vi "16Channels_savedata.vi"() -> ()   [LabVIEW 2020]
uses:
  Energy Meter/Labview Driver for S-Link (VISA).llb/Factor.ctl
  <vilib>/Utility/file.llb/Write Delimited Spreadsheet (string).vi
  <vilib>/Utility/file.llb/Write To Spreadsheet File (string).vi
  <vilib>/Utility/file.llb/Read Delimited Spreadsheet (DBL).vi
panel:
  out "Second Window Output":T1={"Status"=TRUE, "Indicator Color"=[], "Time"="", "Energy Value"=0.0, "Spectrometer Output"={array[3648 elements], array[3648 elements]}, "Energy stat"=TRUE}
  out "Program Status:":string="Program Stopped!"
  in  "Send 8":bool
  in  "Send 7":bool
  in  "Send 6":bool
  in  "Com Port 8":refnum<visa-resource-name>="COM27"
  in  "Com Port 7":refnum<visa-resource-name>="COM25"
  in  "Com Port 6":refnum<visa-resource-name>="COM23"
  in  "Save Next shot to File?":bool=TRUE
  in  "Com Port 5":refnum<visa-resource-name>="COM24"
  in  "Send 5":bool
  in  "Tab Control":T2(tab)=enum."Plots"
  out "Scale 8":dbl format="%.0e"
  out "Ch 08 Status":bool
  in  "Scale UP 8":bool
  in  "Scale Down 8":bool
  out "Measure 8":dbl format="%.3e"
  out "Scale 1":dbl=0.00031622776601683794 format="%.0e"
  out "Scale 2":dbl=0.00031622776601683794 format="%.0e"
  out "Ch 02 Status":bool
  out "Ch 01 Status":bool
  out "Scale 3":dbl=0.03162277660168379 format="%.0e"
  out "Scale 4":dbl=0.03162277660168379 format="%.0e"
  out "Ch 04 Status":bool
  out "Ch 03 Status":bool
  in  "Scale Down":bool
  in  "Scale UP 2":bool
  in  "Scale Down 2":bool
  in  "Scale UP":bool
  out "Measure 2":dbl format="%.3e"
  out "Measure 3":dbl format="%.3e"
  out "Measure 4":dbl format="%.3e"
  in  "Scale UP 3":bool
  in  "Scale Down 3":bool
  in  "Scale UP 4":bool
  in  "Scale Down 4":bool
  out "Scale 5":dbl=0.03162277660168379 format="%.0e"
  out "Scale 6":dbl=0.03162277660168379 format="%.0e"
  out "Ch 06 Status":bool
  out "Ch 05 Status":bool
  out "Measure 5":dbl format="%.3e"
  out "Measure 6":dbl format="%.3e"
  in  "Scale UP 5":bool
  in  "Scale Down 5":bool
  in  "Scale UP 6":bool
  in  "Scale Down 6":bool
  out "Measure 1":dbl format="%.3e"
  out "Scale 7":dbl format="%.0e"
  out "Ch 07 Status":bool
  in  "Scale UP 7":bool
  in  "Scale Down 7":bool
  out "Measure 7":dbl format="%.3e"
  in  "Scale UP 9":bool
  in  "Scale Down 9":bool
  in  "Scale UP 10":bool
  in  "Scale Down 10":bool
  out "Scale 9":dbl=0.03162277660168379 format="%.0e"
  out "Scale 10":dbl=0.03162277660168379 format="%.0e"
  out "Ch 09 Status":bool
  out "Ch 10 Status":bool
  out "Measure 9":dbl format="%.3e"
  out "Measure 10":dbl format="%.3e"
  out "Measure 11":dbl=0.00198 format="%.3e"
  out "Measure 12":dbl=0.001829 format="%.3e"
  in  "Scale UP 11":bool
  in  "Scale Down 11":bool
  in  "Scale UP 12":bool
  in  "Scale Down 12":bool
  out "Scale 11":dbl=0.0031622776601683794 format="%.0e"
  out "Scale 12":dbl=0.03162277660168379 format="%.0e"
  out "Ch 11 Status":bool
  out "Ch 12 Status":bool
  out "Scale 13":dbl format="%.0e"
  out "Scale 14":dbl format="%.0e"
  out "Ch 13 Status":bool
  out "Ch 14 Status":bool
  out "Scale 15":dbl=0.03162277660168379 format="%.0e"
  out "Scale 16":dbl=0.03162277660168379 format="%.0e"
  out "Ch 15 Status":bool
  out "Ch 16 Status":bool
  in  "Scale UP 13":bool
  in  "Scale Down 13":bool
  in  "Scale UP 14":bool
  in  "Scale Down 14":bool
  out "Measure 13":dbl=0.0004823 format="%.3e"
  out "Measure 14":dbl=1.44e-05 format="%.3e"
  in  "Scale UP 15":bool
  in  "Scale Down 15":bool
  in  "Scale UP 16":bool
  in  "Scale Down 16":bool
  out "Measure 15":dbl format="%.3e"
  out "Measure 16":dbl format="%.3e"
  out "Ch 1":dbl(graph)
  out "Ch 2":dbl(graph)
  out "Ch 3":dbl(graph)
  out "Ch 4":dbl(graph)
  out "Ch 5":dbl(graph)
  out "Ch 6":dbl(graph)=0.01011366
  out "Ch 7":dbl(graph)=0.0052277218000000006
  out "Ch 8":dbl(graph)=0.007128125500000001
  out "Ch 9":dbl(graph)=1.049625
  out "Ch 10":dbl(graph)=11.3826
  out "Ch 11":dbl(graph)=178.2
  out "Ch 12":dbl(graph)=0.001829
  out "Ch 13":dbl(graph)=591.068296
  out "Ch 14":dbl(graph)=1.44
  out "Ch 15":dbl(graph)
  out "Ch 16":dbl(graph)
  out "Ch 01 Status 2":bool=TRUE
  out "Ch 03 Status 2":bool=TRUE
  out "Ch 06 Status 2":bool=TRUE
  out "Ch 07 Status 2":bool=TRUE
  out "Ch 10 Status 2":bool=TRUE
  out "Ch 02 Status 2":bool=TRUE
  out "Ch 04 Status 2":bool=TRUE
  out "Ch 05 Status 2":bool=TRUE
  out "Ch 08 Status 2":bool=TRUE
  out "Ch 09 Status 2":bool=TRUE
  out "Ch 11 Status 2":bool=TRUE
  out "Ch 13 Status 2":bool=TRUE
  out "Ch 15 Status 2":bool=TRUE
  out "Ch 12 Status 2":bool=TRUE
  out "Ch 14 Status 2":bool=TRUE
  out "Ch 16 Status 2":bool=TRUE
  in  "Ch9 ON/OFF":bool=TRUE
  in  "Ch10 ON/OFF":bool=TRUE
  in  "Ch11 ON/OFF":bool=TRUE
  in  "Ch12 ON/OFF":bool=TRUE
  in  "Ch13 ON/OFF":bool=TRUE
  in  "Ch14 ON/OFF":bool=TRUE
  in  "C15 ON/OFF":bool=TRUE
  in  "Ch16 ON/OFF":bool=TRUE
  in  "Ch1 ON/OFF":bool=TRUE
  in  "Ch2 ON/OFF":bool=TRUE
  in  "Ch4 ON/OFF":bool=TRUE
  in  "Ch3 ON/OFF":bool=TRUE
  in  "Ch6 ON/OFF":bool=TRUE
  in  "Ch5 ON/OFF":bool=TRUE
  in  "Ch8 ON/OFF":bool=TRUE
  in  "Ch7 ON/OFF":bool=TRUE
  out "Trigger ch 10":bool=TRUE
  out "Trigger ch 9":bool=TRUE
  out "Trigger ch 8":bool=TRUE
  out "Trigger ch 7":bool
  out "Trigger ch 6":bool=TRUE
  out "Trigger ch 5":bool=TRUE
  out "Trigger ch 4":bool=TRUE
  out "Trigger ch 3":bool=TRUE
  out "Trigger ch 2":bool=TRUE
  out "Trigger ch 1":bool=TRUE
  in  "Threshold Green 1":dbl=9.0
  in  "Threshold Green 2":dbl=6.0
  out "Wavelength 7":i16
  out "Wavelength 6":i16=532
  out "Wavelength 5":i16=532
  out "Wavelength 4":i16=532
  out "Wavelength 3":i16=532
  out "Wavelength 2":i16=1064
  out "Wavelength 1":i16=1064
  out "Wavelength 8":i16
  in  "Factor 7":T3=642.7 caption="Factor1" format="%#_13g"
  in  "Factor 6":T3=470.0 caption="Factor1" format="%#_13g"
  in  "Factor 5":T3=470.0 caption="Factor1" format="%#_13g"
  in  "Factor 4":T3=486.0 caption="Factor1" format="%#_13g"
  in  "Factor 3":T3=3108.0 caption="Factor1" format="%#_13g"
  in  "Factor 2":T3=12595.0 caption="Factor1" format="%#_13g"
  in  "Factor 1":T3=8156.0 caption="Factor1" format="%#_13g"
  in  "Factor 8":T3=789.82 caption="Factor1" format="%#_13g"
  in  "Threshold IR 1":dbl=2.3
  in  "Threshold IR 2":dbl=2.0
  in  "Factor 9":T3=622.2 caption="Factor1" format="%#_13g"
  in  "Factor 10":T3=777.5 caption="Factor1" format="%#_13g"
  out "Wavelength 9":i16=532
  out "Wavelength 10":i16=532
  in  "Factor 11":T3=90.0 caption="Factor1" format="%#_13g"
  in  "Factor 12":T3=1.0 caption="Factor1" format="%#_13g"
  in  "Threshold 2nd stage 1":dbl=0.16
  in  "Threshold 2nd stage 2":dbl=0.12
  in  "Threshold 3rd stage 1":dbl=2.5
  in  "Threshold 3rd stage 2":dbl=2.0
  out "Trigger ch 11":bool
  out "Trigger ch 12":bool=TRUE
  out "Wavelength 11":i16=800
  out "Wavelength 12":i16=800
  out "Wavelength 13":i16
  out "Wavelength 14":i16
  out "Trigger ch 13":bool
  out "Trigger ch 14":bool
  out "Wavelength 15":i16=800
  out "Wavelength 16":i16=800
  out "Trigger ch 15":bool=TRUE
  out "Trigger ch 16":bool=TRUE
  in  "Threshold 1st stage 1":dbl=0.0013 format="%#_2e"
  in  "Threshold 1st stage 2":dbl=0.001 format="%#_2e"
  in  "Threshold quantaray stage 1":dbl=0.62
  in  "Threshold quantaray stage 2":dbl=0.58
  in  "Factor 13":T3=1225.52 caption="Factor1" format="%#_13g"
  in  "Factor 14":T3=100.0 caption="Factor1" format="%#_13g"
  in  "Factor 15":T3=1.0 caption="Factor1" format="%#_13g"
  in  "Factor a":T3=43958.0 caption="Factor1" format="%#_13g"
  in  "Threshold 4th stage 2":dbl=7.0
  in  "Threshold 4th stage 1":dbl=9.0
  in  "Threshold 5th stage 2":dbl
  in  "Threshold 5th stage 1":dbl
  in  "Factor b":T3=10193.0 caption="Factor1" format="%#_13g"
  in  "Factor c":T3=-0.3437 caption="Factor1" format="%#_13g"
  out "Path Spectrometer Folder":path=path "D:/Spectrometer/20220114"
  out "Path Spectrometer Data Old":path
  in  "Path Spectrometer Base":path=path "D:/Spectrometer"
  in  "Base Path":path=path "D:/Energy Meter"
  out "Folder":path=path "D:/Energy Meter/20220114"
  in  "Path SLAB #10":path=path "D:/Energy Meter/20220114/SLAB10.csv"
  in  "Path SLAB #9":path=path "D:/Energy Meter/20220114/SLAB9.csv"
  in  "Path SLAB #8":path=path "D:/Energy Meter/20220114/SLAB8.csv"
  in  "Path SLAB #7":path=path "D:/Energy Meter/20220114/SLAB7.csv"
  in  "Path SLAB #5":path=path "D:/Energy Meter/20220114/SLAB5.csv"
  in  "Path SLAB #4":path=path "D:/Energy Meter/20220114/SLAB4.csv"
  in  "Path SLAB #3":path=path "D:/Energy Meter/20220114/SLAB3.csv"
  in  "Path SLAB #2":path=path "D:/Energy Meter/20220114/SLAB2.csv"
  in  "Path Frontend #2":path=path "D:/Energy Meter/20220114/FrontEnd2.csv"
  in  "Path Frontend #1":path=path "D:/Energy Meter/20220114/FrontEnd1.csv"
  out "Date":string="20220114"
  out "Time":string="11:33:50.900"
  in  "Path 1st stage":path=path "D:/Energy Meter/20220114/1st_stage.csv"
  in  "Path 2nd stage":path=path "D:/Energy Meter/20220114/2nd_stage.csv"
  in  "Path 3rd stage":path=path "D:/Energy Meter/20220114/3rd_stage.csv"
  in  "Path 4th stage":path=path "D:/Energy Meter/20220114/4th_stage.csv"
  in  "Path 5th stage":path=path "D:/Energy Meter/20220114/5th_stage.csv"
  in  "Path quanta ray":path=path "D:/Energy Meter/20220114/quanta-ray.csv"
  in  "Send 4":bool
  in  "Com Port 4":refnum<visa-resource-name>="COM26"
  in  "Command":i32(ring)=22 items=["*RST", "*VER", "*CA1", "*CA2", "*SS1", "*SS2", "*SU1", "*SU2", "*SD1", "*SD2", "*CS1", "*CS2", "*AT1", "*AT2", "*AN1", "*AN2", "*PW1", "*PW2", "*TL1", "*TL2", "*ST1", "*ST2", "*ET1", "*ET2", "*EM1", "*EM2", "*SC1", "*SC2"]
  in  "Option":string="0"
  in  "Send 3":bool
  in  "Com Port 3":refnum<visa-resource-name>="COM20"
  in  "Send 2":bool
  in  "Stop Application":bool
  in  "Send":bool
  in  "Com Port 2":refnum<visa-resource-name>="COM22"
  in  "Com Port 1":refnum<visa-resource-name>="COM21"
  # "FrontEnd 1"
  # "SLAB 7"
  # "Quanta-Ray"
  # "FrontEnd 2"
  # "SLAB 9"
  # "1st Stage"
  # "SLAB 2"
  # "SLAB 10"
  # "4th Stage"
  # "SLAB 4"
  # "SLAB 8"
  # "5th Stage"
  # "SLAB 5"
  # "2nd Stage"
  # "SLAB 3"
  # "3rd Stage"
  # "FrontEnd #1"
  # "J"
  # "FrontEnd #2"
  # "J"
  # "Quanta-Ray"
  # "mJ"
  # "1st Stage"
  # "mJ"
  # "SLAB #2"
  # "SLAB #4"
  # "2nd Stage"
  # "3rd Stage"
  # "J"
  # "J"
  # "mJ"
  # "J"
  # "SLAB #3"
  # "SLAB #5"
  # "4th Stage"
  # "5th Stage"
  # "J"
  # "J"
  # "J"
  # "J"
  # "SLAB #7"
  # "SLAB #9"
  # "J"
  # "J"
  # "SLAB #8"
  # "SLAB #10"
  # "J"
  # "J"
  # "External\nTrigger"
  # "Wavelength"
  # "Energy Factor"
  # "Threshold 1\n(Warning)"
  # "Threshold 2\n(Bad)"
  # "Channel 01"
  # "IR"
  # "J"
  # "Com Port 1"
  # "Channel 02"
  # "Green"
  # "J"
  # "Channel 03"
  # "1st Stage"
  # "J"
  # "Com Port 2"
  # "Channel 04"
  # "2nd Stage"
  # "J"
  # "Channel 05"
  # "3rd Stage"
  # "J"
  # "Com Port 3"
  # "4th Stage"
  # "J"
  # "Channel 06"
  # "5th Stage"
  # "J"
  # "Channel 07"
  # "Com Port 4"
  # "Quanta-Ray"
  # "J"
  # "MUST USE THE FOLLOWING COMPORT SETTING! Otherwise the app will not save to proper files\n\nCom Port 1: COM21\nCom Port 2: COM22\nCom Port 3: COM20\nCom Port 4: COM26\nCom Port 5: COM24\nCom Port 6: COM23\nCom Port 7: COM25\nCom Port 8: COM27\n\nCOM20: Ch1- SLAB 5  Ch2 - SLAB 3  \nCOM21: Ch1- FrontEnd 1  Ch2- FrontEnd 2\nCOM22: Ch1- SLAB 2  Ch2 - SLAB 4\nCOM24: Ch1 - SLAB 10   Ch2 - SLAB 8\nCOM26: Ch1 - SLAB 7   Ch2 -SLAB 9\nCOM23: Ch1 - 2nd Stage  Ch2 - 3rd Stage\nCOM25: Ch1 - Quantaray  Ch2 - 1st Stage\nCOM27: Ch1 - 4th Stage  Ch2 - 5th Stage"
  # "Channel 08"
  # "Channel 09"
  # "Activate Channels"
  # "Com Port 5"
  # "Channel 10"
  # "Need to restart to change the status!"
  # "Ch09"
  # "Ch01"
  # "Ch09: SLAB #10\n\nCh10: SLAB #8\n\nCh11: 2nd Stage\n\nCh12: 3rd Stage\n\nCh13: Quanta-Ray\n\nCh14: 1st Stage\n\nCh15: 4th Stage\n\nCh16: 5th Stage"
  # "Ch01: FrontEnd #1 \n\nCh02: FrontEnd #2\n\nCh03: SLAB #2\n\nCh04: SLAB #4\n\nCh05: SLAB #5\n\nCh06: SLAB #3\n\nCh07: SLAB #7\n\nCh08: SLAB #9"
  # "OFF"
  # "ON"
  # "OFF"
  # "ON"
  # "Channel 11"
  # "Com Port 6"
  # "Ch10"
  # "Ch02"
  # "OFF"
  # "ON"
  # "OFF"
  # "ON"
  # "Channel 12"
  # "Ch11"
  # "Ch03"
  # "OFF"
  # "ON"
  # "OFF"
  # "ON"
  # "Channel 13"
  # "Ch12"
  # "Ch04"
  # "OFF"
  # "ON"
  # "OFF"
  # "ON"
  # "Com Port 7"
  # "Channel 14"
  # "Ch13"
  # "Ch05"
  # "OFF"
  # "ON"
  # "OFF"
  # "ON"
  # "Ch14"
  # "Channel 15"
  # "Ch06"
  # "OFF"
  # "ON"
  # "OFF"
  # "ON"
  # "Com Port 8"
  # "Ch15"
  # "Ch07"
  # "Channel 16"
  # "a"
  # "OFF"
  # "ON"
  # "OFF"
  # "ON"
  # "b"
  # "Ch16"
  # "Ch08"
  # "OFF"
  # "ON"
  # "OFF"
  # "ON"
  # "Polynominal Factor: ax^2+bx+c"
  # "c"
  # "Change base path before running the program!"
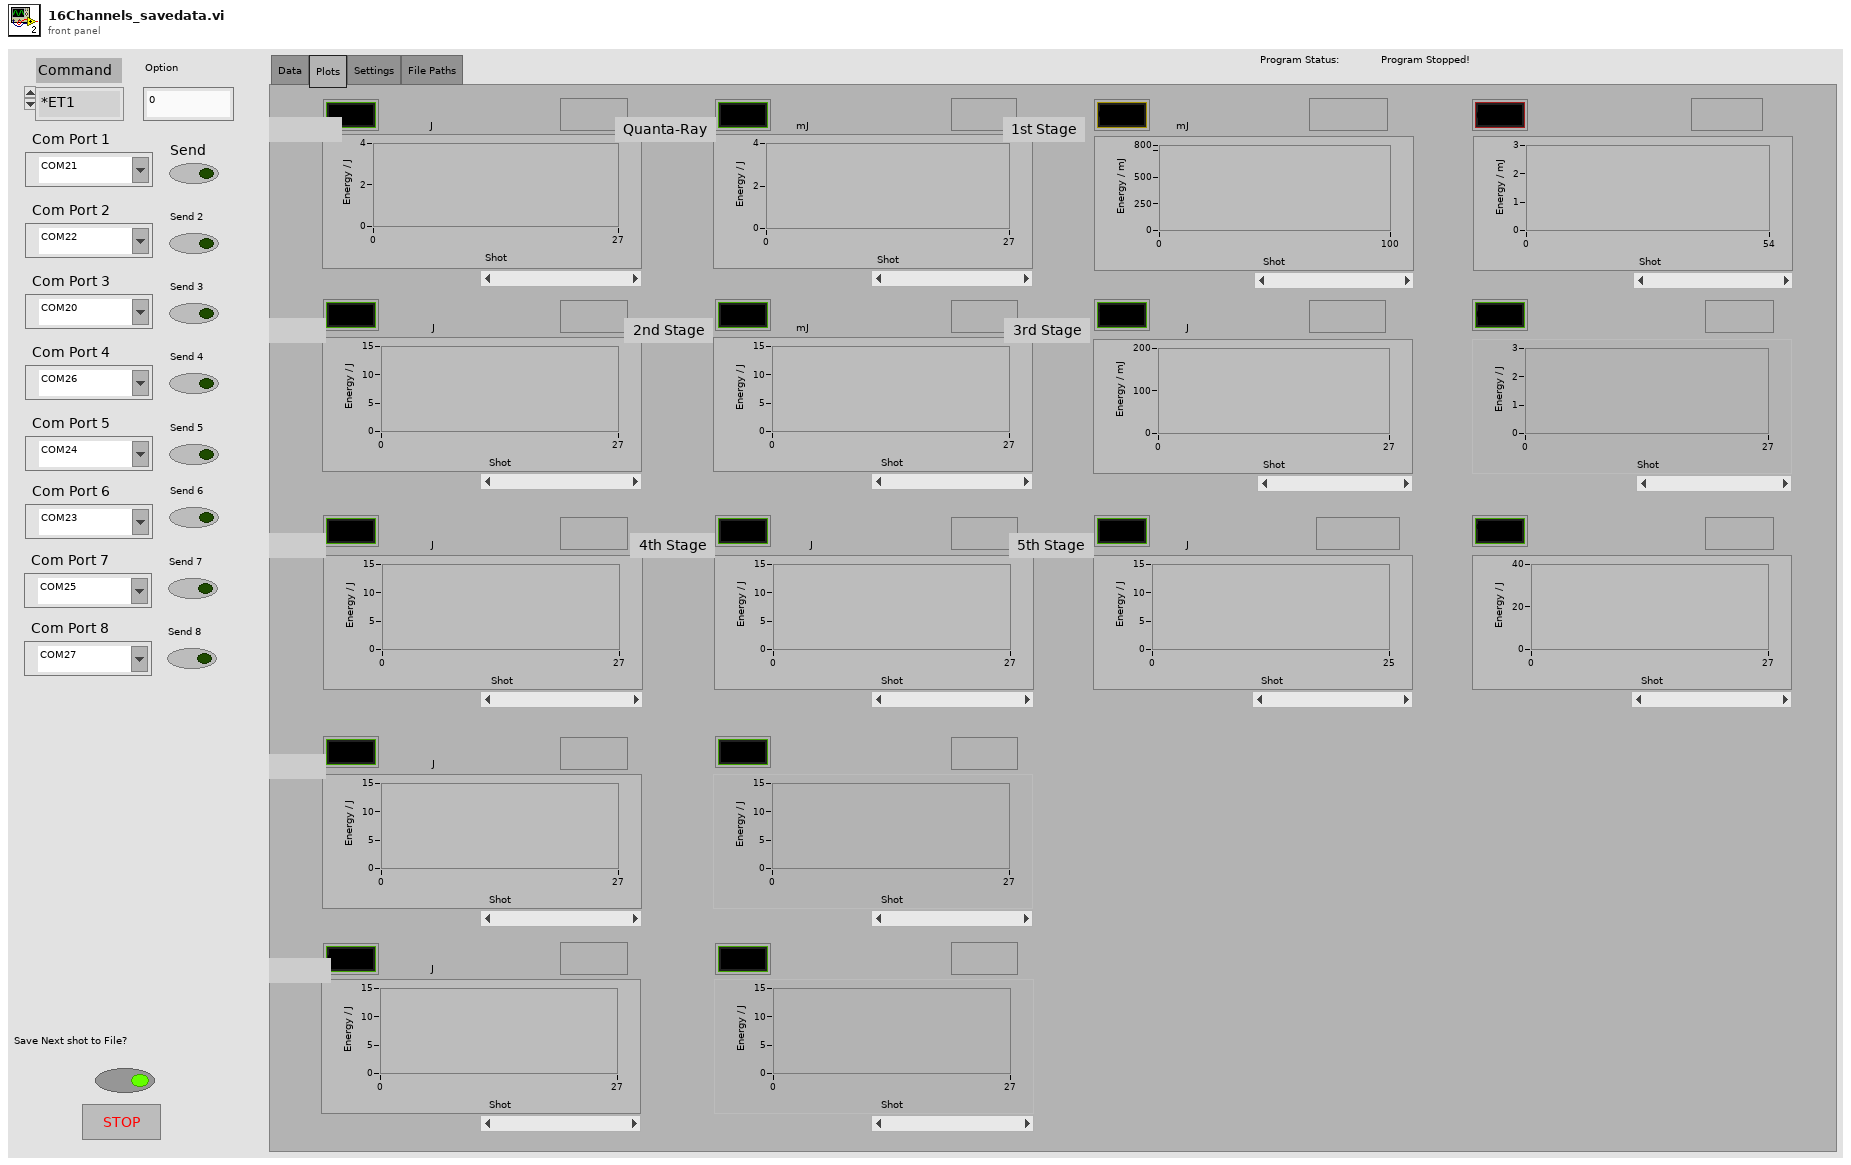
[diagram p1: front panel]
types:
  T1 = cluster{"Status":bool, "Indicator Color":cluster{u32, u32}[], "Time":string, "Energy Value":dbl, "Spectrometer Output":cluster{dbl[], dbl[]}, "Energy stat":bool}
  T2 = enum32{"Data", "Plots", "Settings", "File Paths"}
  T3 = typedef "Factor.ctl" = dbl
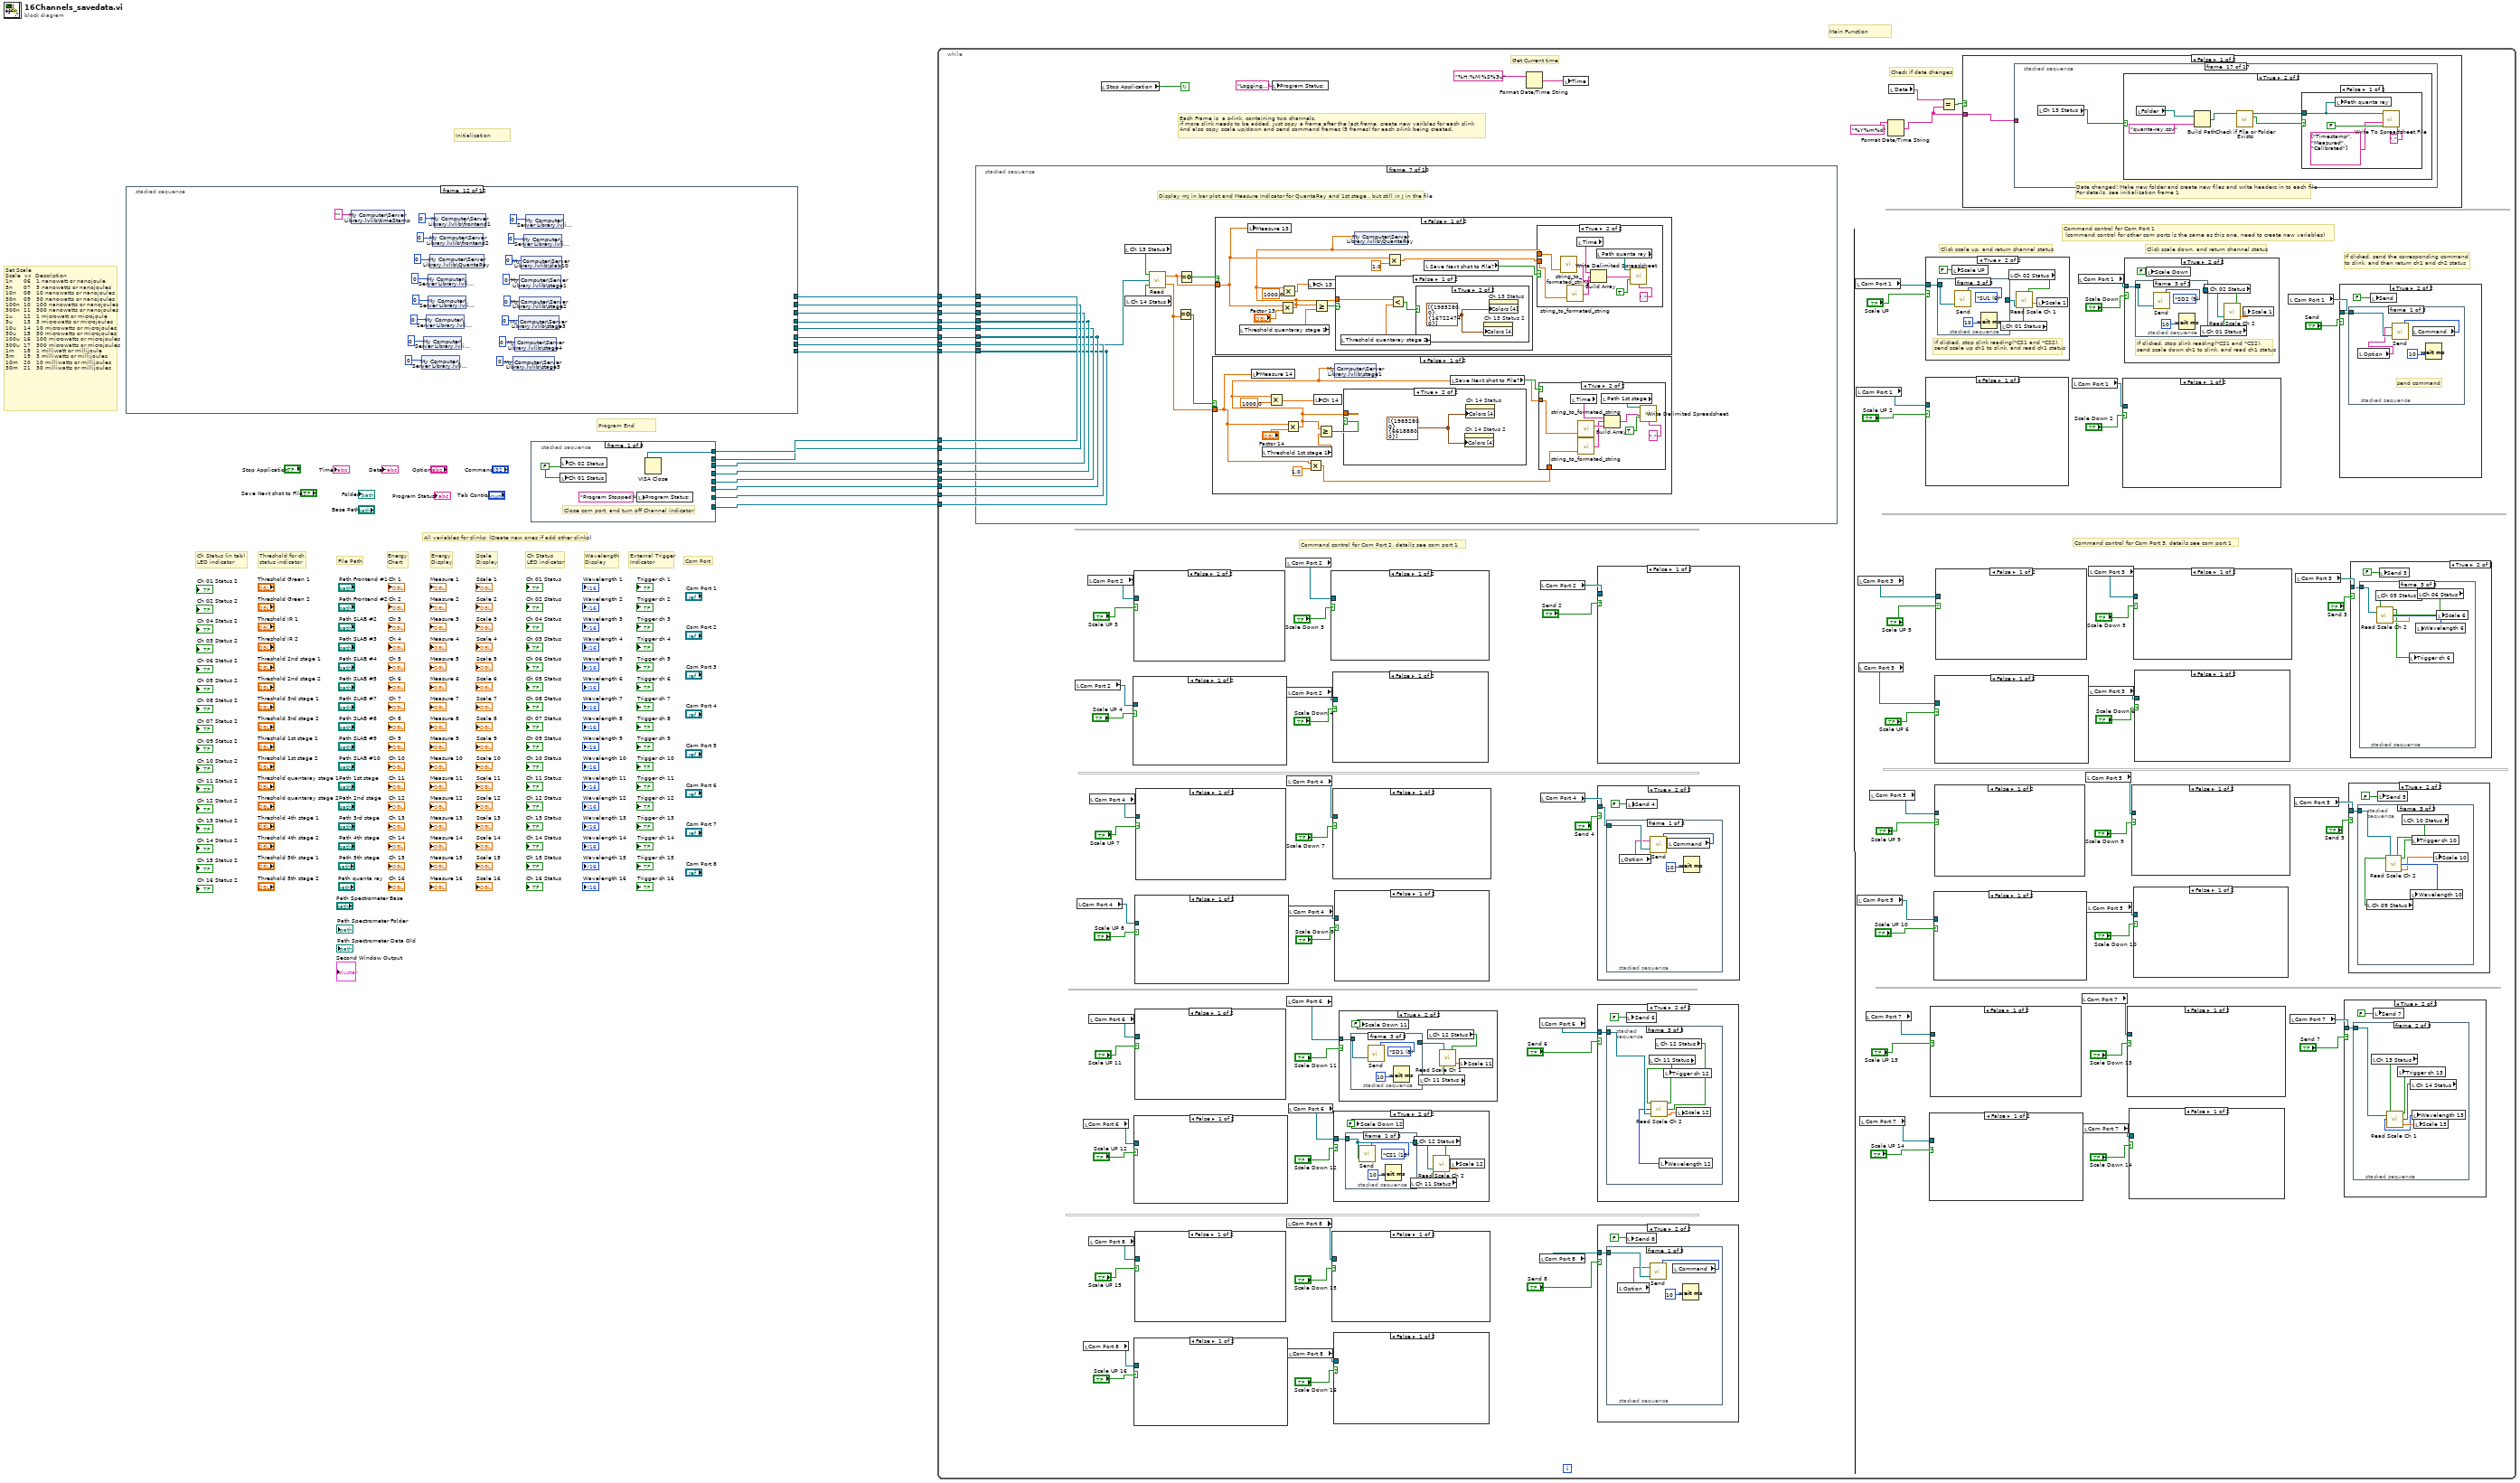
[diagram p0: block diagram]
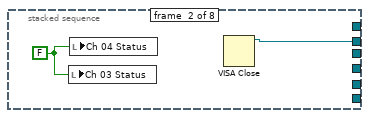
[diagram p2: hidden frame]
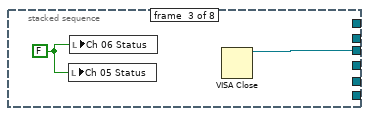
[diagram p3: hidden frame]
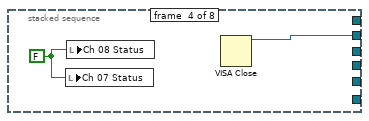
[diagram p4: hidden frame]
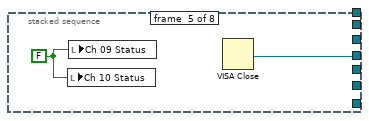
[diagram p5: hidden frame]
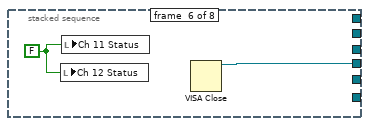
[diagram p6: hidden frame]
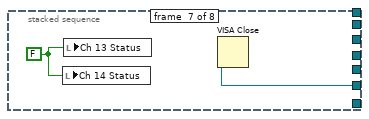
[diagram p7: hidden frame]
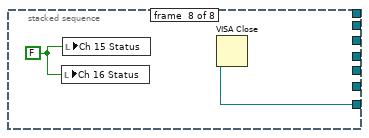
[diagram p8: hidden frame]
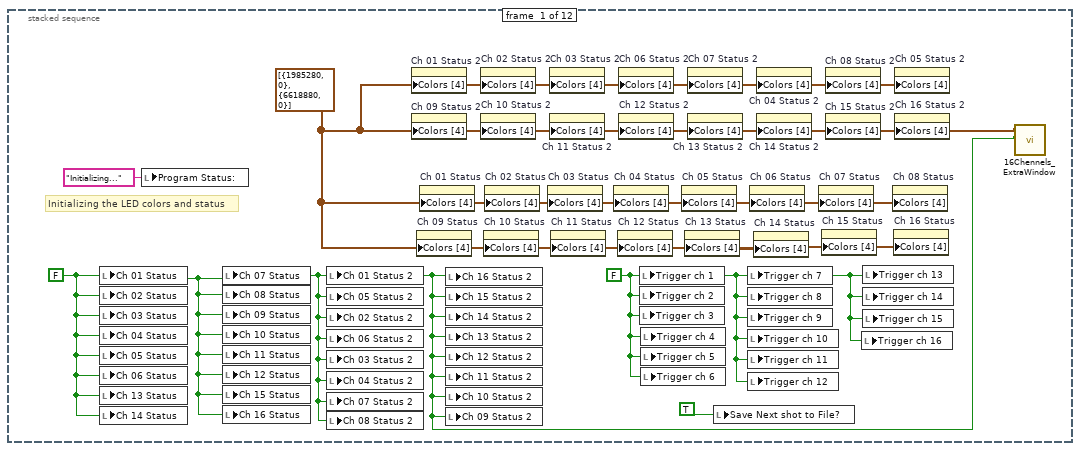
[diagram p9: hidden frame]
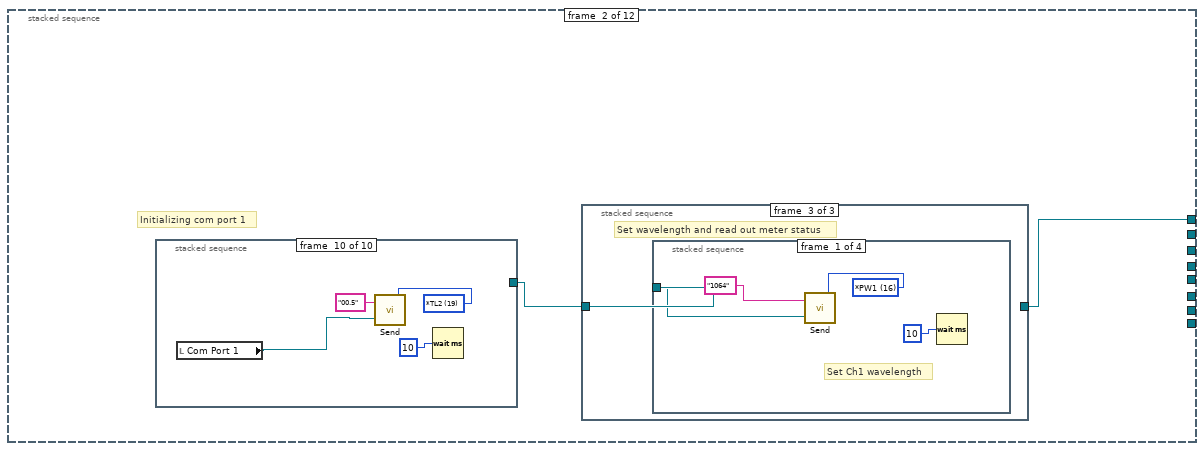
[diagram p10: hidden frame]
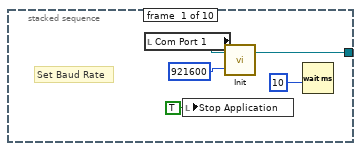
[diagram p11: hidden frame]
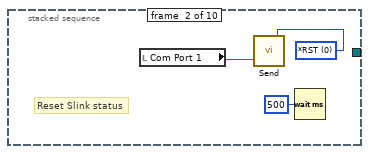
[diagram p12: hidden frame]
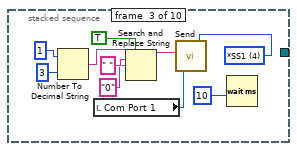
[diagram p13: hidden frame]
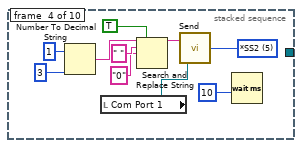
[diagram p14: hidden frame]
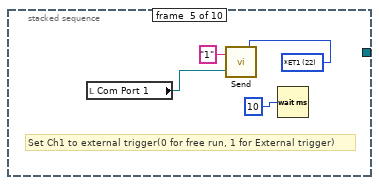
[diagram p15: hidden frame]
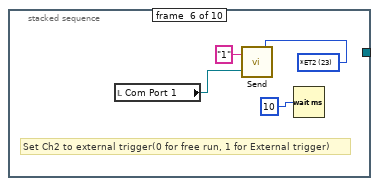
[diagram p16: hidden frame]
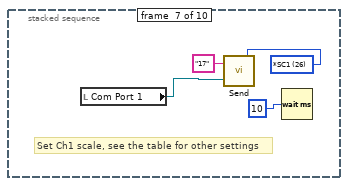
[diagram p17: hidden frame]
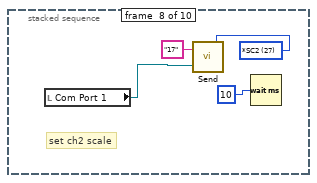
[diagram p18: hidden frame]
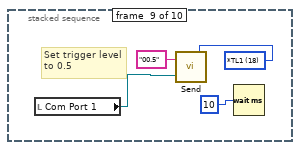
[diagram p19: hidden frame]
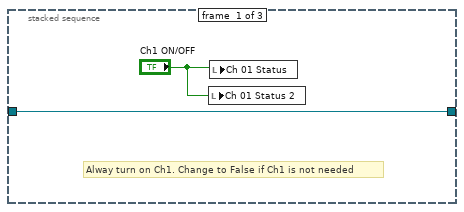
[diagram p20: hidden frame]
diagram:
  # "Ch Status (in tab) \nLED indicator"
  # "Com Port"
  # "Wavelength\nDisplay"
  # "Ch Status \nLED indicator"
  # "Scale \nDisplay"
  # "Energy\nDisplay"
  # "Energy\nChart"
  # "File Path"
  # "Threshold for ch\nstatus indicator"
  # "Main Function"
  # "All variables for slinks: (Create new ones if add other slinks)"
  # "Initialization"
  # "Program End"
  # "External Trigger\nIndicator"
  # "Set Scale\nScale  xx  Description\n1n      06   1 nanowatt or nanojoule\n3n      07   3 nanowatts or nanojoules\n10n    08   10 nanowatts or nanojoules\n30n    09   30 nanowatts or nanojoules\n100n  10   100 nanowatts or nanojoules\n300n  11   300 nanowatts or nanojoules\n1u      12   1 microwatt or microjoule\n3u      13   3 microwatts or microjoules\n10u    14   10 microwatts or microjoules\n30u    15   30 microwatts or microjoules\n100u  16   100 microwatts or microjoules\n300u  17   300 microwatts or microjoules\n1m     18   1 milliwatt or millijoule\n3m     19   3 milliwatts or millijoules\n10m   20   10 milliwatts or millijoules\n30m   21   30 milliwatts or millijoules"
  n1 = stacked-sequence {
    tunnel: [_ w23 _ _ _ _ _ _ _ _ _ _] -> w16
    tunnel: [_ _ w104 _ _ _ _ _ _ _ _ _] -> w14
    tunnel: [_ _ _ w185 _ _ _ _ _ _ _ _] -> w13
    tunnel: [_ _ _ _ w266 _ _ _ _ _ _ _] -> w12
    tunnel: [_ _ _ _ _ w338 _ _ _ _ _ _] -> w11
    tunnel: [_ _ _ _ _ _ w410 _ _ _ _ _] -> w10
    tunnel: [_ _ _ _ _ _ _ w483 _ _ _ _] -> w9
    tunnel: [_ _ _ _ _ _ _ _ w556 _ _ _] -> w8
    frame #0 {
      w19 = FALSE
      w18 = cluster{u32, u32}[] [{1985280, 0}, {6618880, 0}] ("Colors [4]")
      w17 = FALSE ("Ch 1 Status")
      # "Initializing the LED colors and status"
      n2 = local write "Ch 01 Status"(w17) -> ()
      n3 = local write "Ch 02 Status"(w17) -> ()
      n4 = local write "Ch 03 Status"(w17) -> ()
      n5 = local write "Ch 04 Status"(w17) -> ()
      n6 = local write "Ch 05 Status"(w17) -> ()
      n7 = local write "Ch 06 Status"(w17) -> ()
      n8 = local write "Ch 13 Status"(w17) -> ()
      n9 = local write "Ch 14 Status"(w17) -> ()
      n10 = local write "Program Status:"("Initializing..." ("Program Status")) -> ()
      n11 = local write "Ch 07 Status"(w17) -> ()
      n12 = local write "Ch 08 Status"(w17) -> ()
      n13 = local write "Ch 09 Status"(w17) -> ()
      n14 = local write "Ch 10 Status"(w17) -> ()
      n15 = local write "Ch 11 Status"(w17) -> ()
      n16 = local write "Ch 12 Status"(w17) -> ()
      n17 = local write "Ch 15 Status"(w17) -> ()
      n18 = local write "Ch 16 Status"(w17) -> ()
      n19 = local write "Ch 01 Status 2"(w17) -> ()
      n20 = local write "Ch 05 Status 2"(w17) -> ()
      n21 = local write "Ch 02 Status 2"(w17) -> ()
      n22 = local write "Ch 06 Status 2"(w17) -> ()
      n23 = local write "Ch 03 Status 2"(w17) -> ()
      n24 = local write "Ch 04 Status 2"(w17) -> ()
      n25 = local write "Ch 07 Status 2"(w17) -> ()
      n26 = local write "Ch 08 Status 2"(w17) -> ()
      n27 = property on="Ch 01 Status 2" class="Bool (strict)"("Colors [4]"=w18) -> ()  [unwired: 2 in, 2 out]
      n28 = property on="Ch 09 Status 2" class="Bool (strict)"("Colors [4]"=w18) -> ()  [unwired: 2 in, 2 out]
      n29 = property on="Ch 09 Status" class="Bool (strict)"("Colors [4]"=w18) -> ()  [unwired: 2 in, 2 out]
      n30 = property on="Ch 01 Status" class="Bool (strict)"("Colors [4]"=w18) -> ()  [unwired: 2 in, 2 out]
      n31 = local write "Ch 16 Status 2"(w17) -> ()
      n32 = local write "Ch 15 Status 2"(w17) -> ()
      n33 = local write "Ch 14 Status 2"(w17) -> ()
      n34 = local write "Ch 13 Status 2"(w17) -> ()
      n35 = local write "Ch 12 Status 2"(w17) -> ()
      n36 = local write "Ch 11 Status 2"(w17) -> ()
      n37 = local write "Ch 10 Status 2"(w17) -> ()
      n38 = local write "Ch 09 Status 2"(w17) -> ()
      n39 = property on="Ch 02 Status 2" class="Bool (strict)"("Colors [4]"=w18) -> ()  [unwired: 2 in, 2 out]
      n40 = property on="Ch 10 Status 2" class="Bool (strict)"("Colors [4]"=w18) -> ()  [unwired: 2 in, 2 out]
      n41 = property on="Ch 10 Status" class="Bool (strict)"("Colors [4]"=w18) -> ()  [unwired: 2 in, 2 out]
      n42 = property on="Ch 02 Status" class="Bool (strict)"("Colors [4]"=w18) -> ()  [unwired: 2 in, 2 out]
      n43 = property on="Ch 03 Status" class="Bool (strict)"("Colors [4]"=w18) -> ()  [unwired: 2 in, 2 out]
      n44 = property on="Ch 03 Status 2" class="Bool (strict)"("Colors [4]"=w18) -> ()  [unwired: 2 in, 2 out]
      n45 = property on="Ch 11 Status 2" class="Bool (strict)"("Colors [4]"=w18) -> ()  [unwired: 2 in, 2 out]
      n46 = property on="Ch 11 Status" class="Bool (strict)"("Colors [4]"=w18) -> ()  [unwired: 2 in, 2 out]
      n47 = property on="Ch 04 Status" class="Bool (strict)"("Colors [4]"=w18) -> ()  [unwired: 2 in, 2 out]
      n48 = property on="Ch 12 Status" class="Bool (strict)"("Colors [4]"=w18) -> ()  [unwired: 2 in, 2 out]
      n49 = property on="Ch 06 Status 2" class="Bool (strict)"("Colors [4]"=w18) -> ()  [unwired: 2 in, 2 out]
      n50 = property on="Ch 12 Status 2" class="Bool (strict)"("Colors [4]"=w18) -> ()  [unwired: 2 in, 2 out]
      n51 = local write "Trigger ch 1"(w19) -> ()
      n52 = local write "Trigger ch 2"(w19) -> ()
      n53 = local write "Trigger ch 3"(w19) -> ()
      n54 = local write "Trigger ch 4"(w19) -> ()
      n55 = local write "Trigger ch 5"(w19) -> ()
      n56 = local write "Trigger ch 6"(w19) -> ()
      n57 = property on="Ch 05 Status" class="Bool (strict)"("Colors [4]"=w18) -> ()  [unwired: 2 in, 2 out]
      n58 = property on="Ch 13 Status" class="Bool (strict)"("Colors [4]"=w18) -> ()  [unwired: 2 in, 2 out]
      n59 = property on="Ch 07 Status 2" class="Bool (strict)"("Colors [4]"=w18) -> ()  [unwired: 2 in, 2 out]
      n60 = property on="Ch 13 Status 2" class="Bool (strict)"("Colors [4]"=w18) -> ()  [unwired: 2 in, 2 out]
      n61 = local write "Save Next shot to File?"(TRUE) -> ()
      n62 = local write "Trigger ch 7"(w19) -> ()
      n63 = local write "Trigger ch 8"(w19) -> ()
      n64 = local write "Trigger ch 9"(w19) -> ()
      n65 = local write "Trigger ch 10"(w19) -> ()
      n66 = local write "Trigger ch 11"(w19) -> ()
      n67 = local write "Trigger ch 12"(w19) -> ()
      n68 = property on="Ch 06 Status" class="Bool (strict)"("Colors [4]"=w18) -> ()  [unwired: 2 in, 2 out]
      n69 = property on="Ch 14 Status" class="Bool (strict)"("Colors [4]"=w18) -> ()  [unwired: 2 in, 2 out]
      n70 = property on="Ch 04 Status 2" class="Bool (strict)"("Colors [4]"=w18) -> ()  [unwired: 2 in, 2 out]
      n71 = property on="Ch 14 Status 2" class="Bool (strict)"("Colors [4]"=w18) -> ()  [unwired: 2 in, 2 out]
      n72 = property on="Ch 07 Status" class="Bool (strict)"("Colors [4]"=w18) -> ()  [unwired: 2 in, 2 out]
      n73 = property on="Ch 15 Status" class="Bool (strict)"("Colors [4]"=w18) -> ()  [unwired: 2 in, 2 out]
      n74 = property on="Ch 08 Status 2" class="Bool (strict)"("Colors [4]"=w18) -> ()  [unwired: 2 in, 2 out]
      n75 = property on="Ch 15 Status 2" class="Bool (strict)"("Colors [4]"=w18) -> ()  [unwired: 2 in, 2 out]
      n76 = local write "Trigger ch 16"(w19) -> ()
      n77 = local write "Trigger ch 13"(w19) -> ()
      n78 = local write "Trigger ch 14"(w19) -> ()
      n79 = local write "Trigger ch 15"(w19) -> ()
      n80 = property on="Ch 08 Status" class="Bool (strict)"("Colors [4]"=w18) -> ()  [unwired: 2 in, 2 out]
      n81 = property on="Ch 16 Status" class="Bool (strict)"("Colors [4]"=w18) -> ()  [unwired: 2 in, 2 out]
      n82 = property on="Ch 05 Status 2" class="Bool (strict)"("Colors [4]"=w18) -> ()  [unwired: 2 in, 2 out]
      n83 = property on="Ch 16 Status 2" class="Bool (strict)"("Colors [4]"=w18) -> ()  [unwired: 2 in, 2 out]
      n84 = call "16Chennels_ExtraWindow.vi"("Ch 16 Status"=w17, "Colors [4]"=w18) -> ()  [unwired: 8 in]
    }
    frame #1 {
      # "Initializing com port 1"
      n85 = stacked-sequence {
        tunnel: [w24 _ _ _ _ _ _ _ _ _] -> w22
        frame #0 {
          # "Set Baud Rate"
          n86 = local read "Com Port 1"() -> (w24:refnum<visa-resource-name>)
          n87 = local write "Stop Application"(TRUE ("Stop programme")) -> ()
          n88 = call "Init.vi"("Baud Rate 2"=u32 921600 ("Baud Rate 3"), "# Port"=w24) -> ()  [unwired: 1 in]
          n89 = Wait (ms)(milliseconds to wait=10) -> ()  [unwired: 1 out]
        }
        frame #1 {
          w29 = 0 items=["*RST", "*VER", "*CA1", "*CA2", "*SS100", "*SS200", "*SU1", "*SU2", "*SD1", "*SD2", "*CS1", "*CS2", "*AT1", "*AT2", "*AN1", "*AN2", "*PW1", "*PW2", "*TL1", "*TL2", "*ST1", "*ST2", "*ET1", "*ET2", "*EM1", "*EM2", "*SC1", "*SC2"] ("string to write")
          # "Reset Slink status"
          n90 = local read "Com Port 1"() -> (w30:refnum<visa-resource-name>)
          n91 = call "Send.vi"("string to write"=w29, "port number"=w30) -> ()  [unwired: 1 in]
          n92 = Wait (ms)(milliseconds to wait=500) -> ()  [unwired: 1 out]
        }
        frame #2 {
          w37 = 4 items=["*RST", "*VER", "*CA1", "*CA2", "*SS1", "*SS2", "*SU1", "*SU2", "*SD1", "*SD2", "*CS1", "*CS2", "*AT1", "*AT2", "*AN1", "*AN2", "*PW1", "*PW2", "*TL1", "*TL2", "*ST1", "*ST2", "*ET1", "*ET2", "*EM1", "*EM2", "*SC1", "*SC2"] ("string to write")
          n93 = Number To Decimal String(number=1, width (-)=i16 3) -> (decimal integer string=w32:string)
          n94 = local read "Com Port 1"() -> (w39:refnum<visa-resource-name>)
          n95 = Search and Replace String(replace all?=TRUE ("replace all? (F)"), input string=w32, search string=" ", replace string="0" ("replace string (\"\")")) -> (result string=w33:string)  [unwired: 4 in, 3 out]
          n96 = call "Send.vi"("string to write"=w37, "port number"=w39, "Option"=w33) -> ()
          n97 = Wait (ms)(milliseconds to wait=10) -> ()  [unwired: 1 out]
        }
        frame #3 {
          w47 = 5 items=["*RST", "*VER", "*CA1", "*CA2", "*SS1", "*SS2", "*SU1", "*SU2", "*SD1", "*SD2", "*CS1", "*CS2", "*AT1", "*AT2", "*AN1", "*AN2", "*PW1", "*PW2", "*TL1", "*TL2", "*ST1", "*ST2", "*ET1", "*ET2", "*EM1", "*EM2", "*SC1", "*SC2"] ("string to write")
          n98 = Number To Decimal String(number=1, width (-)=i16 3) -> (decimal integer string=w46:string)
          n99 = local read "Com Port 1"() -> (w49:refnum<visa-resource-name>)
          n100 = Search and Replace String(replace all?=TRUE ("replace all? (F)"), input string=w46, search string=" ", replace string="0" ("replace string (\"\")")) -> (result string=w42:string)  [unwired: 4 in, 3 out]
          n101 = call "Send.vi"("string to write"=w47, "port number"=w49, "Option"=w42) -> ()
          n102 = Wait (ms)(milliseconds to wait=10) -> ()  [unwired: 1 out]
        }
        frame #4 {
          w53 = 22 items=["*RST", "*VER", "*CA1", "*CA2", "*SS1", "*SS2", "*SU1", "*SU2", "*SD1", "*SD2", "*CS1", "*CS2", "*AT1", "*AT2", "*AN1", "*AN2", "*PW1", "*PW2", "*TL1", "*TL2", "*ST1", "*ST2", "*ET1", "*ET2", "*EM1", "*EM2", "*SC1", "*SC2"] ("string to write")
          # "Set Ch1 to external trigger(0 for free run, 1 for External trigger)"
          n103 = local read "Com Port 1"() -> (w51:refnum<visa-resource-name>)
          n104 = call "Send.vi"("string to write"=w53, "port number"=w51, "Option"="1") -> ()
          n105 = Wait (ms)(milliseconds to wait=10) -> ()  [unwired: 1 out]
        }
        frame #5 {
          w57 = 23 items=["*RST", "*VER", "*CA1", "*CA2", "*SS1", "*SS2", "*SU1", "*SU2", "*SD1", "*SD2", "*CS1", "*CS2", "*AT1", "*AT2", "*AN1", "*AN2", "*PW1", "*PW2", "*TL1", "*TL2", "*ST1", "*ST2", "*ET1", "*ET2", "*EM1", "*EM2", "*SC1", "*SC2"] ("string to write")
          # "Set Ch2 to external trigger(0 for free run, 1 for External trigger)"
          n106 = local read "Com Port 1"() -> (w55:refnum<visa-resource-name>)
          n107 = call "Send.vi"("string to write"=w57, "port number"=w55, "Option"="1") -> ()
          n108 = Wait (ms)(milliseconds to wait=10) -> ()  [unwired: 1 out]
        }
        frame #6 {
          w61 = 26 items=["*RST", "*VER", "*CA1", "*CA2", "*SS1", "*SS2", "*SU1", "*SU2", "*SD1", "*SD2", "*CS1", "*CS2", "*AT1", "*AT2", "*AN1", "*AN2", "*PW1", "*PW2", "*TL1", "*TL2", "*ST1", "*ST2", "*ET1", "*ET2", "*EM1", "*EM2", "*SC1", "*SC2"] ("string to write")
          # "Set Ch1 scale, see the table for other settings"
          n109 = local read "Com Port 1"() -> (w59:refnum<visa-resource-name>)
          n110 = call "Send.vi"("string to write"=w61, "port number"=w59, "Option"="17") -> ()
          n111 = Wait (ms)(milliseconds to wait=10) -> ()  [unwired: 1 out]
        }
        frame #7 {
          w65 = 27 items=["*RST", "*VER", "*CA1", "*CA2", "*SS1", "*SS2", "*SU1", "*SU2", "*SD1", "*SD2", "*CS1", "*CS2", "*AT1", "*AT2", "*AN1", "*AN2", "*PW1", "*PW2", "*TL1", "*TL2", "*ST1", "*ST2", "*ET1", "*ET2", "*EM1", "*EM2", "*SC1", "*SC2"] ("string to write")
          # "set ch2 scale"
          n112 = local read "Com Port 1"() -> (w63:refnum<visa-resource-name>)
          n113 = call "Send.vi"("string to write"=w65, "port number"=w63, "Option"="17") -> ()
          n114 = Wait (ms)(milliseconds to wait=10) -> ()  [unwired: 1 out]
        }
        frame #8 {
          w69 = 18 items=["*RST", "*VER", "*CA1", "*CA2", "*SS1", "*SS2", "*SU1", "*SU2", "*SD1", "*SD2", "*CS1", "*CS2", "*AT1", "*AT2", "*AN1", "*AN2", "*PW1", "*PW2", "*TL1", "*TL2", "*ST1", "*ST2", "*ET1", "*ET2", "*EM1", "*EM2", "*SC1", "*SC2"] ("string to write")
          # "Set trigger level\nto 0.5"
          n115 = local read "Com Port 1"() -> (w68:refnum<visa-resource-name>)
          n116 = call "Send.vi"("string to write"=w69, "port number"=w68, "Option"="00.5") -> ()
          n117 = Wait (ms)(milliseconds to wait=10) -> ()  [unwired: 1 out]
        }
        frame #9 {
          w73 = 19 items=["*RST", "*VER", "*CA1", "*CA2", "*SS1", "*SS2", "*SU1", "*SU2", "*SD1", "*SD2", "*CS1", "*CS2", "*AT1", "*AT2", "*AN1", "*AN2", "*PW1", "*PW2", "*TL1", "*TL2", "*ST1", "*ST2", "*ET1", "*ET2", "*EM1", "*EM2", "*SC1", "*SC2"] ("string to write")
          n118 = local read "Com Port 1"() -> (w71:refnum<visa-resource-name>)
          n119 = call "Send.vi"("string to write"=w73, "port number"=w71, "Option"="00.5") -> ()
          n120 = Wait (ms)(milliseconds to wait=10) -> ()  [unwired: 1 out]
        }
      }
      n121 = stacked-sequence {
        tunnel: w22 -> [w76 _ w78]
        tunnel: [w76 _ _] -> w23
        frame #0 {
          # "Alway turn on Ch1. Change to False if Ch1 is not needed"
          n122 = local write "Ch 01 Status 2"("Ch1 ON/OFF") -> ()
          n123 = local write "Ch 01 Status"("Ch1 ON/OFF") -> ()
        }
        frame #1 {
          # "Alway turn on Ch2. Change to False if Ch1 is not needed"
          n124 = local write "Ch 02 Status 2"("Ch2 ON/OFF") -> ()
          n125 = local write "Ch 02 Status"("Ch2 ON/OFF") -> ()
        }
        frame #2 {
          # "Set wavelength and read out meter status"
          n126 = stacked-sequence {
            tunnel: w78 -> [w80 w84 w92 w96]
            frame #0 {
              w82 = 16 items=["*RST", "*VER", "*CA1", "*CA2", "*SS1", "*SS2", "*SU1", "*SU2", "*SD1", "*SD2", "*CS1", "*CS2", "*AT1", "*AT2", "*AN1", "*AN2", "*PW1", "*PW2", "*TL1", "*TL2", "*ST1", "*ST2", "*ET1", "*ET2", "*EM1", "*EM2", "*SC1", "*SC2"] ("string to write")
              # "Set Ch1 wavelength"
              n127 = call "Send.vi"("string to write"=w82, "port number"=w80, "Option"="1064") -> ()
              n128 = Wait (ms)(milliseconds to wait=10) -> ()  [unwired: 1 out]
            }
            frame #1 {
              # "read out ch1 status"
              n129 = local read "Ch 01 Status"() -> (w83:bool)
              n130 = case shown="True" w83 {
                tunnel: w84 -> [_ w90]
                frame False {
                }
                frame True {
                  n131 = local read "Ch 02 Status"() -> (w86:bool)
                  n132 = local read "Ch 01 Status"() -> (w89:bool)
                  n133 = call "Read Scale Ch 1.vi"("Ch2"=w86, "Com Port"=w90, "Ch 1"=w89) -> ("Scale 1Ch"=w87:dbl, "Trigger Status Ch1"=w85:bool, "Wavelength"=w88:u32)
                  n134 = local write "Trigger ch 1"(w85) -> ()
                  n135 = local write "Wavelength 1"(w88) -> ()
                  n136 = local write "Scale 1"(w87) -> ()
                }
              }
            }
            frame #2 {
              w94 = 17 items=["*RST", "*VER", "*CA1", "*CA2", "*SS1", "*SS2", "*SU1", "*SU2", "*SD1", "*SD2", "*CS1", "*CS2", "*AT1", "*AT2", "*AN1", "*AN2", "*PW1", "*PW2", "*TL1", "*TL2", "*ST1", "*ST2", "*ET1", "*ET2", "*EM1", "*EM2", "*SC1", "*SC2"] ("string to write")
              # "set ch2 wavelength"
              n137 = call "Send.vi"("string to write"=w94, "port number"=w92, "Option"="1064") -> ()
              n138 = Wait (ms)(milliseconds to wait=10) -> ()  [unwired: 1 out]
            }
            frame #3 {
              # "read out ch2 status"
              n139 = local read "Ch 02 Status"() -> (w95:bool)
              n140 = case shown="True" w95 {
                tunnel: w96 -> [_ w102]
                frame False {
                }
                frame True {
                  n141 = local read "Ch 01 Status"() -> (w100:bool)
                  n142 = local read "Ch 02 Status"() -> (w99:bool)
                  n143 = call "Read Scale Ch 2.vi"("Ch 2"=w99, "Com Port"=w102, "Ch1"=w100) -> ("Scale Ch2"=w101:dbl, "External Trigger Ch2"=w97:bool, "Wavelength"=w98:u32)
                  n144 = local write "Wavelength 2"(w98) -> ()
                  n145 = local write "Trigger ch 2"(w97) -> ()
                  n146 = local write "Scale 2"(w101) -> ()
                }
              }
            }
          }
        }
      }
    }
    frame #2 {
      # "See frame 2 for explanations"
      # "Initializing com port 2"
      n147 = stacked-sequence {
        tunnel: [w105 _ _ _ _ _ _ _ _ _] -> w103
        frame #0 {
          n148 = local read "Com Port 2"() -> (w105:refnum<visa-resource-name>)
          n149 = local write "Stop Application"(TRUE ("Stop programme")) -> ()
          n150 = call "Init.vi"("Baud Rate 2"=u32 921600 ("Baud Rate 3"), "# Port"=w105) -> ()  [unwired: 1 in]
          n151 = Wait (ms)(milliseconds to wait=10) -> ()  [unwired: 1 out]
        }
        frame #1 {
          w110 = 0 items=["*RST", "*VER", "*CA1", "*CA2", "*SS100", "*SS200", "*SU1", "*SU2", "*SD1", "*SD2", "*CS1", "*CS2", "*AT1", "*AT2", "*AN1", "*AN2", "*PW1", "*PW2", "*TL1", "*TL2", "*ST1", "*ST2", "*ET1", "*ET2", "*EM1", "*EM2", "*SC1", "*SC2"] ("string to write")
          n152 = local read "Com Port 2"() -> (w111:refnum<visa-resource-name>)
          n153 = call "Send.vi"("string to write"=w110, "port number"=w111) -> ()  [unwired: 1 in]
          n154 = Wait (ms)(milliseconds to wait=500) -> ()  [unwired: 1 out]
        }
        frame #2 {
          w118 = 4 items=["*RST", "*VER", "*CA1", "*CA2", "*SS1", "*SS2", "*SU1", "*SU2", "*SD1", "*SD2", "*CS1", "*CS2", "*AT1", "*AT2", "*AN1", "*AN2", "*PW1", "*PW2", "*TL1", "*TL2", "*ST1", "*ST2", "*ET1", "*ET2", "*EM1", "*EM2", "*SC1", "*SC2"] ("string to write")
          n155 = Number To Decimal String(number=1, width (-)=i16 3) -> (decimal integer string=w113:string)
          n156 = local read "Com Port 2"() -> (w120:refnum<visa-resource-name>)
          n157 = Search and Replace String(replace all?=TRUE ("replace all? (F)"), input string=w113, search string=" ", replace string="0" ("replace string (\"\")")) -> (result string=w114:string)  [unwired: 4 in, 3 out]
          n158 = call "Send.vi"("string to write"=w118, "port number"=w120, "Option"=w114) -> ()
          n159 = Wait (ms)(milliseconds to wait=10) -> ()  [unwired: 1 out]
        }
        frame #3 {
          w128 = 5 items=["*RST", "*VER", "*CA1", "*CA2", "*SS1", "*SS2", "*SU1", "*SU2", "*SD1", "*SD2", "*CS1", "*CS2", "*AT1", "*AT2", "*AN1", "*AN2", "*PW1", "*PW2", "*TL1", "*TL2", "*ST1", "*ST2", "*ET1", "*ET2", "*EM1", "*EM2", "*SC1", "*SC2"] ("string to write")
          n160 = Number To Decimal String(number=1, width (-)=i16 3) -> (decimal integer string=w127:string)
          n161 = local read "Com Port 2"() -> (w130:refnum<visa-resource-name>)
          n162 = Search and Replace String(replace all?=TRUE ("replace all? (F)"), input string=w127, search string=" ", replace string="0" ("replace string (\"\")")) -> (result string=w123:string)  [unwired: 4 in, 3 out]
          n163 = call "Send.vi"("string to write"=w128, "port number"=w130, "Option"=w123) -> ()
          n164 = Wait (ms)(milliseconds to wait=10) -> ()  [unwired: 1 out]
        }
        frame #4 {
          w134 = 22 items=["*RST", "*VER", "*CA1", "*CA2", "*SS1", "*SS2", "*SU1", "*SU2", "*SD1", "*SD2", "*CS1", "*CS2", "*AT1", "*AT2", "*AN1", "*AN2", "*PW1", "*PW2", "*TL1", "*TL2", "*ST1", "*ST2", "*ET1", "*ET2", "*EM1", "*EM2", "*SC1", "*SC2"] ("string to write")
          n165 = local read "Com Port 2"() -> (w132:refnum<visa-resource-name>)
          n166 = call "Send.vi"("string to write"=w134, "port number"=w132, "Option"="1") -> ()
          n167 = Wait (ms)(milliseconds to wait=10) -> ()  [unwired: 1 out]
        }
        frame #5 {
          w138 = 23 items=["*RST", "*VER", "*CA1", "*CA2", "*SS1", "*SS2", "*SU1", "*SU2", "*SD1", "*SD2", "*CS1", "*CS2", "*AT1", "*AT2", "*AN1", "*AN2", "*PW1", "*PW2", "*TL1", "*TL2", "*ST1", "*ST2", "*ET1", "*ET2", "*EM1", "*EM2", "*SC1", "*SC2"] ("string to write")
          n168 = local read "Com Port 2"() -> (w136:refnum<visa-resource-name>)
          n169 = call "Send.vi"("string to write"=w138, "port number"=w136, "Option"="1") -> ()
          n170 = Wait (ms)(milliseconds to wait=10) -> ()  [unwired: 1 out]
        }
        frame #6 {
          w142 = 26 items=["*RST", "*VER", "*CA1", "*CA2", "*SS1", "*SS2", "*SU1", "*SU2", "*SD1", "*SD2", "*CS1", "*CS2", "*AT1", "*AT2", "*AN1", "*AN2", "*PW1", "*PW2", "*TL1", "*TL2", "*ST1", "*ST2", "*ET1", "*ET2", "*EM1", "*EM2", "*SC1", "*SC2"] ("string to write")
          n171 = local read "Com Port 2"() -> (w141:refnum<visa-resource-name>)
          n172 = call "Send.vi"("string to write"=w142, "port number"=w141, "Option"="21") -> ()
          n173 = Wait (ms)(milliseconds to wait=10) -> ()  [unwired: 1 out]
        }
        frame #7 {
          w146 = 27 items=["*RST", "*VER", "*CA1", "*CA2", "*SS1", "*SS2", "*SU1", "*SU2", "*SD1", "*SD2", "*CS1", "*CS2", "*AT1", "*AT2", "*AN1", "*AN2", "*PW1", "*PW2", "*TL1", "*TL2", "*ST1", "*ST2", "*ET1", "*ET2", "*EM1", "*EM2", "*SC1", "*SC2"] ("string to write")
          n174 = local read "Com Port 2"() -> (w144:refnum<visa-resource-name>)
          n175 = call "Send.vi"("string to write"=w146, "port number"=w144, "Option"="21") -> ()
          n176 = Wait (ms)(milliseconds to wait=10) -> ()  [unwired: 1 out]
        }
        frame #8 {
          w150 = 18 items=["*RST", "*VER", "*CA1", "*CA2", "*SS1", "*SS2", "*SU1", "*SU2", "*SD1", "*SD2", "*CS1", "*CS2", "*AT1", "*AT2", "*AN1", "*AN2", "*PW1", "*PW2", "*TL1", "*TL2", "*ST1", "*ST2", "*ET1", "*ET2", "*EM1", "*EM2", "*SC1", "*SC2"] ("string to write")
          n177 = local read "Com Port 2"() -> (w148:refnum<visa-resource-name>)
          n178 = call "Send.vi"("string to write"=w150, "port number"=w148, "Option"="00.5") -> ()
          n179 = Wait (ms)(milliseconds to wait=10) -> ()  [unwired: 1 out]
        }
        frame #9 {
          w154 = 19 items=["*RST", "*VER", "*CA1", "*CA2", "*SS1", "*SS2", "*SU1", "*SU2", "*SD1", "*SD2", "*CS1", "*CS2", "*AT1", "*AT2", "*AN1", "*AN2", "*PW1", "*PW2", "*TL1", "*TL2", "*ST1", "*ST2", "*ET1", "*ET2", "*EM1", "*EM2", "*SC1", "*SC2"] ("string to write")
          n180 = local read "Com Port 2"() -> (w152:refnum<visa-resource-name>)
          n181 = call "Send.vi"("string to write"=w154, "port number"=w152, "Option"="00.5") -> ()
          n182 = Wait (ms)(milliseconds to wait=10) -> ()  [unwired: 1 out]
        }
      }
      n183 = stacked-sequence {
        tunnel: w103 -> [w157 _ w159]
        tunnel: [w157 _ _] -> w104
        frame #0 {
          n184 = local write "Ch 03 Status 2"("Ch3 ON/OFF") -> ()
          n185 = local write "Ch 03 Status"("Ch3 ON/OFF") -> ()
        }
        frame #1 {
          n186 = local write "Ch 04 Status"("Ch4 ON/OFF") -> ()
          n187 = local write "Ch 04 Status 2"("Ch4 ON/OFF") -> ()
        }
        frame #2 {
          n188 = stacked-sequence {
            tunnel: w159 -> [w160 w165 w172 w177]
            frame #0 {
              w163 = 16 items=["*RST", "*VER", "*CA1", "*CA2", "*SS1", "*SS2", "*SU1", "*SU2", "*SD1", "*SD2", "*CS1", "*CS2", "*AT1", "*AT2", "*AN1", "*AN2", "*PW1", "*PW2", "*TL1", "*TL2", "*ST1", "*ST2", "*ET1", "*ET2", "*EM1", "*EM2", "*SC1", "*SC2"] ("string to write")
              n189 = call "Send.vi"("string to write"=w163, "port number"=w160, "Option"="532") -> ()
              n190 = Wait (ms)(milliseconds to wait=10) -> ()  [unwired: 1 out]
            }
            frame #1 {
              n191 = local read "Ch 03 Status"() -> (w164:bool)
              n192 = case shown="True" w164 {
                tunnel: w165 -> [_ w171]
                frame False {
                }
                frame True {
                  n193 = local read "Ch 04 Status"() -> (w168:bool)
                  n194 = local read "Ch 03 Status"() -> (w170:bool)
                  n195 = call "Read Scale Ch 1.vi"("Ch2"=w168, "Com Port"=w171, "Ch 1"=w170) -> ("Scale 1Ch"=w167:dbl, "Trigger Status Ch1"=w166:bool, "Wavelength"=w169:u32)
                  n196 = local write "Wavelength 3"(w169) -> ()
                  n197 = local write "Scale 3"(w167) -> ()
                  n198 = local write "Trigger ch 3"(w166) -> ()
                }
              }
            }
            frame #2 {
              w175 = 17 items=["*RST", "*VER", "*CA1", "*CA2", "*SS1", "*SS2", "*SU1", "*SU2", "*SD1", "*SD2", "*CS1", "*CS2", "*AT1", "*AT2", "*AN1", "*AN2", "*PW1", "*PW2", "*TL1", "*TL2", "*ST1", "*ST2", "*ET1", "*ET2", "*EM1", "*EM2", "*SC1", "*SC2"] ("string to write")
              n199 = call "Send.vi"("string to write"=w175, "port number"=w172, "Option"="532") -> ()
              n200 = Wait (ms)(milliseconds to wait=10) -> ()  [unwired: 1 out]
            }
            frame #3 {
              n201 = local read "Ch 04 Status"() -> (w176:bool)
              n202 = case shown="True" w176 {
                tunnel: w177 -> [_ w183]
                frame False {
                }
                frame True {
                  n203 = local read "Ch 03 Status"() -> (w181:bool)
                  n204 = local read "Ch 04 Status"() -> (w180:bool)
                  n205 = call "Read Scale Ch 2.vi"("Ch 2"=w180, "Com Port"=w183, "Ch1"=w181) -> ("Scale Ch2"=w182:dbl, "External Trigger Ch2"=w178:bool, "Wavelength"=w179:u32)
                  n206 = local write "Trigger ch 4"(w178) -> ()
                  n207 = local write "Wavelength 4"(w179) -> ()
                  n208 = local write "Scale 4"(w182) -> ()
                }
              }
            }
          }
        }
      }
    }
    frame #3 {
      # "See frame 2 for explanations"
      # "Initializing com port 3"
      n209 = stacked-sequence {
        tunnel: [w186 _ _ _ _ _ _ _ _ _] -> w184
        frame #0 {
          n210 = local read "Com Port 3"() -> (w186:refnum<visa-resource-name>)
          n211 = local write "Stop Application"(TRUE ("Stop programme")) -> ()
          n212 = call "Init.vi"("Baud Rate 2"=u32 921600 ("Baud Rate 3"), "# Port"=w186) -> ()  [unwired: 1 in]
          n213 = Wait (ms)(milliseconds to wait=10) -> ()  [unwired: 1 out]
        }
        frame #1 {
          w190 = 0 items=["*RST", "*VER", "*CA1", "*CA2", "*SS100", "*SS200", "*SU1", "*SU2", "*SD1", "*SD2", "*CS1", "*CS2", "*AT1", "*AT2", "*AN1", "*AN2", "*PW1", "*PW2", "*TL1", "*TL2", "*ST1", "*ST2", "*ET1", "*ET2", "*EM1", "*EM2", "*SC1", "*SC2"] ("string to write")
          n214 = local read "Com Port 3"() -> (w192:refnum<visa-resource-name>)
          n215 = call "Send.vi"("string to write"=w190, "port number"=w192) -> ()  [unwired: 1 in]
          n216 = Wait (ms)(milliseconds to wait=500) -> ()  [unwired: 1 out]
        }
        frame #2 {
          w199 = 4 items=["*RST", "*VER", "*CA1", "*CA2", "*SS1", "*SS2", "*SU1", "*SU2", "*SD1", "*SD2", "*CS1", "*CS2", "*AT1", "*AT2", "*AN1", "*AN2", "*PW1", "*PW2", "*TL1", "*TL2", "*ST1", "*ST2", "*ET1", "*ET2", "*EM1", "*EM2", "*SC1", "*SC2"] ("string to write")
          n217 = Number To Decimal String(number=1, width (-)=i16 3) -> (decimal integer string=w194:string)
          n218 = local read "Com Port 3"() -> (w201:refnum<visa-resource-name>)
          n219 = Search and Replace String(replace all?=TRUE ("replace all? (F)"), input string=w194, search string=" ", replace string="0" ("replace string (\"\")")) -> (result string=w195:string)  [unwired: 4 in, 3 out]
          n220 = call "Send.vi"("string to write"=w199, "port number"=w201, "Option"=w195) -> ()
          n221 = Wait (ms)(milliseconds to wait=10) -> ()  [unwired: 1 out]
        }
        frame #3 {
          w209 = 5 items=["*RST", "*VER", "*CA1", "*CA2", "*SS1", "*SS2", "*SU1", "*SU2", "*SD1", "*SD2", "*CS1", "*CS2", "*AT1", "*AT2", "*AN1", "*AN2", "*PW1", "*PW2", "*TL1", "*TL2", "*ST1", "*ST2", "*ET1", "*ET2", "*EM1", "*EM2", "*SC1", "*SC2"] ("string to write")
          n222 = Number To Decimal String(number=1, width (-)=i16 3) -> (decimal integer string=w208:string)
          n223 = local read "Com Port 3"() -> (w211:refnum<visa-resource-name>)
          n224 = Search and Replace String(replace all?=TRUE ("replace all? (F)"), input string=w208, search string=" ", replace string="0" ("replace string (\"\")")) -> (result string=w204:string)  [unwired: 4 in, 3 out]
          n225 = call "Send.vi"("string to write"=w209, "port number"=w211, "Option"=w204) -> ()
          n226 = Wait (ms)(milliseconds to wait=10) -> ()  [unwired: 1 out]
        }
        frame #4 {
          w215 = 22 items=["*RST", "*VER", "*CA1", "*CA2", "*SS1", "*SS2", "*SU1", "*SU2", "*SD1", "*SD2", "*CS1", "*CS2", "*AT1", "*AT2", "*AN1", "*AN2", "*PW1", "*PW2", "*TL1", "*TL2", "*ST1", "*ST2", "*ET1", "*ET2", "*EM1", "*EM2", "*SC1", "*SC2"] ("string to write")
          n227 = local read "Com Port 3"() -> (w213:refnum<visa-resource-name>)
          n228 = call "Send.vi"("string to write"=w215, "port number"=w213, "Option"="1") -> ()
          n229 = Wait (ms)(milliseconds to wait=10) -> ()  [unwired: 1 out]
        }
        frame #5 {
          w219 = 23 items=["*RST", "*VER", "*CA1", "*CA2", "*SS1", "*SS2", "*SU1", "*SU2", "*SD1", "*SD2", "*CS1", "*CS2", "*AT1", "*AT2", "*AN1", "*AN2", "*PW1", "*PW2", "*TL1", "*TL2", "*ST1", "*ST2", "*ET1", "*ET2", "*EM1", "*EM2", "*SC1", "*SC2"] ("string to write")
          n230 = local read "Com Port 3"() -> (w217:refnum<visa-resource-name>)
          n231 = call "Send.vi"("string to write"=w219, "port number"=w217, "Option"="1") -> ()
          n232 = Wait (ms)(milliseconds to wait=10) -> ()  [unwired: 1 out]
        }
        frame #6 {
          w223 = 26 items=["*RST", "*VER", "*CA1", "*CA2", "*SS1", "*SS2", "*SU1", "*SU2", "*SD1", "*SD2", "*CS1", "*CS2", "*AT1", "*AT2", "*AN1", "*AN2", "*PW1", "*PW2", "*TL1", "*TL2", "*ST1", "*ST2", "*ET1", "*ET2", "*EM1", "*EM2", "*SC1", "*SC2"] ("string to write")
          n233 = local read "Com Port 3"() -> (w221:refnum<visa-resource-name>)
          n234 = call "Send.vi"("string to write"=w223, "port number"=w221, "Option"="21") -> ()
          n235 = Wait (ms)(milliseconds to wait=10) -> ()  [unwired: 1 out]
        }
        frame #7 {
          w227 = 27 items=["*RST", "*VER", "*CA1", "*CA2", "*SS1", "*SS2", "*SU1", "*SU2", "*SD1", "*SD2", "*CS1", "*CS2", "*AT1", "*AT2", "*AN1", "*AN2", "*PW1", "*PW2", "*TL1", "*TL2", "*ST1", "*ST2", "*ET1", "*ET2", "*EM1", "*EM2", "*SC1", "*SC2"] ("string to write")
          n236 = local read "Com Port 3"() -> (w225:refnum<visa-resource-name>)
          n237 = call "Send.vi"("string to write"=w227, "port number"=w225, "Option"="21") -> ()
          n238 = Wait (ms)(milliseconds to wait=10) -> ()  [unwired: 1 out]
        }
        frame #8 {
          w231 = 18 items=["*RST", "*VER", "*CA1", "*CA2", "*SS1", "*SS2", "*SU1", "*SU2", "*SD1", "*SD2", "*CS1", "*CS2", "*AT1", "*AT2", "*AN1", "*AN2", "*PW1", "*PW2", "*TL1", "*TL2", "*ST1", "*ST2", "*ET1", "*ET2", "*EM1", "*EM2", "*SC1", "*SC2"] ("string to write")
          n239 = local read "Com Port 3"() -> (w229:refnum<visa-resource-name>)
          n240 = call "Send.vi"("string to write"=w231, "port number"=w229, "Option"="00.5") -> ()
          n241 = Wait (ms)(milliseconds to wait=10) -> ()  [unwired: 1 out]
        }
        frame #9 {
          w235 = 19 items=["*RST", "*VER", "*CA1", "*CA2", "*SS1", "*SS2", "*SU1", "*SU2", "*SD1", "*SD2", "*CS1", "*CS2", "*AT1", "*AT2", "*AN1", "*AN2", "*PW1", "*PW2", "*TL1", "*TL2", "*ST1", "*ST2", "*ET1", "*ET2", "*EM1", "*EM2", "*SC1", "*SC2"] ("string to write")
          n242 = local read "Com Port 3"() -> (w233:refnum<visa-resource-name>)
          n243 = call "Send.vi"("string to write"=w235, "port number"=w233, "Option"="00.5") -> ()
          n244 = Wait (ms)(milliseconds to wait=10) -> ()  [unwired: 1 out]
        }
      }
      n245 = stacked-sequence {
        tunnel: w184 -> [w238 _ w240]
        tunnel: [w238 _ _] -> w185
        frame #0 {
          n246 = local write "Ch 05 Status"("Ch5 ON/OFF") -> ()
          n247 = local write "Ch 05 Status 2"("Ch5 ON/OFF") -> ()
        }
        frame #1 {
          n248 = local write "Ch 06 Status"("Ch6 ON/OFF") -> ()
          n249 = local write "Ch 06 Status 2"("Ch6 ON/OFF") -> ()
        }
        frame #2 {
          n250 = stacked-sequence {
            tunnel: w240 -> [w241 w246 w253 w258]
            frame #0 {
              w244 = 16 items=["*RST", "*VER", "*CA1", "*CA2", "*SS1", "*SS2", "*SU1", "*SU2", "*SD1", "*SD2", "*CS1", "*CS2", "*AT1", "*AT2", "*AN1", "*AN2", "*PW1", "*PW2", "*TL1", "*TL2", "*ST1", "*ST2", "*ET1", "*ET2", "*EM1", "*EM2", "*SC1", "*SC2"] ("string to write")
              n251 = call "Send.vi"("string to write"=w244, "port number"=w241, "Option"="532") -> ()
              n252 = Wait (ms)(milliseconds to wait=10) -> ()  [unwired: 1 out]
            }
            frame #1 {
              n253 = local read "Ch 05 Status"() -> (w245:bool)
              n254 = case shown="True" w245 {
                tunnel: w246 -> [_ w252]
                frame False {
                }
                frame True {
                  n255 = local read "Ch 05 Status"() -> (w251:bool)
                  n256 = local read "Ch 06 Status"() -> (w249:bool)
                  n257 = call "Read Scale Ch 1.vi"("Ch2"=w249, "Com Port"=w252, "Ch 1"=w251) -> ("Scale 1Ch"=w248:dbl, "Trigger Status Ch1"=w247:bool, "Wavelength"=w250:u32)
                  n258 = local write "Trigger ch 5"(w247) -> ()
                  n259 = local write "Wavelength 5"(w250) -> ()
                  n260 = local write "Scale 5"(w248) -> ()
                }
              }
            }
            frame #2 {
              w256 = 17 items=["*RST", "*VER", "*CA1", "*CA2", "*SS1", "*SS2", "*SU1", "*SU2", "*SD1", "*SD2", "*CS1", "*CS2", "*AT1", "*AT2", "*AN1", "*AN2", "*PW1", "*PW2", "*TL1", "*TL2", "*ST1", "*ST2", "*ET1", "*ET2", "*EM1", "*EM2", "*SC1", "*SC2"] ("string to write")
              n261 = call "Send.vi"("string to write"=w256, "port number"=w253, "Option"="532") -> ()
              n262 = Wait (ms)(milliseconds to wait=10) -> ()  [unwired: 1 out]
            }
            frame #3 {
              n263 = local read "Ch 06 Status"() -> (w257:bool)
              n264 = case shown="True" w257 {
                tunnel: w258 -> [_ w264]
                frame False {
                }
                frame True {
                  n265 = local read "Ch 05 Status"() -> (w262:bool)
                  n266 = local read "Ch 06 Status"() -> (w261:bool)
                  n267 = call "Read Scale Ch 2.vi"("Ch 2"=w261, "Com Port"=w264, "Ch1"=w262) -> ("Scale Ch2"=w263:dbl, "External Trigger Ch2"=w259:bool, "Wavelength"=w260:u32)
                  n268 = local write "Wavelength 6"(w260) -> ()
                  n269 = local write "Trigger ch 6"(w259) -> ()
                  n270 = local write "Scale 6"(w263) -> ()
                }
              }
            }
          }
        }
      }
    }
    frame #4 {
      # "See frame 2 for explanations"
      # "Initializing com port 4"
      n271 = stacked-sequence {
        tunnel: [w267 _ _ _ _ _ _ _] -> w265
        frame #0 {
          n272 = local read "Com Port 4"() -> (w267:refnum<visa-resource-name>)
          n273 = local write "Stop Application"(TRUE ("Stop programme")) -> ()
          n274 = call "Init.vi"("Baud Rate 2"=u32 921600 ("Baud Rate 3"), "# Port"=w267) -> ()  [unwired: 1 in]
          n275 = Wait (ms)(milliseconds to wait=10) -> ()  [unwired: 1 out]
        }
        frame #1 {
          w271 = 0 items=["*RST", "*VER", "*CA1", "*CA2", "*SS100", "*SS200", "*SU1", "*SU2", "*SD1", "*SD2", "*CS1", "*CS2", "*AT1", "*AT2", "*AN1", "*AN2", "*PW1", "*PW2", "*TL1", "*TL2", "*ST1", "*ST2", "*ET1", "*ET2", "*EM1", "*EM2", "*SC1", "*SC2"] ("string to write")
          n276 = local read "Com Port 4"() -> (w273:refnum<visa-resource-name>)
          n277 = call "Send.vi"("string to write"=w271, "port number"=w273) -> ()  [unwired: 1 in]
          n278 = Wait (ms)(milliseconds to wait=500) -> ()  [unwired: 1 out]
        }
        frame #2 {
          w280 = 4 items=["*RST", "*VER", "*CA1", "*CA2", "*SS1", "*SS2", "*SU1", "*SU2", "*SD1", "*SD2", "*CS1", "*CS2", "*AT1", "*AT2", "*AN1", "*AN2", "*PW1", "*PW2", "*TL1", "*TL2", "*ST1", "*ST2", "*ET1", "*ET2", "*EM1", "*EM2", "*SC1", "*SC2"] ("string to write")
          n279 = Number To Decimal String(number=1, width (-)=i16 3) -> (decimal integer string=w275:string)
          n280 = local read "Com Port 4"() -> (w282:refnum<visa-resource-name>)
          n281 = Search and Replace String(replace all?=TRUE ("replace all? (F)"), input string=w275, search string=" ", replace string="0" ("replace string (\"\")")) -> (result string=w276:string)  [unwired: 4 in, 3 out]
          n282 = call "Send.vi"("string to write"=w280, "port number"=w282, "Option"=w276) -> ()
          n283 = Wait (ms)(milliseconds to wait=10) -> ()  [unwired: 1 out]
        }
        frame #3 {
          w290 = 5 items=["*RST", "*VER", "*CA1", "*CA2", "*SS1", "*SS2", "*SU1", "*SU2", "*SD1", "*SD2", "*CS1", "*CS2", "*AT1", "*AT2", "*AN1", "*AN2", "*PW1", "*PW2", "*TL1", "*TL2", "*ST1", "*ST2", "*ET1", "*ET2", "*EM1", "*EM2", "*SC1", "*SC2"] ("string to write")
          n284 = Number To Decimal String(number=1, width (-)=i16 3) -> (decimal integer string=w289:string)
          n285 = local read "Com Port 4"() -> (w292:refnum<visa-resource-name>)
          n286 = Search and Replace String(replace all?=TRUE ("replace all? (F)"), input string=w289, search string=" ", replace string="0" ("replace string (\"\")")) -> (result string=w285:string)  [unwired: 4 in, 3 out]
          n287 = call "Send.vi"("string to write"=w290, "port number"=w292, "Option"=w285) -> ()
          n288 = Wait (ms)(milliseconds to wait=10) -> ()  [unwired: 1 out]
        }
        frame #4 {
          w296 = 22 items=["*RST", "*VER", "*CA1", "*CA2", "*SS1", "*SS2", "*SU1", "*SU2", "*SD1", "*SD2", "*CS1", "*CS2", "*AT1", "*AT2", "*AN1", "*AN2", "*PW1", "*PW2", "*TL1", "*TL2", "*ST1", "*ST2", "*ET1", "*ET2", "*EM1", "*EM2", "*SC1", "*SC2"] ("string to write")
          n289 = local read "Com Port 4"() -> (w294:refnum<visa-resource-name>)
          n290 = call "Send.vi"("string to write"=w296, "port number"=w294, "Option"="1") -> ()
          n291 = Wait (ms)(milliseconds to wait=10) -> ()  [unwired: 1 out]
        }
        frame #5 {
          w300 = 23 items=["*RST", "*VER", "*CA1", "*CA2", "*SS1", "*SS2", "*SU1", "*SU2", "*SD1", "*SD2", "*CS1", "*CS2", "*AT1", "*AT2", "*AN1", "*AN2", "*PW1", "*PW2", "*TL1", "*TL2", "*ST1", "*ST2", "*ET1", "*ET2", "*EM1", "*EM2", "*SC1", "*SC2"] ("string to write")
          n292 = local read "Com Port 4"() -> (w298:refnum<visa-resource-name>)
          n293 = call "Send.vi"("string to write"=w300, "port number"=w298, "Option"="1") -> ()
          n294 = Wait (ms)(milliseconds to wait=10) -> ()  [unwired: 1 out]
        }
        frame #6 {
          w304 = 26 items=["*RST", "*VER", "*CA1", "*CA2", "*SS1", "*SS2", "*SU1", "*SU2", "*SD1", "*SD2", "*CS1", "*CS2", "*AT1", "*AT2", "*AN1", "*AN2", "*PW1", "*PW2", "*TL1", "*TL2", "*ST1", "*ST2", "*ET1", "*ET2", "*EM1", "*EM2", "*SC1", "*SC2"] ("string to write")
          n295 = local read "Com Port 4"() -> (w302:refnum<visa-resource-name>)
          n296 = call "Send.vi"("string to write"=w304, "port number"=w302, "Option"="21") -> ()
          n297 = Wait (ms)(milliseconds to wait=10) -> ()  [unwired: 1 out]
        }
        frame #7 {
          w308 = 27 items=["*RST", "*VER", "*CA1", "*CA2", "*SS1", "*SS2", "*SU1", "*SU2", "*SD1", "*SD2", "*CS1", "*CS2", "*AT1", "*AT2", "*AN1", "*AN2", "*PW1", "*PW2", "*TL1", "*TL2", "*ST1", "*ST2", "*ET1", "*ET2", "*EM1", "*EM2", "*SC1", "*SC2"] ("string to write")
          n298 = local read "Com Port 4"() -> (w306:refnum<visa-resource-name>)
          n299 = call "Send.vi"("string to write"=w308, "port number"=w306, "Option"="21") -> ()
          n300 = Wait (ms)(milliseconds to wait=10) -> ()  [unwired: 1 out]
        }
      }
      n301 = stacked-sequence {
        tunnel: w265 -> [w311 _ w313]
        tunnel: [w311 _ _] -> w266
        frame #0 {
          n302 = local write "Ch 07 Status"("Ch7 ON/OFF") -> ()
          n303 = local write "Ch 07 Status 2"("Ch7 ON/OFF") -> ()
        }
        frame #1 {
          n304 = local write "Ch 08 Status 2"("Ch8 ON/OFF") -> ()
          n305 = local write "Ch 08 Status"("Ch8 ON/OFF") -> ()
        }
        frame #2 {
          n306 = stacked-sequence {
            tunnel: w313 -> [w314 w319 w326 w331]
            frame #0 {
              w317 = 16 items=["*RST", "*VER", "*CA1", "*CA2", "*SS1", "*SS2", "*SU1", "*SU2", "*SD1", "*SD2", "*CS1", "*CS2", "*AT1", "*AT2", "*AN1", "*AN2", "*PW1", "*PW2", "*TL1", "*TL2", "*ST1", "*ST2", "*ET1", "*ET2", "*EM1", "*EM2", "*SC1", "*SC2"] ("string to write")
              n307 = call "Send.vi"("string to write"=w317, "port number"=w314, "Option"="532") -> ()
              n308 = Wait (ms)(milliseconds to wait=10) -> ()  [unwired: 1 out]
            }
            frame #1 {
              n309 = local read "Ch 07 Status"() -> (w318:bool)
              n310 = case shown="True" w318 {
                tunnel: w319 -> [_ w325]
                frame False {
                }
                frame True {
                  n311 = local read "Ch 08 Status"() -> (w322:bool)
                  n312 = local read "Ch 07 Status"() -> (w324:bool)
                  n313 = call "Read Scale Ch 1.vi"("Ch2"=w322, "Com Port"=w325, "Ch 1"=w324) -> ("Scale 1Ch"=w321:dbl, "Trigger Status Ch1"=w320:bool, "Wavelength"=w323:u32)
                  n314 = local write "Wavelength 7"(w323) -> ()
                  n315 = local write "Scale 7"(w321) -> ()
                  n316 = local write "Trigger ch 7"(w320) -> ()
                }
              }
            }
            frame #2 {
              w329 = 17 items=["*RST", "*VER", "*CA1", "*CA2", "*SS1", "*SS2", "*SU1", "*SU2", "*SD1", "*SD2", "*CS1", "*CS2", "*AT1", "*AT2", "*AN1", "*AN2", "*PW1", "*PW2", "*TL1", "*TL2", "*ST1", "*ST2", "*ET1", "*ET2", "*EM1", "*EM2", "*SC1", "*SC2"] ("string to write")
              n317 = call "Send.vi"("string to write"=w329, "port number"=w326, "Option"="532") -> ()
              n318 = Wait (ms)(milliseconds to wait=10) -> ()  [unwired: 1 out]
            }
            frame #3 {
              n319 = local read "Ch 08 Status"() -> (w330:bool)
              n320 = case shown="True" w330 {
                tunnel: w331 -> [_ w336]
                frame False {
                }
                frame True {
                  n321 = local read "Ch 07 Status"() -> (w334:bool)
                  n322 = local read "Ch 08 Status"() -> (w332:bool)
                  n323 = call "Read Scale Ch 2.vi"("Ch 2"=w332, "Com Port"=w336, "Ch1"=w334) -> ("Scale Ch2"=w335:dbl, "Wavelength"=w333:u32)  [unwired: 1 out]
                  n324 = local write "Wavelength 8"(w333) -> ()
                  n325 = local write "Trigger ch 8"(w332) -> ()
                  n326 = local write "Scale 8"(w335) -> ()
                }
              }
            }
          }
        }
      }
    }
    frame #5 {
      # "See frame 2 for explanations"
      # "Initializing com port 5"
      n327 = stacked-sequence {
        tunnel: [w339 _ _ _ _ _ _ _] -> w337
        frame #0 {
          n328 = local read "Com Port 5"() -> (w339:refnum<visa-resource-name>)
          n329 = local write "Stop Application"(TRUE ("Stop programme")) -> ()
          n330 = call "Init.vi"("Baud Rate 2"=u32 921600 ("Baud Rate 3"), "# Port"=w339) -> ()  [unwired: 1 in]
          n331 = Wait (ms)(milliseconds to wait=10) -> ()  [unwired: 1 out]
        }
        frame #1 {
          w343 = 0 items=["*RST", "*VER", "*CA1", "*CA2", "*SS100", "*SS200", "*SU1", "*SU2", "*SD1", "*SD2", "*CS1", "*CS2", "*AT1", "*AT2", "*AN1", "*AN2", "*PW1", "*PW2", "*TL1", "*TL2", "*ST1", "*ST2", "*ET1", "*ET2", "*EM1", "*EM2", "*SC1", "*SC2"] ("string to write")
          n332 = local read "Com Port 5"() -> (w345:refnum<visa-resource-name>)
          n333 = call "Send.vi"("string to write"=w343, "port number"=w345) -> ()  [unwired: 1 in]
          n334 = Wait (ms)(milliseconds to wait=500) -> ()  [unwired: 1 out]
        }
        frame #2 {
          w352 = 4 items=["*RST", "*VER", "*CA1", "*CA2", "*SS1", "*SS2", "*SU1", "*SU2", "*SD1", "*SD2", "*CS1", "*CS2", "*AT1", "*AT2", "*AN1", "*AN2", "*PW1", "*PW2", "*TL1", "*TL2", "*ST1", "*ST2", "*ET1", "*ET2", "*EM1", "*EM2", "*SC1", "*SC2"] ("string to write")
          n335 = Number To Decimal String(number=1, width (-)=i16 3) -> (decimal integer string=w347:string)
          n336 = local read "Com Port 5"() -> (w354:refnum<visa-resource-name>)
          n337 = Search and Replace String(replace all?=TRUE ("replace all? (F)"), input string=w347, search string=" ", replace string="0" ("replace string (\"\")")) -> (result string=w348:string)  [unwired: 4 in, 3 out]
          n338 = call "Send.vi"("string to write"=w352, "port number"=w354, "Option"=w348) -> ()
          n339 = Wait (ms)(milliseconds to wait=10) -> ()  [unwired: 1 out]
        }
        frame #3 {
          w362 = 5 items=["*RST", "*VER", "*CA1", "*CA2", "*SS1", "*SS2", "*SU1", "*SU2", "*SD1", "*SD2", "*CS1", "*CS2", "*AT1", "*AT2", "*AN1", "*AN2", "*PW1", "*PW2", "*TL1", "*TL2", "*ST1", "*ST2", "*ET1", "*ET2", "*EM1", "*EM2", "*SC1", "*SC2"] ("string to write")
          n340 = Number To Decimal String(number=1, width (-)=i16 3) -> (decimal integer string=w361:string)
          n341 = local read "Com Port 5"() -> (w364:refnum<visa-resource-name>)
          n342 = Search and Replace String(replace all?=TRUE ("replace all? (F)"), input string=w361, search string=" ", replace string="0" ("replace string (\"\")")) -> (result string=w357:string)  [unwired: 4 in, 3 out]
          n343 = call "Send.vi"("string to write"=w362, "port number"=w364, "Option"=w357) -> ()
          n344 = Wait (ms)(milliseconds to wait=10) -> ()  [unwired: 1 out]
        }
        frame #4 {
          w368 = 22 items=["*RST", "*VER", "*CA1", "*CA2", "*SS1", "*SS2", "*SU1", "*SU2", "*SD1", "*SD2", "*CS1", "*CS2", "*AT1", "*AT2", "*AN1", "*AN2", "*PW1", "*PW2", "*TL1", "*TL2", "*ST1", "*ST2", "*ET1", "*ET2", "*EM1", "*EM2", "*SC1", "*SC2"] ("string to write")
          n345 = local read "Com Port 5"() -> (w366:refnum<visa-resource-name>)
          n346 = call "Send.vi"("string to write"=w368, "port number"=w366, "Option"="1") -> ()
          n347 = Wait (ms)(milliseconds to wait=10) -> ()  [unwired: 1 out]
        }
        frame #5 {
          w372 = 23 items=["*RST", "*VER", "*CA1", "*CA2", "*SS1", "*SS2", "*SU1", "*SU2", "*SD1", "*SD2", "*CS1", "*CS2", "*AT1", "*AT2", "*AN1", "*AN2", "*PW1", "*PW2", "*TL1", "*TL2", "*ST1", "*ST2", "*ET1", "*ET2", "*EM1", "*EM2", "*SC1", "*SC2"] ("string to write")
          n348 = local read "Com Port 5"() -> (w370:refnum<visa-resource-name>)
          n349 = call "Send.vi"("string to write"=w372, "port number"=w370, "Option"="1") -> ()
          n350 = Wait (ms)(milliseconds to wait=10) -> ()  [unwired: 1 out]
        }
        frame #6 {
          w376 = 26 items=["*RST", "*VER", "*CA1", "*CA2", "*SS1", "*SS2", "*SU1", "*SU2", "*SD1", "*SD2", "*CS1", "*CS2", "*AT1", "*AT2", "*AN1", "*AN2", "*PW1", "*PW2", "*TL1", "*TL2", "*ST1", "*ST2", "*ET1", "*ET2", "*EM1", "*EM2", "*SC1", "*SC2"] ("string to write")
          n351 = local read "Com Port 5"() -> (w374:refnum<visa-resource-name>)
          n352 = call "Send.vi"("string to write"=w376, "port number"=w374, "Option"="21") -> ()
          n353 = Wait (ms)(milliseconds to wait=10) -> ()  [unwired: 1 out]
        }
        frame #7 {
          w380 = 27 items=["*RST", "*VER", "*CA1", "*CA2", "*SS1", "*SS2", "*SU1", "*SU2", "*SD1", "*SD2", "*CS1", "*CS2", "*AT1", "*AT2", "*AN1", "*AN2", "*PW1", "*PW2", "*TL1", "*TL2", "*ST1", "*ST2", "*ET1", "*ET2", "*EM1", "*EM2", "*SC1", "*SC2"] ("string to write")
          n354 = local read "Com Port 5"() -> (w378:refnum<visa-resource-name>)
          n355 = call "Send.vi"("string to write"=w380, "port number"=w378, "Option"="21") -> ()
          n356 = Wait (ms)(milliseconds to wait=10) -> ()  [unwired: 1 out]
        }
      }
      n357 = stacked-sequence {
        tunnel: w337 -> [w383 _ w385]
        tunnel: [w383 _ _] -> w338
        frame #0 {
          n358 = local write "Ch 09 Status"("Ch9 ON/OFF") -> ()
          n359 = local write "Ch 09 Status 2"("Ch9 ON/OFF") -> ()
        }
        frame #1 {
          n360 = local write "Ch 10 Status 2"("Ch10 ON/OFF") -> ()
          n361 = local write "Ch 10 Status"("Ch10 ON/OFF") -> ()
        }
        frame #2 {
          n362 = stacked-sequence {
            tunnel: w385 -> [w386 w391 w398 w403]
            frame #0 {
              w389 = 16 items=["*RST", "*VER", "*CA1", "*CA2", "*SS1", "*SS2", "*SU1", "*SU2", "*SD1", "*SD2", "*CS1", "*CS2", "*AT1", "*AT2", "*AN1", "*AN2", "*PW1", "*PW2", "*TL1", "*TL2", "*ST1", "*ST2", "*ET1", "*ET2", "*EM1", "*EM2", "*SC1", "*SC2"] ("string to write")
              n363 = call "Send.vi"("string to write"=w389, "port number"=w386, "Option"="532") -> ()
              n364 = Wait (ms)(milliseconds to wait=10) -> ()  [unwired: 1 out]
            }
            frame #1 {
              n365 = local read "Ch 09 Status"() -> (w390:bool)
              n366 = case shown="True" w390 {
                tunnel: w391 -> [_ w397]
                frame False {
                }
                frame True {
                  n367 = local read "Ch 10 Status"() -> (w393:bool)
                  n368 = local read "Ch 09 Status"() -> (w396:bool)
                  n369 = call "Read Scale Ch 1.vi"("Ch2"=w393, "Com Port"=w397, "Ch 1"=w396) -> ("Scale 1Ch"=w394:dbl, "Trigger Status Ch1"=w392:bool, "Wavelength"=w395:u32)
                  n370 = local write "Trigger ch 9"(w392) -> ()
                  n371 = local write "Wavelength 9"(w395) -> ()
                  n372 = local write "Scale 9"(w394) -> ()
                }
              }
            }
            frame #2 {
              w401 = 17 items=["*RST", "*VER", "*CA1", "*CA2", "*SS1", "*SS2", "*SU1", "*SU2", "*SD1", "*SD2", "*CS1", "*CS2", "*AT1", "*AT2", "*AN1", "*AN2", "*PW1", "*PW2", "*TL1", "*TL2", "*ST1", "*ST2", "*ET1", "*ET2", "*EM1", "*EM2", "*SC1", "*SC2"] ("string to write")
              n373 = call "Send.vi"("string to write"=w401, "port number"=w398, "Option"="532") -> ()
              n374 = Wait (ms)(milliseconds to wait=10) -> ()  [unwired: 1 out]
            }
            frame #3 {
              n375 = local read "Ch 10 Status"() -> (w402:bool)
              n376 = case shown="True" w402 {
                tunnel: w403 -> [_ w409]
                frame False {
                }
                frame True {
                  n377 = local read "Ch 09 Status"() -> (w407:bool)
                  n378 = local read "Ch 10 Status"() -> (w406:bool)
                  n379 = call "Read Scale Ch 2.vi"("Ch 2"=w406, "Com Port"=w409, "Ch1"=w407) -> ("Scale Ch2"=w408:dbl, "External Trigger Ch2"=w404:bool, "Wavelength"=w405:u32)
                  n380 = local write "Wavelength 10"(w405) -> ()
                  n381 = local write "Trigger ch 10"(w404) -> ()
                  n382 = local write "Scale 10"(w408) -> ()
                }
              }
            }
          }
        }
      }
    }
    frame #6 {
      # "See frame 2 for explanations"
      # "Initializing com port 6"
      n383 = stacked-sequence {
        tunnel: [w412 _ _ _ _ _ _ _] -> w411
        frame #0 {
          n384 = local read "Com Port 6"() -> (w412:refnum<visa-resource-name>)
          n385 = local write "Stop Application"(TRUE ("Stop programme")) -> ()
          n386 = call "Init.vi"("Baud Rate 2"=u32 921600 ("Baud Rate 3"), "# Port"=w412) -> ()  [unwired: 1 in]
          n387 = Wait (ms)(milliseconds to wait=10) -> ()  [unwired: 1 out]
        }
        frame #1 {
          w416 = 0 items=["*RST", "*VER", "*CA1", "*CA2", "*SS100", "*SS200", "*SU1", "*SU2", "*SD1", "*SD2", "*CS1", "*CS2", "*AT1", "*AT2", "*AN1", "*AN2", "*PW1", "*PW2", "*TL1", "*TL2", "*ST1", "*ST2", "*ET1", "*ET2", "*EM1", "*EM2", "*SC1", "*SC2"] ("string to write")
          n388 = local read "Com Port 6"() -> (w418:refnum<visa-resource-name>)
          n389 = call "Send.vi"("string to write"=w416, "port number"=w418) -> ()  [unwired: 1 in]
          n390 = Wait (ms)(milliseconds to wait=500) -> ()  [unwired: 1 out]
        }
        frame #2 {
          w425 = 4 items=["*RST", "*VER", "*CA1", "*CA2", "*SS1", "*SS2", "*SU1", "*SU2", "*SD1", "*SD2", "*CS1", "*CS2", "*AT1", "*AT2", "*AN1", "*AN2", "*PW1", "*PW2", "*TL1", "*TL2", "*ST1", "*ST2", "*ET1", "*ET2", "*EM1", "*EM2", "*SC1", "*SC2"] ("string to write")
          n391 = Number To Decimal String(number=1, width (-)=i16 3) -> (decimal integer string=w420:string)
          n392 = local read "Com Port 6"() -> (w427:refnum<visa-resource-name>)
          n393 = Search and Replace String(replace all?=TRUE ("replace all? (F)"), input string=w420, search string=" ", replace string="0" ("replace string (\"\")")) -> (result string=w421:string)  [unwired: 4 in, 3 out]
          n394 = call "Send.vi"("string to write"=w425, "port number"=w427, "Option"=w421) -> ()
          n395 = Wait (ms)(milliseconds to wait=10) -> ()  [unwired: 1 out]
        }
        frame #3 {
          w435 = 5 items=["*RST", "*VER", "*CA1", "*CA2", "*SS1", "*SS2", "*SU1", "*SU2", "*SD1", "*SD2", "*CS1", "*CS2", "*AT1", "*AT2", "*AN1", "*AN2", "*PW1", "*PW2", "*TL1", "*TL2", "*ST1", "*ST2", "*ET1", "*ET2", "*EM1", "*EM2", "*SC1", "*SC2"] ("string to write")
          n396 = Number To Decimal String(number=1, width (-)=i16 3) -> (decimal integer string=w434:string)
          n397 = local read "Com Port 6"() -> (w437:refnum<visa-resource-name>)
          n398 = Search and Replace String(replace all?=TRUE ("replace all? (F)"), input string=w434, search string=" ", replace string="0" ("replace string (\"\")")) -> (result string=w430:string)  [unwired: 4 in, 3 out]
          n399 = call "Send.vi"("string to write"=w435, "port number"=w437, "Option"=w430) -> ()
          n400 = Wait (ms)(milliseconds to wait=10) -> ()  [unwired: 1 out]
        }
        frame #4 {
          w441 = 22 items=["*RST", "*VER", "*CA1", "*CA2", "*SS1", "*SS2", "*SU1", "*SU2", "*SD1", "*SD2", "*CS1", "*CS2", "*AT1", "*AT2", "*AN1", "*AN2", "*PW1", "*PW2", "*TL1", "*TL2", "*ST1", "*ST2", "*ET1", "*ET2", "*EM1", "*EM2", "*SC1", "*SC2"] ("string to write")
          n401 = local read "Com Port 6"() -> (w439:refnum<visa-resource-name>)
          n402 = call "Send.vi"("string to write"=w441, "port number"=w439, "Option"="1") -> ()
          n403 = Wait (ms)(milliseconds to wait=10) -> ()  [unwired: 1 out]
        }
        frame #5 {
          w445 = 23 items=["*RST", "*VER", "*CA1", "*CA2", "*SS1", "*SS2", "*SU1", "*SU2", "*SD1", "*SD2", "*CS1", "*CS2", "*AT1", "*AT2", "*AN1", "*AN2", "*PW1", "*PW2", "*TL1", "*TL2", "*ST1", "*ST2", "*ET1", "*ET2", "*EM1", "*EM2", "*SC1", "*SC2"] ("string to write")
          n404 = local read "Com Port 6"() -> (w443:refnum<visa-resource-name>)
          n405 = call "Send.vi"("string to write"=w445, "port number"=w443, "Option"="1") -> ()
          n406 = Wait (ms)(milliseconds to wait=10) -> ()  [unwired: 1 out]
        }
        frame #6 {
          w449 = 26 items=["*RST", "*VER", "*CA1", "*CA2", "*SS1", "*SS2", "*SU1", "*SU2", "*SD1", "*SD2", "*CS1", "*CS2", "*AT1", "*AT2", "*AN1", "*AN2", "*PW1", "*PW2", "*TL1", "*TL2", "*ST1", "*ST2", "*ET1", "*ET2", "*EM1", "*EM2", "*SC1", "*SC2"] ("string to write")
          n407 = local read "Com Port 6"() -> (w447:refnum<visa-resource-name>)
          n408 = call "Send.vi"("string to write"=w449, "port number"=w447, "Option"="19") -> ()
          n409 = Wait (ms)(milliseconds to wait=10) -> ()  [unwired: 1 out]
        }
        frame #7 {
          w453 = 27 items=["*RST", "*VER", "*CA1", "*CA2", "*SS1", "*SS2", "*SU1", "*SU2", "*SD1", "*SD2", "*CS1", "*CS2", "*AT1", "*AT2", "*AN1", "*AN2", "*PW1", "*PW2", "*TL1", "*TL2", "*ST1", "*ST2", "*ET1", "*ET2", "*EM1", "*EM2", "*SC1", "*SC2"] ("string to write")
          n410 = local read "Com Port 6"() -> (w451:refnum<visa-resource-name>)
          n411 = call "Send.vi"("string to write"=w453, "port number"=w451, "Option"="21") -> ()
          n412 = Wait (ms)(milliseconds to wait=10) -> ()  [unwired: 1 out]
        }
      }
      n413 = stacked-sequence {
        tunnel: w411 -> [w456 _ w458]
        tunnel: [w456 _ _] -> w410
        frame #0 {
          n414 = local write "Ch 11 Status"("Ch11 ON/OFF") -> ()
          n415 = local write "Ch 11 Status 2"("Ch11 ON/OFF") -> ()
        }
        frame #1 {
          n416 = local write "Ch 12 Status 2"("Ch12 ON/OFF") -> ()
          n417 = local write "Ch 12 Status"("Ch12 ON/OFF") -> ()
        }
        frame #2 {
          n418 = stacked-sequence {
            tunnel: w458 -> [w459 w464 w471 w476]
            frame #0 {
              w462 = 16 items=["*RST", "*VER", "*CA1", "*CA2", "*SS1", "*SS2", "*SU1", "*SU2", "*SD1", "*SD2", "*CS1", "*CS2", "*AT1", "*AT2", "*AN1", "*AN2", "*PW1", "*PW2", "*TL1", "*TL2", "*ST1", "*ST2", "*ET1", "*ET2", "*EM1", "*EM2", "*SC1", "*SC2"] ("string to write")
              n419 = call "Send.vi"("string to write"=w462, "port number"=w459, "Option"="800") -> ()
              n420 = Wait (ms)(milliseconds to wait=10) -> ()  [unwired: 1 out]
            }
            frame #1 {
              n421 = local read "Ch 11 Status"() -> (w463:bool)
              n422 = case shown="True" w463 {
                tunnel: w464 -> [_ w470]
                frame False {
                }
                frame True {
                  n423 = local read "Ch 12 Status"() -> (w466:bool)
                  n424 = local read "Ch 11 Status"() -> (w469:bool)
                  n425 = call "Read Scale Ch 1.vi"("Ch2"=w466, "Com Port"=w470, "Ch 1"=w469) -> ("Scale 1Ch"=w467:dbl, "Trigger Status Ch1"=w465:bool, "Wavelength"=w468:u32)
                  n426 = local write "Trigger ch 11"(w465) -> ()
                  n427 = local write "Wavelength 11"(w468) -> ()
                  n428 = local write "Scale 11"(w467) -> ()
                }
              }
            }
            frame #2 {
              w474 = 17 items=["*RST", "*VER", "*CA1", "*CA2", "*SS1", "*SS2", "*SU1", "*SU2", "*SD1", "*SD2", "*CS1", "*CS2", "*AT1", "*AT2", "*AN1", "*AN2", "*PW1", "*PW2", "*TL1", "*TL2", "*ST1", "*ST2", "*ET1", "*ET2", "*EM1", "*EM2", "*SC1", "*SC2"] ("string to write")
              n429 = call "Send.vi"("string to write"=w474, "port number"=w471, "Option"="800") -> ()
              n430 = Wait (ms)(milliseconds to wait=10) -> ()  [unwired: 1 out]
            }
            frame #3 {
              n431 = local read "Ch 12 Status"() -> (w475:bool)
              n432 = case shown="True" w475 {
                tunnel: w476 -> [_ w482]
                frame False {
                }
                frame True {
                  n433 = local read "Ch 11 Status"() -> (w480:bool)
                  n434 = local read "Ch 12 Status"() -> (w479:bool)
                  n435 = call "Read Scale Ch 2.vi"("Ch 2"=w479, "Com Port"=w482, "Ch1"=w480) -> ("Scale Ch2"=w481:dbl, "External Trigger Ch2"=w477:bool, "Wavelength"=w478:u32)
                  n436 = local write "Wavelength 12"(w478) -> ()
                  n437 = local write "Trigger ch 12"(w477) -> ()
                  n438 = local write "Scale 12"(w481) -> ()
                }
              }
            }
          }
        }
      }
    }
    frame #7 {
      # "See frame 2 for explanations"
      # "Initializing com port 7"
      n439 = stacked-sequence {
        tunnel: [w485 _ _ _ _ _ _ _] -> w484
        frame #0 {
          n440 = local read "Com Port 7"() -> (w485:refnum<visa-resource-name>)
          n441 = local write "Stop Application"(TRUE ("Stop programme")) -> ()
          n442 = call "Init.vi"("Baud Rate 2"=u32 921600 ("Baud Rate 3"), "# Port"=w485) -> ()  [unwired: 1 in]
          n443 = Wait (ms)(milliseconds to wait=10) -> ()  [unwired: 1 out]
        }
        frame #1 {
          w489 = 0 items=["*RST", "*VER", "*CA1", "*CA2", "*SS100", "*SS200", "*SU1", "*SU2", "*SD1", "*SD2", "*CS1", "*CS2", "*AT1", "*AT2", "*AN1", "*AN2", "*PW1", "*PW2", "*TL1", "*TL2", "*ST1", "*ST2", "*ET1", "*ET2", "*EM1", "*EM2", "*SC1", "*SC2"] ("string to write")
          n444 = local read "Com Port 7"() -> (w491:refnum<visa-resource-name>)
          n445 = call "Send.vi"("string to write"=w489, "port number"=w491) -> ()  [unwired: 1 in]
          n446 = Wait (ms)(milliseconds to wait=500) -> ()  [unwired: 1 out]
        }
        frame #2 {
          w498 = 4 items=["*RST", "*VER", "*CA1", "*CA2", "*SS1", "*SS2", "*SU1", "*SU2", "*SD1", "*SD2", "*CS1", "*CS2", "*AT1", "*AT2", "*AN1", "*AN2", "*PW1", "*PW2", "*TL1", "*TL2", "*ST1", "*ST2", "*ET1", "*ET2", "*EM1", "*EM2", "*SC1", "*SC2"] ("string to write")
          n447 = Number To Decimal String(number=1, width (-)=i16 3) -> (decimal integer string=w493:string)
          n448 = local read "Com Port 7"() -> (w500:refnum<visa-resource-name>)
          n449 = Search and Replace String(replace all?=TRUE ("replace all? (F)"), input string=w493, search string=" ", replace string="0" ("replace string (\"\")")) -> (result string=w494:string)  [unwired: 4 in, 3 out]
          n450 = call "Send.vi"("string to write"=w498, "port number"=w500, "Option"=w494) -> ()
          n451 = Wait (ms)(milliseconds to wait=10) -> ()  [unwired: 1 out]
        }
        frame #3 {
          w508 = 5 items=["*RST", "*VER", "*CA1", "*CA2", "*SS1", "*SS2", "*SU1", "*SU2", "*SD1", "*SD2", "*CS1", "*CS2", "*AT1", "*AT2", "*AN1", "*AN2", "*PW1", "*PW2", "*TL1", "*TL2", "*ST1", "*ST2", "*ET1", "*ET2", "*EM1", "*EM2", "*SC1", "*SC2"] ("string to write")
          n452 = Number To Decimal String(number=1, width (-)=i16 3) -> (decimal integer string=w507:string)
          n453 = local read "Com Port 7"() -> (w510:refnum<visa-resource-name>)
          n454 = Search and Replace String(replace all?=TRUE ("replace all? (F)"), input string=w507, search string=" ", replace string="0" ("replace string (\"\")")) -> (result string=w503:string)  [unwired: 4 in, 3 out]
          n455 = call "Send.vi"("string to write"=w508, "port number"=w510, "Option"=w503) -> ()
          n456 = Wait (ms)(milliseconds to wait=10) -> ()  [unwired: 1 out]
        }
        frame #4 {
          w514 = 22 items=["*RST", "*VER", "*CA1", "*CA2", "*SS1", "*SS2", "*SU1", "*SU2", "*SD1", "*SD2", "*CS1", "*CS2", "*AT1", "*AT2", "*AN1", "*AN2", "*PW1", "*PW2", "*TL1", "*TL2", "*ST1", "*ST2", "*ET1", "*ET2", "*EM1", "*EM2", "*SC1", "*SC2"] ("string to write")
          n457 = local read "Com Port 7"() -> (w512:refnum<visa-resource-name>)
          n458 = call "Send.vi"("string to write"=w514, "port number"=w512, "Option"="1") -> ()
          n459 = Wait (ms)(milliseconds to wait=10) -> ()  [unwired: 1 out]
        }
        frame #5 {
          w518 = 23 items=["*RST", "*VER", "*CA1", "*CA2", "*SS1", "*SS2", "*SU1", "*SU2", "*SD1", "*SD2", "*CS1", "*CS2", "*AT1", "*AT2", "*AN1", "*AN2", "*PW1", "*PW2", "*TL1", "*TL2", "*ST1", "*ST2", "*ET1", "*ET2", "*EM1", "*EM2", "*SC1", "*SC2"] ("string to write")
          n460 = local read "Com Port 7"() -> (w516:refnum<visa-resource-name>)
          n461 = call "Send.vi"("string to write"=w518, "port number"=w516, "Option"="1") -> ()
          n462 = Wait (ms)(milliseconds to wait=10) -> ()  [unwired: 1 out]
        }
        frame #6 {
          w522 = 26 items=["*RST", "*VER", "*CA1", "*CA2", "*SS1", "*SS2", "*SU1", "*SU2", "*SD1", "*SD2", "*CS1", "*CS2", "*AT1", "*AT2", "*AN1", "*AN2", "*PW1", "*PW2", "*TL1", "*TL2", "*ST1", "*ST2", "*ET1", "*ET2", "*EM1", "*EM2", "*SC1", "*SC2"] ("string to write")
          n463 = local read "Com Port 7"() -> (w520:refnum<visa-resource-name>)
          n464 = call "Send.vi"("string to write"=w522, "port number"=w520, "Option"="19") -> ()
          n465 = Wait (ms)(milliseconds to wait=10) -> ()  [unwired: 1 out]
        }
        frame #7 {
          w526 = 27 items=["*RST", "*VER", "*CA1", "*CA2", "*SS1", "*SS2", "*SU1", "*SU2", "*SD1", "*SD2", "*CS1", "*CS2", "*AT1", "*AT2", "*AN1", "*AN2", "*PW1", "*PW2", "*TL1", "*TL2", "*ST1", "*ST2", "*ET1", "*ET2", "*EM1", "*EM2", "*SC1", "*SC2"] ("string to write")
          n466 = local read "Com Port 7"() -> (w524:refnum<visa-resource-name>)
          n467 = call "Send.vi"("string to write"=w526, "port number"=w524, "Option"="15") -> ()
          n468 = Wait (ms)(milliseconds to wait=10) -> ()  [unwired: 1 out]
        }
      }
      n469 = stacked-sequence {
        tunnel: w484 -> [w529 _ w531]
        tunnel: [w529 _ _] -> w483
        frame #0 {
          n470 = local write "Ch 13 Status 2"("Ch13 ON/OFF") -> ()
          n471 = local write "Ch 13 Status"("Ch13 ON/OFF") -> ()
        }
        frame #1 {
          n472 = local write "Ch 14 Status 2"("Ch14 ON/OFF") -> ()
          n473 = local write "Ch 14 Status"("Ch14 ON/OFF") -> ()
        }
        frame #2 {
          n474 = stacked-sequence {
            tunnel: w531 -> [w532 w537 w544 w549]
            frame #0 {
              w534 = 16 items=["*RST", "*VER", "*CA1", "*CA2", "*SS1", "*SS2", "*SU1", "*SU2", "*SD1", "*SD2", "*CS1", "*CS2", "*AT1", "*AT2", "*AN1", "*AN2", "*PW1", "*PW2", "*TL1", "*TL2", "*ST1", "*ST2", "*ET1", "*ET2", "*EM1", "*EM2", "*SC1", "*SC2"] ("string to write")
              n475 = call "Send.vi"("string to write"=w534, "port number"=w532, "Option"="532") -> ()
              n476 = Wait (ms)(milliseconds to wait=10) -> ()  [unwired: 1 out]
            }
            frame #1 {
              n477 = local read "Ch 13 Status"() -> (w536:bool)
              n478 = case shown="True" w536 {
                tunnel: w537 -> [_ w543]
                frame False {
                }
                frame True {
                  n479 = local read "Ch 14 Status"() -> (w539:bool)
                  n480 = local read "Ch 13 Status"() -> (w542:bool)
                  n481 = call "Read Scale Ch 1.vi"("Ch2"=w539, "Com Port"=w543, "Ch 1"=w542) -> ("Scale 1Ch"=w540:dbl, "Trigger Status Ch1"=w538:bool, "Wavelength"=w541:u32)
                  n482 = local write "Trigger ch 13"(w538) -> ()
                  n483 = local write "Wavelength 13"(w541) -> ()
                  n484 = local write "Scale 13"(w540) -> ()
                }
              }
            }
            frame #2 {
              w546 = 17 items=["*RST", "*VER", "*CA1", "*CA2", "*SS1", "*SS2", "*SU1", "*SU2", "*SD1", "*SD2", "*CS1", "*CS2", "*AT1", "*AT2", "*AN1", "*AN2", "*PW1", "*PW2", "*TL1", "*TL2", "*ST1", "*ST2", "*ET1", "*ET2", "*EM1", "*EM2", "*SC1", "*SC2"] ("string to write")
              n485 = call "Send.vi"("string to write"=w546, "port number"=w544, "Option"="800") -> ()
              n486 = Wait (ms)(milliseconds to wait=10) -> ()  [unwired: 1 out]
            }
            frame #3 {
              n487 = local read "Ch 14 Status"() -> (w548:bool)
              n488 = case shown="True" w548 {
                tunnel: w549 -> [_ w555]
                frame False {
                }
                frame True {
                  n489 = local read "Ch 13 Status"() -> (w553:bool)
                  n490 = local read "Ch 14 Status"() -> (w552:bool)
                  n491 = call "Read Scale Ch 2.vi"("Ch 2"=w552, "Com Port"=w555, "Ch1"=w553) -> ("Scale Ch2"=w554:dbl, "External Trigger Ch2"=w550:bool, "Wavelength"=w551:u32)
                  n492 = local write "Wavelength 14"(w551) -> ()
                  n493 = local write "Trigger ch 14"(w550) -> ()
                  n494 = local write "Scale 14"(w554) -> ()
                }
              }
            }
          }
        }
      }
    }
    frame #8 {
      # "See frame 2 for explanations"
      # "Initializing com port 8"
      n495 = stacked-sequence {
        tunnel: [w558 _ _ _ _ _ _ _] -> w557
        frame #0 {
          n496 = local read "Com Port 8"() -> (w558:refnum<visa-resource-name>)
          n497 = local write "Stop Application"(TRUE ("Stop programme")) -> ()
          n498 = call "Init.vi"("Baud Rate 2"=u32 921600 ("Baud Rate 3"), "# Port"=w558) -> ()  [unwired: 1 in]
          n499 = Wait (ms)(milliseconds to wait=10) -> ()  [unwired: 1 out]
        }
        frame #1 {
          w562 = 0 items=["*RST", "*VER", "*CA1", "*CA2", "*SS100", "*SS200", "*SU1", "*SU2", "*SD1", "*SD2", "*CS1", "*CS2", "*AT1", "*AT2", "*AN1", "*AN2", "*PW1", "*PW2", "*TL1", "*TL2", "*ST1", "*ST2", "*ET1", "*ET2", "*EM1", "*EM2", "*SC1", "*SC2"] ("string to write")
          n500 = local read "Com Port 8"() -> (w564:refnum<visa-resource-name>)
          n501 = call "Send.vi"("string to write"=w562, "port number"=w564) -> ()  [unwired: 1 in]
          n502 = Wait (ms)(milliseconds to wait=500) -> ()  [unwired: 1 out]
        }
        frame #2 {
          w571 = 4 items=["*RST", "*VER", "*CA1", "*CA2", "*SS1", "*SS2", "*SU1", "*SU2", "*SD1", "*SD2", "*CS1", "*CS2", "*AT1", "*AT2", "*AN1", "*AN2", "*PW1", "*PW2", "*TL1", "*TL2", "*ST1", "*ST2", "*ET1", "*ET2", "*EM1", "*EM2", "*SC1", "*SC2"] ("string to write")
          n503 = Number To Decimal String(number=1, width (-)=i16 3) -> (decimal integer string=w566:string)
          n504 = local read "Com Port 8"() -> (w573:refnum<visa-resource-name>)
          n505 = Search and Replace String(replace all?=TRUE ("replace all? (F)"), input string=w566, search string=" ", replace string="0" ("replace string (\"\")")) -> (result string=w567:string)  [unwired: 4 in, 3 out]
          n506 = call "Send.vi"("string to write"=w571, "port number"=w573, "Option"=w567) -> ()
          n507 = Wait (ms)(milliseconds to wait=10) -> ()  [unwired: 1 out]
        }
        frame #3 {
          w581 = 5 items=["*RST", "*VER", "*CA1", "*CA2", "*SS1", "*SS2", "*SU1", "*SU2", "*SD1", "*SD2", "*CS1", "*CS2", "*AT1", "*AT2", "*AN1", "*AN2", "*PW1", "*PW2", "*TL1", "*TL2", "*ST1", "*ST2", "*ET1", "*ET2", "*EM1", "*EM2", "*SC1", "*SC2"] ("string to write")
          n508 = Number To Decimal String(number=1, width (-)=i16 3) -> (decimal integer string=w580:string)
          n509 = local read "Com Port 8"() -> (w583:refnum<visa-resource-name>)
          n510 = Search and Replace String(replace all?=TRUE ("replace all? (F)"), input string=w580, search string=" ", replace string="0" ("replace string (\"\")")) -> (result string=w576:string)  [unwired: 4 in, 3 out]
          n511 = call "Send.vi"("string to write"=w581, "port number"=w583, "Option"=w576) -> ()
          n512 = Wait (ms)(milliseconds to wait=10) -> ()  [unwired: 1 out]
        }
        frame #4 {
          w587 = 22 items=["*RST", "*VER", "*CA1", "*CA2", "*SS1", "*SS2", "*SU1", "*SU2", "*SD1", "*SD2", "*CS1", "*CS2", "*AT1", "*AT2", "*AN1", "*AN2", "*PW1", "*PW2", "*TL1", "*TL2", "*ST1", "*ST2", "*ET1", "*ET2", "*EM1", "*EM2", "*SC1", "*SC2"] ("string to write")
          n513 = local read "Com Port 8"() -> (w585:refnum<visa-resource-name>)
          n514 = call "Send.vi"("string to write"=w587, "port number"=w585, "Option"="1") -> ()
          n515 = Wait (ms)(milliseconds to wait=10) -> ()  [unwired: 1 out]
        }
        frame #5 {
          w591 = 23 items=["*RST", "*VER", "*CA1", "*CA2", "*SS1", "*SS2", "*SU1", "*SU2", "*SD1", "*SD2", "*CS1", "*CS2", "*AT1", "*AT2", "*AN1", "*AN2", "*PW1", "*PW2", "*TL1", "*TL2", "*ST1", "*ST2", "*ET1", "*ET2", "*EM1", "*EM2", "*SC1", "*SC2"] ("string to write")
          n516 = local read "Com Port 8"() -> (w589:refnum<visa-resource-name>)
          n517 = call "Send.vi"("string to write"=w591, "port number"=w589, "Option"="1") -> ()
          n518 = Wait (ms)(milliseconds to wait=10) -> ()  [unwired: 1 out]
        }
        frame #6 {
          w595 = 26 items=["*RST", "*VER", "*CA1", "*CA2", "*SS1", "*SS2", "*SU1", "*SU2", "*SD1", "*SD2", "*CS1", "*CS2", "*AT1", "*AT2", "*AN1", "*AN2", "*PW1", "*PW2", "*TL1", "*TL2", "*ST1", "*ST2", "*ET1", "*ET2", "*EM1", "*EM2", "*SC1", "*SC2"] ("string to write")
          n519 = local read "Com Port 8"() -> (w593:refnum<visa-resource-name>)
          n520 = call "Send.vi"("string to write"=w595, "port number"=w593, "Option"="21") -> ()
          n521 = Wait (ms)(milliseconds to wait=10) -> ()  [unwired: 1 out]
        }
        frame #7 {
          w599 = 27 items=["*RST", "*VER", "*CA1", "*CA2", "*SS1", "*SS2", "*SU1", "*SU2", "*SD1", "*SD2", "*CS1", "*CS2", "*AT1", "*AT2", "*AN1", "*AN2", "*PW1", "*PW2", "*TL1", "*TL2", "*ST1", "*ST2", "*ET1", "*ET2", "*EM1", "*EM2", "*SC1", "*SC2"] ("string to write")
          n522 = local read "Com Port 8"() -> (w597:refnum<visa-resource-name>)
          n523 = call "Send.vi"("string to write"=w599, "port number"=w597, "Option"="21") -> ()
          n524 = Wait (ms)(milliseconds to wait=10) -> ()  [unwired: 1 out]
        }
      }
      n525 = stacked-sequence {
        tunnel: w557 -> [w602 _ w606]
        tunnel: [w602 _ _] -> w556
        frame #0 {
          n526 = local write "Ch 15 Status"("C15 ON/OFF") -> ()
          n527 = local write "Ch 15 Status 2"("C15 ON/OFF") -> ()
        }
        frame #1 {
          n528 = local write "Ch 16 Status 2"("Ch16 ON/OFF") -> ()
          n529 = call "16Chennels_ExtraWindow.vi"("Ch 16 Status"="Ch16 ON/OFF") -> ()  [unwired: 9 in]
          n530 = local write "Ch 16 Status"("Ch16 ON/OFF") -> ()
          n531 = local read "Second Window Output"() -> (w605:T1)
          n532 = Bundle By Name(cluster=w605, "Status"="Ch16 ON/OFF") -> (w604:T1)
          n533 = local write "Second Window Output"(w604) -> ()
        }
        frame #2 {
          n534 = stacked-sequence {
            tunnel: w606 -> [w607 w612 w619 w624]
            frame #0 {
              w609 = 16 items=["*RST", "*VER", "*CA1", "*CA2", "*SS1", "*SS2", "*SU1", "*SU2", "*SD1", "*SD2", "*CS1", "*CS2", "*AT1", "*AT2", "*AN1", "*AN2", "*PW1", "*PW2", "*TL1", "*TL2", "*ST1", "*ST2", "*ET1", "*ET2", "*EM1", "*EM2", "*SC1", "*SC2"] ("string to write")
              n535 = call "Send.vi"("string to write"=w609, "port number"=w607, "Option"="800") -> ()
              n536 = Wait (ms)(milliseconds to wait=10) -> ()  [unwired: 1 out]
            }
            frame #1 {
              n537 = local read "Ch 15 Status"() -> (w611:bool)
              n538 = case shown="True" w611 {
                tunnel: w612 -> [_ w618]
                frame False {
                }
                frame True {
                  n539 = local read "Ch 16 Status"() -> (w614:bool)
                  n540 = local read "Ch 15 Status"() -> (w617:bool)
                  n541 = call "Read Scale Ch 1.vi"("Ch2"=w614, "Com Port"=w618, "Ch 1"=w617) -> ("Scale 1Ch"=w615:dbl, "Trigger Status Ch1"=w613:bool, "Wavelength"=w616:u32)
                  n542 = local write "Trigger ch 15"(w613) -> ()
                  n543 = local write "Wavelength 15"(w616) -> ()
                  n544 = local write "Scale 15"(w615) -> ()
                }
              }
            }
            frame #2 {
              w621 = 17 items=["*RST", "*VER", "*CA1", "*CA2", "*SS1", "*SS2", "*SU1", "*SU2", "*SD1", "*SD2", "*CS1", "*CS2", "*AT1", "*AT2", "*AN1", "*AN2", "*PW1", "*PW2", "*TL1", "*TL2", "*ST1", "*ST2", "*ET1", "*ET2", "*EM1", "*EM2", "*SC1", "*SC2"] ("string to write")
              n545 = call "Send.vi"("string to write"=w621, "port number"=w619, "Option"="800") -> ()
              n546 = Wait (ms)(milliseconds to wait=10) -> ()  [unwired: 1 out]
            }
            frame #3 {
              n547 = local read "Ch 16 Status"() -> (w623:bool)
              n548 = case shown="True" w623 {
                tunnel: w624 -> [_ w630]
                frame False {
                }
                frame True {
                  n549 = local read "Ch 15 Status"() -> (w628:bool)
                  n550 = local read "Ch 16 Status"() -> (w627:bool)
                  n551 = call "Read Scale Ch 2.vi"("Ch 2"=w627, "Com Port"=w630, "Ch1"=w628) -> ("Scale Ch2"=w629:dbl, "External Trigger Ch2"=w625:bool, "Wavelength"=w626:u32)
                  n552 = local write "Wavelength 16"(w626) -> ()
                  n553 = local write "Trigger ch 16"(w625) -> ()
                  n554 = local write "Scale 16"(w629) -> ()
                }
              }
            }
          }
        }
      }
    }
    frame #9 {
      # "Creating .csv files for all the meters"
      n555 = stacked-sequence {
        frame #0 {
          # "Get Current Date and Time"
          n556 = Format Date/Time String(time format string (%c)="%Y%m%d") -> (date/time string=w633:string)  [unwired: 2 in]
          n557 = Format Date/Time String(time format string (%c)="%H:%M:%S%2u") -> (date/time string=w634:string)  [unwired: 2 in]
          n558 = local write "Date"(w633) -> ()
          n559 = local write "Time"(w634) -> ()
        }
        frame #1 {
          # "Check if current date folder exists"
          n560 = local read "Base Path"() -> (w635:path)
          n561 = local read "Date"() -> (w641:string)
          n562 = String To Path(string=w641) -> (path=w640:path)
          n563 = Build Path(base path=w635, name or relative path=w640) -> (appended path=w639:path)
          n564 = call <vilib>:"Check if File or Folder Exists.vi"("path"=w639) -> ("error out"=w637:errorcluster, "file or folder exists?"=w636:bool, "dup path"=w638:path)  [unwired: 8 in]
          n565 = case shown="False" w636 {
            tunnel: w638 -> [w643 w645]
            tunnel: w637 -> [w642 _]
            frame False {
              # "Doesnot exist. Create the folder"
              n566 = Create Folder(path (use dialog)=w643, error in=w642) -> (created path=w644:path)  [unwired: 1 in, 2 out]
              n567 = local write "Folder"(w644) -> ()
            }
            frame True {
              # "Exist, output current path to base path"
              n568 = local write "Folder"(w645) -> ()
            }
          }
        }
        frame #2 {
          n569 = local read "Ch 01 Status"() -> (w646:bool)
          n570 = case shown="True" w646 {
            frame False {
            }
            frame True {
              # "Check if Frontend1.csv exists"
              n571 = local read "Folder"() -> (w651:path)
              n572 = Build Path(base path=w651, name or relative path="FrontEnd1.csv") -> (appended path=w650:path)
              n573 = call <vilib>:"Check if File or Folder Exists.vi"("path"=w650) -> ("file or folder exists?"=w649:bool, "dup path"=w648:path)  [unwired: 8 in, 1 out]
              n574 = case shown="False" w649 {
                tunnel: w648 -> [w654 w656]
                frame False {
                  # "Does not exist. Create the file, \nand write a header to it"
                  n575 = local write "Path Frontend #1"(w654) -> ()
                  n576 = call-poly <vilib>:"Write Delimited Spreadsheet.vi"("file path (dialog if empty)"=w654, "1D data"=string[] ["Timestamp", "Measured", "Calibrated"], "append to file? (new file:F)"=FALSE, "delimiter (\\t)"="," ("delimiter (\\t)")) -> ()  [unwired: 10 in, 2 out]
                }
                frame True {
                  # "Exists. Return File path"
                  n577 = local write "Path Frontend #1"(w656) -> ()
                }
              }
            }
          }
        }
        frame #3 {
          n578 = local read "Ch 02 Status"() -> (w657:bool)
          n579 = case shown="True" w657 {
            frame False {
            }
            frame True {
              # "See frame 2 for explanation"
              n580 = local read "Folder"() -> (w662:path)
              n581 = Build Path(base path=w662, name or relative path="FrontEnd2.csv") -> (appended path=w661:path)
              n582 = call <vilib>:"Check if File or Folder Exists.vi"("path"=w661) -> ("file or folder exists?"=w660:bool, "dup path"=w659:path)  [unwired: 8 in, 1 out]
              n583 = case shown="False" w660 {
                tunnel: w659 -> [w665 w667]
                frame False {
                  n584 = local write "Path Frontend #2"(w665) -> ()
                  n585 = call-poly <vilib>:"Write Delimited Spreadsheet.vi"("file path (dialog if empty)"=w665, "1D data"=string[] ["Timestamp", "Measured", "Calibrated"], "append to file? (new file:F)"=FALSE, "delimiter (\\t)"="," ("delimiter (\\t)")) -> ()  [unwired: 10 in, 2 out]
                }
                frame True {
                  n586 = local write "Path Frontend #2"(w667) -> ()
                }
              }
            }
          }
        }
        frame #4 {
          n587 = local read "Ch 03 Status"() -> (w668:bool)
          n588 = case shown="True" w668 {
            frame False {
            }
            frame True {
              # "See frame 2 for explanation"
              n589 = local read "Folder"() -> (w670:path)
              n590 = Build Path(base path=w670, name or relative path="SLAB2.csv") -> (appended path=w671:path)
              n591 = call <vilib>:"Check if File or Folder Exists.vi"("path"=w671) -> ("file or folder exists?"=w672:bool, "dup path"=w673:path)  [unwired: 8 in, 1 out]
              n592 = case shown="False" w672 {
                tunnel: w673 -> [w676 w678]
                frame False {
                  n593 = local write "Path SLAB #2"(w676) -> ()
                  n594 = call-poly <vilib>:"Write Delimited Spreadsheet.vi"("file path (dialog if empty)"=w676, "1D data"=string[] ["Timestamp", "Measured", "Calibrated"], "append to file? (new file:F)"=FALSE, "delimiter (\\t)"="," ("delimiter (\\t)")) -> ()  [unwired: 10 in, 2 out]
                }
                frame True {
                  n595 = local write "Path SLAB #2"(w678) -> ()
                }
              }
            }
          }
        }
        frame #5 {
          n596 = local read "Ch 06 Status"() -> (w679:bool)
          n597 = case shown="True" w679 {
            frame False {
            }
            frame True {
              # "See frame 2 for explanation"
              n598 = local read "Folder"() -> (w681:path)
              n599 = Build Path(base path=w681, name or relative path="SLAB3.csv") -> (appended path=w682:path)
              n600 = call <vilib>:"Check if File or Folder Exists.vi"("path"=w682) -> ("file or folder exists?"=w683:bool, "dup path"=w684:path)  [unwired: 8 in, 1 out]
              n601 = case shown="False" w683 {
                tunnel: w684 -> [w687 w689]
                frame False {
                  n602 = local write "Path SLAB #3"(w687) -> ()
                  n603 = call-poly <vilib>:"Write Delimited Spreadsheet.vi"("file path (dialog if empty)"=w687, "1D data"=string[] ["Timestamp", "Measured", "Calibrated"], "append to file? (new file:F)"=FALSE, "delimiter (\\t)"="," ("delimiter (\\t)")) -> ()  [unwired: 10 in, 2 out]
                }
                frame True {
                  n604 = local write "Path SLAB #3"(w689) -> ()
                }
              }
            }
          }
        }
        frame #6 {
          n605 = local read "Ch 04 Status"() -> (w690:bool)
          n606 = case shown="True" w690 {
            frame False {
            }
            frame True {
              # "See frame 2 for explanation"
              n607 = local read "Folder"() -> (w692:path)
              n608 = Build Path(base path=w692, name or relative path="SLAB4.csv") -> (appended path=w693:path)
              n609 = call <vilib>:"Check if File or Folder Exists.vi"("path"=w693) -> ("file or folder exists?"=w694:bool, "dup path"=w695:path)  [unwired: 8 in, 1 out]
              n610 = case shown="False" w694 {
                tunnel: w695 -> [w698 w700]
                frame False {
                  n611 = local write "Path SLAB #4"(w698) -> ()
                  n612 = call-poly <vilib>:"Write Delimited Spreadsheet.vi"("file path (dialog if empty)"=w698, "1D data"=string[] ["Timestamp", "Measured", "Calibrated"], "append to file? (new file:F)"=FALSE, "delimiter (\\t)"="," ("delimiter (\\t)")) -> ()  [unwired: 10 in, 2 out]
                }
                frame True {
                  n613 = local write "Path SLAB #4"(w700) -> ()
                }
              }
            }
          }
        }
        frame #7 {
          n614 = local read "Ch 05 Status"() -> (w701:bool)
          n615 = case shown="True" w701 {
            frame False {
            }
            frame True {
              # "See frame 2 for explanation"
              n616 = local read "Folder"() -> (w703:path)
              n617 = Build Path(base path=w703, name or relative path="SLAB5.csv") -> (appended path=w704:path)
              n618 = call <vilib>:"Check if File or Folder Exists.vi"("path"=w704) -> ("file or folder exists?"=w705:bool, "dup path"=w706:path)  [unwired: 8 in, 1 out]
              n619 = case shown="False" w705 {
                tunnel: w706 -> [w709 w711]
                frame False {
                  n620 = local write "Path SLAB #5"(w709) -> ()
                  n621 = call-poly <vilib>:"Write Delimited Spreadsheet.vi"("file path (dialog if empty)"=w709, "1D data"=string[] ["Timestamp", "Measured", "Calibrated"], "append to file? (new file:F)"=FALSE, "delimiter (\\t)"="," ("delimiter (\\t)")) -> ()  [unwired: 10 in, 2 out]
                }
                frame True {
                  n622 = local write "Path SLAB #5"(w711) -> ()
                }
              }
            }
          }
        }
        frame #8 {
          n623 = local read "Ch 07 Status"() -> (w712:bool)
          n624 = case shown="True" w712 {
            frame False {
            }
            frame True {
              # "See frame 2 for explanation"
              n625 = local read "Folder"() -> (w714:path)
              n626 = Build Path(base path=w714, name or relative path="SLAB7.csv") -> (appended path=w715:path)
              n627 = call <vilib>:"Check if File or Folder Exists.vi"("path"=w715) -> ("file or folder exists?"=w716:bool, "dup path"=w717:path)  [unwired: 8 in, 1 out]
              n628 = case shown="False" w716 {
                tunnel: w717 -> [w720 w722]
                frame False {
                  n629 = local write "Path SLAB #7"(w720) -> ()
                  n630 = call-poly <vilib>:"Write Delimited Spreadsheet.vi"("file path (dialog if empty)"=w720, "1D data"=string[] ["Timestamp", "Measured", "Calibrated"], "append to file? (new file:F)"=FALSE, "delimiter (\\t)"="," ("delimiter (\\t)")) -> ()  [unwired: 10 in, 2 out]
                }
                frame True {
                  n631 = local write "Path SLAB #7"(w722) -> ()
                }
              }
            }
          }
        }
        frame #9 {
          n632 = local read "Ch 10 Status"() -> (w723:bool)
          n633 = case shown="True" w723 {
            frame False {
            }
            frame True {
              # "See frame 2 for explanation"
              n634 = local read "Folder"() -> (w725:path)
              n635 = Build Path(base path=w725, name or relative path="SLAB8.csv") -> (appended path=w726:path)
              n636 = call <vilib>:"Check if File or Folder Exists.vi"("path"=w726) -> ("file or folder exists?"=w727:bool, "dup path"=w728:path)  [unwired: 8 in, 1 out]
              n637 = case shown="False" w727 {
                tunnel: w728 -> [w731 w733]
                frame False {
                  n638 = local write "Path SLAB #8"(w731) -> ()
                  n639 = call-poly <vilib>:"Write Delimited Spreadsheet.vi"("file path (dialog if empty)"=w731, "1D data"=string[] ["Timestamp", "Measured", "Calibrated"], "append to file? (new file:F)"=FALSE, "delimiter (\\t)"="," ("delimiter (\\t)")) -> ()  [unwired: 10 in, 2 out]
                }
                frame True {
                  n640 = local write "Path SLAB #8"(w733) -> ()
                }
              }
            }
          }
        }
        frame #10 {
          n641 = local read "Ch 08 Status"() -> (w734:bool)
          n642 = case shown="True" w734 {
            frame False {
            }
            frame True {
              # "See frame 2 for explanation"
              n643 = local read "Folder"() -> (w736:path)
              n644 = Build Path(base path=w736, name or relative path="SLAB9.csv") -> (appended path=w737:path)
              n645 = call <vilib>:"Check if File or Folder Exists.vi"("path"=w737) -> ("file or folder exists?"=w738:bool, "dup path"=w739:path)  [unwired: 8 in, 1 out]
              n646 = case shown="False" w738 {
                tunnel: w739 -> [w742 w744]
                frame False {
                  n647 = local write "Path SLAB #9"(w742) -> ()
                  n648 = call-poly <vilib>:"Write Delimited Spreadsheet.vi"("file path (dialog if empty)"=w742, "1D data"=string[] ["Timestamp", "Measured", "Calibrated"], "append to file? (new file:F)"=FALSE, "delimiter (\\t)"="," ("delimiter (\\t)")) -> ()  [unwired: 10 in, 2 out]
                }
                frame True {
                  n649 = local write "Path SLAB #9"(w744) -> ()
                }
              }
            }
          }
        }
        frame #11 {
          n650 = local read "Ch 09 Status"() -> (w745:bool)
          n651 = case shown="True" w745 {
            frame False {
            }
            frame True {
              # "See frame 2 for explanation"
              n652 = local read "Folder"() -> (w747:path)
              n653 = Build Path(base path=w747, name or relative path="SLAB10.csv") -> (appended path=w748:path)
              n654 = call <vilib>:"Check if File or Folder Exists.vi"("path"=w748) -> ("file or folder exists?"=w749:bool, "dup path"=w750:path)  [unwired: 8 in, 1 out]
              n655 = case shown="False" w749 {
                tunnel: w750 -> [w753 w755]
                frame False {
                  n656 = local write "Path SLAB #10"(w753) -> ()
                  n657 = call-poly <vilib>:"Write Delimited Spreadsheet.vi"("file path (dialog if empty)"=w753, "1D data"=string[] ["Timestamp", "Measured", "Calibrated"], "append to file? (new file:F)"=FALSE, "delimiter (\\t)"="," ("delimiter (\\t)")) -> ()  [unwired: 10 in, 2 out]
                }
                frame True {
                  n658 = local write "Path SLAB #10"(w755) -> ()
                }
              }
            }
          }
        }
        frame #12 {
          n659 = local read "Ch 14 Status"() -> (w756:bool)
          n660 = case shown="True" w756 {
            frame False {
            }
            frame True {
              # "Check if 1st_stage.csv exists"
              n661 = local read "Folder"() -> (w758:path)
              n662 = Build Path(base path=w758, name or relative path="1st_stage.csv") -> (appended path=w759:path)
              n663 = call <vilib>:"Check if File or Folder Exists.vi"("path"=w759) -> ("file or folder exists?"=w760:bool, "dup path"=w761:path)  [unwired: 8 in, 1 out]
              n664 = case shown="False" w760 {
                tunnel: w761 -> [w764 w766]
                frame False {
                  # "Does not exist. Create the file, \nand write a header to it"
                  n665 = local write "Path 1st stage"(w764) -> ()
                  n666 = call-poly <vilib>:"Write Delimited Spreadsheet.vi"("file path (dialog if empty)"=w764, "1D data"=string[] ["Timestamp", "Measured", "Calibrated"], "append to file? (new file:F)"=FALSE, "delimiter (\\t)"="," ("delimiter (\\t)")) -> ()  [unwired: 10 in, 2 out]
                }
                frame True {
                  # "Exists. Return File path"
                  n667 = local write "Path 1st stage"(w766) -> ()
                }
              }
            }
          }
        }
        frame #13 {
          n668 = local read "Ch 11 Status"() -> (w767:bool)
          n669 = case shown="True" w767 {
            frame False {
            }
            frame True {
              # "Check if 2nd_stage.csv exists"
              n670 = local read "Folder"() -> (w769:path)
              n671 = Build Path(base path=w769, name or relative path="2nd_stage.csv") -> (appended path=w770:path)
              n672 = call <vilib>:"Check if File or Folder Exists.vi"("path"=w770) -> ("file or folder exists?"=w771:bool, "dup path"=w772:path)  [unwired: 8 in, 1 out]
              n673 = case shown="False" w771 {
                tunnel: w772 -> [w775 w777]
                frame False {
                  # "Does not exist. Create the file, \nand write a header to it"
                  n674 = local write "Path 2nd stage"(w775) -> ()
                  n675 = call-poly <vilib>:"Write Delimited Spreadsheet.vi"("file path (dialog if empty)"=w775, "1D data"=string[] ["Timestamp", "Measured", "Calibrated"], "append to file? (new file:F)"=FALSE, "delimiter (\\t)"="," ("delimiter (\\t)")) -> ()  [unwired: 10 in, 2 out]
                }
                frame True {
                  # "Exists. Return File path"
                  n676 = local write "Path 2nd stage"(w777) -> ()
                }
              }
            }
          }
        }
        frame #14 {
          n677 = local read "Ch 12 Status"() -> (w778:bool)
          n678 = case shown="True" w778 {
            frame False {
            }
            frame True {
              # "Check if 3rd_stage.csv exists"
              n679 = local read "Folder"() -> (w780:path)
              n680 = Build Path(base path=w780, name or relative path="3rd_stage.csv") -> (appended path=w781:path)
              n681 = call <vilib>:"Check if File or Folder Exists.vi"("path"=w781) -> ("file or folder exists?"=w782:bool, "dup path"=w783:path)  [unwired: 8 in, 1 out]
              n682 = case shown="False" w782 {
                tunnel: w783 -> [w786 w788]
                frame False {
                  # "Does not exist. Create the file, \nand write a header to it"
                  n683 = local write "Path 3rd stage"(w786) -> ()
                  n684 = call-poly <vilib>:"Write Delimited Spreadsheet.vi"("file path (dialog if empty)"=w786, "1D data"=string[] ["Timestamp", "Measured", "Calibrated"], "append to file? (new file:F)"=FALSE, "delimiter (\\t)"="," ("delimiter (\\t)")) -> ()  [unwired: 10 in, 2 out]
                }
                frame True {
                  # "Exists. Return File path"
                  n685 = local write "Path 3rd stage"(w788) -> ()
                }
              }
            }
          }
        }
        frame #15 {
          n686 = local read "Ch 15 Status"() -> (w789:bool)
          n687 = case shown="True" w789 {
            frame False {
            }
            frame True {
              # "Check if 4th_stage.csv exists"
              n688 = local read "Folder"() -> (w791:path)
              n689 = Build Path(base path=w791, name or relative path="4th_stage.csv") -> (appended path=w792:path)
              n690 = call <vilib>:"Check if File or Folder Exists.vi"("path"=w792) -> ("file or folder exists?"=w793:bool, "dup path"=w794:path)  [unwired: 8 in, 1 out]
              n691 = case shown="False" w793 {
                tunnel: w794 -> [w797 w799]
                frame False {
                  # "Does not exist. Create the file, \nand write a header to it"
                  n692 = local write "Path 4th stage"(w797) -> ()
                  n693 = call-poly <vilib>:"Write Delimited Spreadsheet.vi"("file path (dialog if empty)"=w797, "1D data"=string[] ["Timestamp", "Measured", "Calibrated"], "append to file? (new file:F)"=FALSE, "delimiter (\\t)"="," ("delimiter (\\t)")) -> ()  [unwired: 10 in, 2 out]
                }
                frame True {
                  # "Exists. Return File path"
                  n694 = local write "Path 4th stage"(w799) -> ()
                }
              }
            }
          }
        }
        frame #16 {
          n695 = local read "Ch 16 Status"() -> (w800:bool)
          n696 = case shown="True" w800 {
            frame False {
            }
            frame True {
              n697 = local read "Folder"() -> (w802:path)
              n698 = Build Path(base path=w802, name or relative path="5th_stage.csv") -> (appended path=w803:path)
              n699 = call <vilib>:"Check if File or Folder Exists.vi"("path"=w803) -> ("file or folder exists?"=w804:bool, "dup path"=w805:path)  [unwired: 8 in, 1 out]
              n700 = case shown="False" w804 {
                tunnel: w805 -> [w808 w810]
                frame False {
                  # "Does not exist. Create the file, \nand write a header to it"
                  n701 = local write "Path 5th stage"(w808) -> ()
                  n702 = call-poly <vilib>:"Write Delimited Spreadsheet.vi"("file path (dialog if empty)"=w808, "1D data"=string[] ["Timestamp", "Measured", "Calibrated"], "append to file? (new file:F)"=FALSE, "delimiter (\\t)"="," ("delimiter (\\t)")) -> ()  [unwired: 10 in, 2 out]
                }
                frame True {
                  # "Exists. Return File path"
                  n703 = local write "Path 5th stage"(w810) -> ()
                }
              }
            }
          }
        }
        frame #17 {
          n704 = local read "Ch 13 Status"() -> (w811:bool)
          n705 = case shown="True" w811 {
            frame False {
            }
            frame True {
              n706 = local read "Folder"() -> (w813:path)
              n707 = Build Path(base path=w813, name or relative path="quanta-ray.csv") -> (appended path=w814:path)
              n708 = call <vilib>:"Check if File or Folder Exists.vi"("path"=w814) -> ("file or folder exists?"=w815:bool, "dup path"=w816:path)  [unwired: 8 in, 1 out]
              n709 = case shown="False" w815 {
                tunnel: w816 -> [w819 w821]
                frame False {
                  # "Does not exist. Create the file, \nand write a header to it"
                  n710 = local write "Path quanta ray"(w819) -> ()
                  n711 = call-poly <vilib>:"Write Delimited Spreadsheet.vi"("file path (dialog if empty)"=w819, "1D data"=string[] ["Timestamp", "Measured", "Calibrated"], "append to file? (new file:F)"=FALSE, "delimiter (\\t)"="," ("delimiter (\\t)")) -> ()  [unwired: 10 in, 2 out]
                }
                frame True {
                  # "Exists. Return File path"
                  n712 = local write "Path quanta ray"(w821) -> ()
                }
              }
            }
          }
        }
      }
    }
    frame #10 {
      # "Initialize Spectrometer and Run Python code"
      n713 = stacked-sequence {
        frame #0 {
          # "Initialize location of Spectrometer data"
          n714 = local read "Path Spectrometer Base"() -> (w833:path)
          n715 = local read "Date"() -> (w834:string)
          n716 = String To Path(string=w834) -> (path=w828:path)
          n717 = Build Path(base path=w833, name or relative path=w828) -> (appended path=w829:path)
          n718 = call <vilib>:"Check if File or Folder Exists.vi"("path"=w829) -> ("error out"=w831:errorcluster, "file or folder exists?"=w832:bool, "dup path"=w830:path)  [unwired: 8 in]
          n719 = case shown="False" w832 {
            tunnel: w830 -> [w845 w846]
            tunnel: w831 -> [w844 _]
            tunnel: [w843 w846] -> w824
            frame False {
              # "Doesnot exist. Create the folder"
              n720 = Create Folder(path (use dialog)=w845, error in=w844) -> (created path=w843:path)  [unwired: 1 in, 2 out]
            }
            frame True {
              # "Exist, output current path to base path"
            }
          }
          n721 = local write "Path Spectrometer Folder"(w824) -> ()
          n722 = List Folder(path=w824, pattern="*.csv") -> (filenames=w827:string[])  [unwired: 2 in, 3 out]
          n723 = Array Size(array=w827) -> (size(s)=w826:i32)
          n724 = Not Equal?(x=w826, y=0) -> (x != y?=w825:bool)
          n725 = case shown="True" w825 {
            tunnel: w827 -> [_ w838]
            tunnel: w824 -> [_ w837]
            frame False {
              n726 = String To Path(string="") -> (path=w835:path)
              n727 = local write "Path Spectrometer Data Old"(w835) -> ()
            }
            frame True {
              n728 = Reverse 1D Array(array=w838) -> (reversed array=w839:string[])
              n729 = Index Array(array=w839) -> (element=w840:string)  [unwired: 1 in]
              n730 = String To Path(string=w840) -> (path=w841:path)
              n731 = Build Path(base path=w837, name or relative path=w841) -> (appended path=w842:path)
              n732 = local write "Path Spectrometer Data Old"(w842) -> ()
            }
          }
        }
        frame #1 {
          # "Start Python server and client"
          n733 = flat-sequence {
            frame #0 {
              n734 = local read "Path Spectrometer Base"() -> (w849:path)
              n735 = Format Into String(format string="cmd /c %s\\\\run_server.bat", w849) -> (resulting string=w848:string)  [unwired: 2 in, 1 out]
              n736 = call <vilib>:"System Exec.vi"("run minimized? (F)"=FALSE, "wait until completion? (T)"=FALSE, "command line"=w848) -> ()  [unwired: 5 in, 4 out]
            }
            frame #1 {
              n737 = local read "Path Spectrometer Base"() -> (w853:path)
              n738 = Format Into String(format string="cmd /c %s\\\\run_client.bat", w853) -> (resulting string=w855:string)  [unwired: 2 in, 1 out]
              n739 = call <vilib>:"System Exec.vi"("run minimized? (F)"=FALSE, "wait until completion? (T)"=FALSE, "command line"=w855) -> ()  [unwired: 5 in, 4 out]
            }
          }
        }
      }
    }
    frame #11 {
      n740 = shared-variable "My Computer\\Server Library.lvlib\\timeStamp"("") -> ()  [unwired: 1 in, 1 out]
      n741 = shared-variable "My Computer\\Server Library.lvlib\\slab7"(0) -> ()  [unwired: 1 in, 1 out]
      n742 = shared-variable "My Computer\\Server Library.lvlib\\slab5"(0) -> ()  [unwired: 1 in, 1 out]
      n743 = shared-variable "My Computer\\Server Library.lvlib\\slab4"(0) -> ()  [unwired: 1 in, 1 out]
      n744 = shared-variable "My Computer\\Server Library.lvlib\\slab2"(0) -> ()  [unwired: 1 in, 1 out]
      n745 = shared-variable "My Computer\\Server Library.lvlib\\slab3"(0) -> ()  [unwired: 1 in, 1 out]
      n746 = shared-variable "My Computer\\Server Library.lvlib\\QuantaRay"(0) -> ()  [unwired: 1 in, 1 out]
      n747 = shared-variable "My Computer\\Server Library.lvlib\\frontend2"(0) -> ()  [unwired: 1 in, 1 out]
      n748 = shared-variable "My Computer\\Server Library.lvlib\\frontend1"(0) -> ()  [unwired: 1 in, 1 out]
      n749 = shared-variable "My Computer\\Server Library.lvlib\\stage5"(0) -> ()  [unwired: 1 in, 1 out]
      n750 = shared-variable "My Computer\\Server Library.lvlib\\stage4"(0) -> ()  [unwired: 1 in, 1 out]
      n751 = shared-variable "My Computer\\Server Library.lvlib\\stage3"(0) -> ()  [unwired: 1 in, 1 out]
      n752 = shared-variable "My Computer\\Server Library.lvlib\\stage1"(0) -> ()  [unwired: 1 in, 1 out]
      n753 = shared-variable "My Computer\\Server Library.lvlib\\stage2"(0) -> ()  [unwired: 1 in, 1 out]
      n754 = shared-variable "My Computer\\Server Library.lvlib\\slab10"(0) -> ()  [unwired: 1 in, 1 out]
      n755 = shared-variable "My Computer\\Server Library.lvlib\\slab9"(0) -> ()  [unwired: 1 in, 1 out]
      n756 = shared-variable "My Computer\\Server Library.lvlib\\slab8"(0) -> ()  [unwired: 1 in, 1 out]
    }
  }
  n757 = while {
    tunnel: w16 -> [w914]
    tunnel: [w914] -> w15
    tunnel: w14 -> [w882]
    tunnel: [w882] -> w7
    tunnel: [w881] -> w6
    tunnel: w13 -> [w881]
    tunnel: w12 -> [w880]
    tunnel: [w880] -> w5
    tunnel: [w879] -> w4
    tunnel: w11 -> [w879]
    tunnel: w10 -> [w878]
    tunnel: w9 -> [w877]
    tunnel: w8 -> [w876]
    tunnel: [w878] -> w3
    tunnel: [w877] -> w2
    tunnel: [w876] -> w1
    stop <- w917 continue-if-true
    # "Command control for Com Port 3, details see com port 1"
    # "Command control for Com Port 2, details see com port 1"
    # "Command control for Com Port 1\n (command control for other com ports is the same as this one, need to create new variables)"
    # "If clicked, send the corresponding command\nto slink, and then return ch1 and ch2 status"
    # "Click scale down, and return channel status"
    # "Click scale up, and return channel status"
    # "Each Frame is  a s-link, containing two channels.\nif more slink needs to be added, just copy a frame after the last frame, create new varibles for each slink \nAnd also copy scale up/down and send command frames (5 frames) for each s-link being created."
    # "Check if date changes"
    # "Get Current time"
    n758 = stacked-sequence {
      tunnel: w914 -> [w976 _ _ _ _ _ _ _ _ _]
      tunnel: w882 -> [_ w1029 _ _ _ _ _ _ _ _]
      tunnel: w881 -> [_ _ w1082 _ _ _ _ _ _ _]
      tunnel: w880 -> [_ _ _ w1135 _ _ _ _ _ _]
      tunnel: w879 -> [_ _ _ _ w1188 _ _ _ _ _]
      tunnel: w878 -> [_ _ _ _ _ w1241 _ _ _ _]
      tunnel: w877 -> [_ _ _ _ _ _ w1296 _ _ _]
      tunnel: w876 -> [_ _ _ _ _ _ _ w1353 _ _]
      frame #0 {
        n759 = local read "Ch 02 Status"() -> (w971:bool)
        n760 = local read "Ch 01 Status"() -> (w970:bool)
        n761 = call "Read.vi"("Ch2 Status"=w971, "Com Port"=w976, "Ch1 Status"=w970) -> ("Ch 2 out"=w973:dbl, "Ch 1 out"=w972:dbl)
        n762 = Equal To 0?(x=w973) -> (x = 0?=w974:bool)
        n763 = Equal To 0?(x=w972) -> (x = 0?=w975:bool)
        n764 = case shown="False" w975 {
          tunnel: w972 -> [w1001 _]
          frame False {
            # "Compare with threshold"
            # "Output data to Chart and Numerical block"
            # "Ch1 get data from the meter"
            n765 = Multiply(x=w1001, y="Factor 1") -> (x*y=w1000:T3)
            n766 = local read "Threshold IR 1"() -> (w1005:dbl)
            n767 = shared-variable "My Computer\\Server Library.lvlib\\frontend1"(w1000) -> ()  [unwired: 1 in, 1 out]
            n768 = local write "Measure 1"(w1001) -> ()
            n769 = Greater Or Equal?(x=w1000, y=w1005) -> (x >= y?=w1006:bool)
            n770 = local write "Ch 1"(w1000) -> ()
            n771 = case shown="True" w1006 {
              tunnel: w1000 -> [w1019 _]
              frame False {
                # "compare with threshold 2"
                n772 = local read "Threshold IR 2"() -> (w1018:dbl)
                n773 = Less?(x=w1019, y=w1018) -> (x < y?=w1017:bool)
                n774 = case shown="False" w1017 {
                  frame False {
                    w1020 = cluster{u32, u32}[] [{1985280, 0}, {16769536, 0}] ("Colors [4]")
                    # "More than threhold 2\nLED turn to yellow"
                    n775 = property on="Ch 01 Status" class="Bool (strict)"("Colors [4]"=w1020) -> ()  [unwired: 2 in, 2 out]
                    n776 = property on="Ch 01 Status 2" class="Bool (strict)"("Colors [4]"=w1020) -> ()  [unwired: 2 in, 2 out]
                  }
                  frame True {
                    w1021 = cluster{u32, u32}[] [{1985280, 0}, {16722474, 0}] ("Colors [4]")
                    # "Less than threhold 2\nLED turn to red"
                    n777 = property on="Ch 01 Status" class="Bool (strict)"("Colors [4]"=w1021) -> ()  [unwired: 2 in, 2 out]
                    n778 = property on="Ch 01 Status 2" class="Bool (strict)"("Colors [4]"=w1021) -> ()  [unwired: 2 in, 2 out]
                  }
                }
              }
              frame True {
                w1022 = cluster{u32, u32}[] [{1985280, 0}, {6618880, 0}] ("Colors [4]")
                # "More the threshold 1\nLED turns to green"
                n779 = property on="Ch 01 Status" class="Bool (strict)"("Colors [4]"=w1022) -> ()  [unwired: 2 in, 2 out]
                n780 = property on="Ch 01 Status 2" class="Bool (strict)"("Colors [4]"=w1022) -> ()  [unwired: 2 in, 2 out]
              }
            }
            n781 = local read "Save Next shot to File?"() -> (w1004:bool)
            n782 = Multiply(x=w1001, y=1.0) -> (x*y=w1003:dbl)
            n783 = case shown="True" w1004 {
              tunnel: w1003 -> [_ w1011]
              tunnel: w1000 -> [_ w1010]
              frame False {
              }
              frame True {
                # "Save original and calibrated data with time into the file"
                n784 = call "string_to_formated_string.vi"("Numeric"=w1010) -> ("String"=w1009:string)  [unwired: 1 in]
                n785 = call "string_to_formated_string.vi"("Numeric"=w1011) -> ("String"=w1008:string)  [unwired: 1 in]
                n786 = local read "Time"() -> (w1016:string)
                n787 = local read "Path Frontend #1"() -> (w1015:path)
                n788 = Build Array(w1016, w1008, w1009) -> (w1014:string[])
                n789 = call-poly <vilib>:"Write Delimited Spreadsheet.vi"("file path (dialog if empty)"=w1015, "1D data"=w1014, "append to file? (new file:F)"=TRUE ("transpose? (no:F)"), "delimiter (\\t)"="," ("delimiter (\\t)")) -> ()  [unwired: 10 in, 2 out]
              }
            }
          }
          frame True {
            # "No data from meters"
          }
        }
        n790 = case shown="False" w974 {
          tunnel: w973 -> [w978 _]
          frame False {
            # "Details see above"
            # "Ch2 get data from the meter"
            n791 = local write "Measure 2"(w978) -> ()
            n792 = Multiply(x=w978, y="Factor 2") -> (x*y=w977:T3)
            n793 = shared-variable "My Computer\\Server Library.lvlib\\frontend2"(w977) -> ()  [unwired: 1 in, 1 out]
            n794 = local read "Threshold IR 1"() -> (w983:dbl)
            n795 = Greater Or Equal?(x=w977, y=w983) -> (x >= y?=w982:bool)
            n796 = local write "Ch 2"(w977) -> ()
            n797 = case shown="True" w982 {
              tunnel: w977 -> [w996 _]
              frame False {
                n798 = local read "Threshold IR 2"() -> (w995:dbl)
                n799 = Less?(x=w996, y=w995) -> (x < y?=w994:bool)
                n800 = case shown="True" w994 {
                  frame False {
                    w997 = cluster{u32, u32}[] [{1985280, 0}, {16769536, 0}] ("Colors [4]")
                    n801 = property on="Ch 02 Status" class="Bool (strict)"("Colors [4]"=w997) -> ()  [unwired: 2 in, 2 out]
                    n802 = property on="Ch 02 Status 2" class="Bool (strict)"("Colors [4]"=w997) -> ()  [unwired: 2 in, 2 out]
                  }
                  frame True {
                    w998 = cluster{u32, u32}[] [{1985280, 0}, {16722474, 0}] ("Colors [4]")
                    n803 = property on="Ch 02 Status 2" class="Bool (strict)"("Colors [4]"=w998) -> ()  [unwired: 2 in, 2 out]
                    n804 = property on="Ch 02 Status" class="Bool (strict)"("Colors [4]"=w998) -> ()  [unwired: 2 in, 2 out]
                  }
                }
              }
              frame True {
                w999 = cluster{u32, u32}[] [{1985280, 0}, {6618880, 0}] ("Colors [4]")
                n805 = property on="Ch 02 Status" class="Bool (strict)"("Colors [4]"=w999) -> ()  [unwired: 2 in, 2 out]
                n806 = property on="Ch 02 Status 2" class="Bool (strict)"("Colors [4]"=w999) -> ()  [unwired: 2 in, 2 out]
              }
            }
            n807 = Multiply(x=w978, y=1.0) -> (x*y=w979:dbl)
            n808 = local read "Save Next shot to File?"() -> (w981:bool)
            n809 = case shown="True" w981 {
              tunnel: w977 -> [_ w993]
              tunnel: w979 -> [_ w992]
              frame False {
              }
              frame True {
                n810 = local read "Time"() -> (w991:string)
                n811 = call "string_to_formated_string.vi"("Numeric"=w993) -> ("String"=w986:string)  [unwired: 1 in]
                n812 = call "string_to_formated_string.vi"("Numeric"=w992) -> ("String"=w985:string)  [unwired: 1 in]
                n813 = local read "Path Frontend #2"() -> (w988:path)
                n814 = Build Array(w991, w985, w986) -> (w987:string[])
                n815 = call-poly <vilib>:"Write Delimited Spreadsheet.vi"("file path (dialog if empty)"=w988, "1D data"=w987, "append to file? (new file:F)"=TRUE, "delimiter (\\t)"="," ("delimiter (\\t)")) -> ()  [unwired: 10 in, 2 out]
              }
            }
          }
          frame True {
            # "No data from meters"
          }
        }
      }
      frame #1 {
        n816 = local read "Ch 04 Status"() -> (w1023:bool)
        n817 = local read "Ch 03 Status"() -> (w1024:bool)
        n818 = call "Read.vi"("Ch2 Status"=w1023, "Com Port"=w1029, "Ch1 Status"=w1024) -> ("Ch 2 out"=w1026:dbl, "Ch 1 out"=w1025:dbl)
        n819 = Equal To 0?(x=w1026) -> (x = 0?=w1028:bool)
        n820 = Equal To 0?(x=w1025) -> (x = 0?=w1027:bool)
        n821 = case shown="False" w1027 {
          tunnel: w1025 -> [w1054 _]
          frame False {
            n822 = local write "Measure 3"(w1054) -> ()
            n823 = local read "Threshold Green 1"() -> (w1059:dbl)
            n824 = Multiply(x=w1054, y="Factor 3") -> (x*y=w1053:T3)
            n825 = local write "Ch 3"(w1053) -> ()
            n826 = Greater Or Equal?(x=w1053, y=w1059) -> (x >= y?=w1058:bool)
            n827 = shared-variable "My Computer\\Server Library.lvlib\\slab2"(w1053) -> ()  [unwired: 1 in, 1 out]
            n828 = case shown="True" w1058 {
              tunnel: w1053 -> [w1072 _]
              frame False {
                n829 = local read "Threshold Green 2"() -> (w1071:dbl)
                n830 = Less?(x=w1072, y=w1071) -> (x < y?=w1070:bool)
                n831 = case shown="False" w1070 {
                  frame False {
                    n832 = property on="Ch 03 Status" class="Bool (strict)"("Colors [4]"=cluster{u32, u32}[] [{1985280, 0}, {16769536, 0}]) -> ()  [unwired: 2 in, 2 out]
                  }
                  frame True {
                    n833 = property on="Ch 03 Status" class="Bool (strict)"("Colors [4]"=cluster{u32, u32}[] [{1985280, 0}, {16722474, 0}]) -> ()  [unwired: 2 in, 2 out]
                  }
                }
              }
              frame True {
                w1075 = cluster{u32, u32}[] [{1985280, 0}, {6618880, 0}] ("Colors [4]")
                n834 = property on="Ch 03 Status" class="Bool (strict)"("Colors [4]"=w1075) -> ()  [unwired: 2 in, 2 out]
                n835 = property on="Ch 03 Status 2" class="Bool (strict)"("Colors [4]"=w1075) -> ()  [unwired: 2 in, 2 out]
              }
            }
            n836 = Multiply(x=w1054, y=1.0) -> (x*y=w1055:dbl)
            n837 = local read "Save Next shot to File?"() -> (w1057:bool)
            n838 = case shown="True" w1057 {
              tunnel: w1053 -> [_ w1069]
              tunnel: w1055 -> [_ w1061]
              frame False {
              }
              frame True {
                n839 = call "string_to_formated_string.vi"("Numeric"=w1069) -> ("String"=w1064:string)  [unwired: 1 in]
                n840 = call "string_to_formated_string.vi"("Numeric"=w1061) -> ("String"=w1062:string)  [unwired: 1 in]
                n841 = local read "Time"() -> (w1068:string)
                n842 = local read "Path SLAB #2"() -> (w1067:path)
                n843 = Build Array(w1068, w1062, w1064) -> (w1063:string[])
                n844 = call-poly <vilib>:"Write Delimited Spreadsheet.vi"("file path (dialog if empty)"=w1067, "1D data"=w1063, "append to file? (new file:F)"=TRUE, "delimiter (\\t)"="," ("delimiter (\\t)")) -> ()  [unwired: 10 in, 2 out]
              }
            }
          }
          frame True {
          }
        }
        n845 = case shown="False" w1028 {
          tunnel: w1026 -> [w1031 _]
          frame False {
            n846 = local write "Measure 4"(w1031) -> ()
            n847 = local read "Threshold Green 1"() -> (w1036:dbl)
            n848 = Multiply(x=w1031, y="Factor 4") -> (x*y=w1030:T3)
            n849 = Multiply(x=w1031, y=1.0) -> (x*y=w1032:dbl)
            n850 = local write "Ch 4"(w1030) -> ()
            n851 = shared-variable "My Computer\\Server Library.lvlib\\slab4"(w1030) -> ()  [unwired: 1 in, 1 out]
            n852 = Greater Or Equal?(x=w1030, y=w1036) -> (x >= y?=w1035:bool)
            n853 = case shown="False" w1035 {
              tunnel: w1030 -> [w1049 _]
              frame False {
                n854 = local read "Threshold Green 2"() -> (w1048:dbl)
                n855 = Less?(x=w1049, y=w1048) -> (x < y?=w1047:bool)
                n856 = case shown="True" w1047 {
                  frame False {
                    w1050 = cluster{u32, u32}[] [{1985280, 0}, {16769536, 0}] ("Colors [4]")
                    n857 = property on="Ch 04 Status 2" class="Bool (strict)"("Colors [4]"=w1050) -> ()  [unwired: 2 in, 2 out]
                    n858 = property on="Ch 04 Status" class="Bool (strict)"("Colors [4]"=w1050) -> ()  [unwired: 2 in, 2 out]
                  }
                  frame True {
                    w1051 = cluster{u32, u32}[] [{1985280, 0}, {16722474, 0}] ("Colors [4]")
                    n859 = property on="Ch 04 Status 2" class="Bool (strict)"("Colors [4]"=w1051) -> ()  [unwired: 2 in, 2 out]
                    n860 = property on="Ch 04 Status" class="Bool (strict)"("Colors [4]"=w1051) -> ()  [unwired: 2 in, 2 out]
                  }
                }
              }
              frame True {
                w1052 = cluster{u32, u32}[] [{1985280, 0}, {6618880, 0}] ("Colors [4]")
                n861 = property on="Ch 04 Status" class="Bool (strict)"("Colors [4]"=w1052) -> ()  [unwired: 2 in, 2 out]
                n862 = property on="Ch 04 Status 2" class="Bool (strict)"("Colors [4]"=w1052) -> ()  [unwired: 2 in, 2 out]
              }
            }
            n863 = local read "Save Next shot to File?"() -> (w1034:bool)
            n864 = case shown="True" w1034 {
              tunnel: w1030 -> [_ w1038]
              tunnel: w1032 -> [_ w1039]
              frame False {
              }
              frame True {
                n865 = call "string_to_formated_string.vi"("Numeric"=w1038) -> ("String"=w1042:string)  [unwired: 1 in]
                n866 = call "string_to_formated_string.vi"("Numeric"=w1039) -> ("String"=w1041:string)  [unwired: 1 in]
                n867 = local read "Time"() -> (w1045:string)
                n868 = Build Array(w1045, w1041, w1042) -> (w1040:string[])
                n869 = local read "Path SLAB #4"() -> (w1046:path)
                n870 = call-poly <vilib>:"Write Delimited Spreadsheet.vi"("file path (dialog if empty)"=w1046, "1D data"=w1040, "append to file? (new file:F)"=TRUE, "delimiter (\\t)"="," ("delimiter (\\t)")) -> ()  [unwired: 10 in, 2 out]
              }
            }
          }
          frame True {
          }
        }
      }
      frame #2 {
        n871 = local read "Ch 05 Status"() -> (w1076:bool)
        n872 = local read "Ch 06 Status"() -> (w1077:bool)
        n873 = call "Read.vi"("Ch2 Status"=w1077, "Com Port"=w1082, "Ch1 Status"=w1076) -> ("Ch 2 out"=w1079:dbl, "Ch 1 out"=w1078:dbl)
        n874 = Equal To 0?(x=w1079) -> (x = 0?=w1081:bool)
        n875 = Equal To 0?(x=w1078) -> (x = 0?=w1080:bool)
        n876 = case shown="False" w1081 {
          tunnel: w1079 -> [w1084 _]
          frame False {
            n877 = local write "Measure 6"(w1084) -> ()
            n878 = local read "Threshold Green 1"() -> (w1089:dbl)
            n879 = Multiply(x=w1084, y="Factor 6") -> (x*y=w1083:T3)
            n880 = Multiply(x=w1084, y=1.0) -> (x*y=w1085:dbl)
            n881 = Greater Or Equal?(x=w1083, y=w1089) -> (x >= y?=w1088:bool)
            n882 = local write "Ch 6"(w1083) -> ()
            n883 = shared-variable "My Computer\\Server Library.lvlib\\slab3"(w1083) -> ()  [unwired: 1 in, 1 out]
            n884 = case shown="False" w1088 {
              tunnel: w1083 -> [w1102 _]
              frame False {
                n885 = local read "Threshold Green 2"() -> (w1101:dbl)
                n886 = Less?(x=w1102, y=w1101) -> (x < y?=w1100:bool)
                n887 = case shown="False" w1100 {
                  frame False {
                    w1103 = cluster{u32, u32}[] [{1985280, 0}, {16769536, 0}] ("Colors [4]")
                    n888 = property on="Ch 06 Status 2" class="Bool (strict)"("Colors [4]"=w1103) -> ()  [unwired: 2 in, 2 out]
                    n889 = property on="Ch 06 Status" class="Bool (strict)"("Colors [4]"=w1103) -> ()  [unwired: 2 in, 2 out]
                  }
                  frame True {
                    w1104 = cluster{u32, u32}[] [{1985280, 0}, {16722474, 0}] ("Colors [4]")
                    n890 = property on="Ch 06 Status" class="Bool (strict)"("Colors [4]"=w1104) -> ()  [unwired: 2 in, 2 out]
                    n891 = property on="Ch 06 Status 2" class="Bool (strict)"("Colors [4]"=w1104) -> ()  [unwired: 2 in, 2 out]
                  }
                }
              }
              frame True {
                w1105 = cluster{u32, u32}[] [{1985280, 0}, {6618880, 0}] ("Colors [4]")
                n892 = property on="Ch 06 Status" class="Bool (strict)"("Colors [4]"=w1105) -> ()  [unwired: 2 in, 2 out]
                n893 = property on="Ch 06 Status 2" class="Bool (strict)"("Colors [4]"=w1105) -> ()  [unwired: 2 in, 2 out]
              }
            }
            n894 = local read "Save Next shot to File?"() -> (w1087:bool)
            n895 = case shown="True" w1087 {
              tunnel: w1083 -> [_ w1092]
              tunnel: w1085 -> [_ w1091]
              frame False {
              }
              frame True {
                n896 = call "string_to_formated_string.vi"("Numeric"=w1092) -> ("String"=w1095:string)  [unwired: 1 in]
                n897 = call "string_to_formated_string.vi"("Numeric"=w1091) -> ("String"=w1093:string)  [unwired: 1 in]
                n898 = local read "Time"() -> (w1098:string)
                n899 = Build Array(w1098, w1093, w1095) -> (w1094:string[])
                n900 = local read "Path SLAB #3"() -> (w1099:path)
                n901 = call-poly <vilib>:"Write Delimited Spreadsheet.vi"("file path (dialog if empty)"=w1099, "1D data"=w1094, "append to file? (new file:F)"=TRUE, "delimiter (\\t)"="," ("delimiter (\\t)")) -> ()  [unwired: 10 in, 2 out]
              }
            }
          }
          frame True {
          }
        }
        n902 = case shown="False" w1080 {
          tunnel: w1078 -> [w1107 _]
          frame False {
            n903 = local write "Measure 5"(w1107) -> ()
            n904 = local read "Threshold Green 1"() -> (w1112:dbl)
            n905 = Multiply(x=w1107, y="Factor 5") -> (x*y=w1106:T3)
            n906 = Multiply(x=w1107, y=1.0) -> (x*y=w1108:dbl)
            n907 = local write "Ch 5"(w1106) -> ()
            n908 = shared-variable "My Computer\\Server Library.lvlib\\slab5"(w1106) -> ()  [unwired: 1 in, 1 out]
            n909 = Greater Or Equal?(x=w1106, y=w1112) -> (x >= y?=w1111:bool)
            n910 = case shown="False" w1111 {
              tunnel: w1106 -> [w1125 _]
              frame False {
                n911 = local read "Threshold Green 2"() -> (w1124:dbl)
                n912 = Less?(x=w1125, y=w1124) -> (x < y?=w1123:bool)
                n913 = case shown="True" w1123 {
                  frame False {
                    w1126 = cluster{u32, u32}[] [{1985280, 0}, {16769536, 0}] ("Colors [4]")
                    n914 = property on="Ch 05 Status 2" class="Bool (strict)"("Colors [4]"=w1126) -> ()  [unwired: 2 in, 2 out]
                    n915 = property on="Ch 05 Status" class="Bool (strict)"("Colors [4]"=w1126) -> ()  [unwired: 2 in, 2 out]
                  }
                  frame True {
                    w1127 = cluster{u32, u32}[] [{1985280, 0}, {16722474, 0}] ("Colors [4]")
                    n916 = property on="Ch 05 Status 2" class="Bool (strict)"("Colors [4]"=w1127) -> ()  [unwired: 2 in, 2 out]
                    n917 = property on="Ch 05 Status" class="Bool (strict)"("Colors [4]"=w1127) -> ()  [unwired: 2 in, 2 out]
                  }
                }
              }
              frame True {
                w1128 = cluster{u32, u32}[] [{1985280, 0}, {6618880, 0}] ("Colors [4]")
                n918 = property on="Ch 05 Status" class="Bool (strict)"("Colors [4]"=w1128) -> ()  [unwired: 2 in, 2 out]
                n919 = property on="Ch 05 Status 2" class="Bool (strict)"("Colors [4]"=w1128) -> ()  [unwired: 2 in, 2 out]
              }
            }
            n920 = local read "Save Next shot to File?"() -> (w1110:bool)
            n921 = case shown="True" w1110 {
              tunnel: w1106 -> [_ w1115]
              tunnel: w1108 -> [_ w1114]
              frame False {
              }
              frame True {
                n922 = call "string_to_formated_string.vi"("Numeric"=w1115) -> ("String"=w1118:string)  [unwired: 1 in]
                n923 = call "string_to_formated_string.vi"("Numeric"=w1114) -> ("String"=w1116:string)  [unwired: 1 in]
                n924 = local read "Time"() -> (w1121:string)
                n925 = Build Array(w1121, w1116, w1118) -> (w1117:string[])
                n926 = local read "Path SLAB #5"() -> (w1122:path)
                n927 = call-poly <vilib>:"Write Delimited Spreadsheet.vi"("file path (dialog if empty)"=w1122, "1D data"=w1117, "append to file? (new file:F)"=TRUE, "delimiter (\\t)"="," ("delimiter (\\t)")) -> ()  [unwired: 10 in, 2 out]
              }
            }
          }
          frame True {
          }
        }
      }
      frame #3 {
        n928 = local read "Ch 07 Status"() -> (w1129:bool)
        n929 = local read "Ch 08 Status"() -> (w1130:bool)
        n930 = call "Read.vi"("Ch2 Status"=w1130, "Com Port"=w1135, "Ch1 Status"=w1129) -> ("Ch 2 out"=w1132:dbl, "Ch 1 out"=w1131:dbl)
        n931 = Equal To 0?(x=w1132) -> (x = 0?=w1134:bool)
        n932 = Equal To 0?(x=w1131) -> (x = 0?=w1133:bool)
        n933 = case shown="False" w1133 {
          tunnel: w1131 -> [w1160 _]
          frame False {
            n934 = local write "Measure 7"(w1160) -> ()
            n935 = Multiply(x=w1160, y="Factor 7") -> (x*y=w1159:T3)
            n936 = local read "Threshold Green 1"() -> (w1165:dbl)
            n937 = Multiply(x=w1160, y=1.0) -> (x*y=w1161:dbl)
            n938 = shared-variable "My Computer\\Server Library.lvlib\\slab7"(w1159) -> ()  [unwired: 1 in, 1 out]
            n939 = local write "Ch 7"(w1159) -> ()
            n940 = Greater Or Equal?(x=w1159, y=w1165) -> (x >= y?=w1164:bool)
            n941 = case shown="False" w1164 {
              tunnel: w1159 -> [w1178 _]
              frame False {
                n942 = local read "Threshold Green 2"() -> (w1177:dbl)
                n943 = Less?(x=w1178, y=w1177) -> (x < y?=w1176:bool)
                n944 = case shown="True" w1176 {
                  frame False {
                    w1179 = cluster{u32, u32}[] [{1985280, 0}, {16769536, 0}] ("Colors [4]")
                    n945 = property on="Ch 07 Status" class="Bool (strict)"("Colors [4]"=w1179) -> ()  [unwired: 2 in, 2 out]
                    n946 = property on="Ch 07 Status 2" class="Bool (strict)"("Colors [4]"=w1179) -> ()  [unwired: 2 in, 2 out]
                  }
                  frame True {
                    w1180 = cluster{u32, u32}[] [{1985280, 0}, {16722474, 0}] ("Colors [4]")
                    n947 = property on="Ch 07 Status 2" class="Bool (strict)"("Colors [4]"=w1180) -> ()  [unwired: 2 in, 2 out]
                    n948 = property on="Ch 07 Status" class="Bool (strict)"("Colors [4]"=w1180) -> ()  [unwired: 2 in, 2 out]
                  }
                }
              }
              frame True {
                w1181 = cluster{u32, u32}[] [{1985280, 0}, {6618880, 0}] ("Colors [4]")
                n949 = property on="Ch 07 Status" class="Bool (strict)"("Colors [4]"=w1181) -> ()  [unwired: 2 in, 2 out]
                n950 = property on="Ch 07 Status 2" class="Bool (strict)"("Colors [4]"=w1181) -> ()  [unwired: 2 in, 2 out]
              }
            }
            n951 = local read "Save Next shot to File?"() -> (w1163:bool)
            n952 = case shown="True" w1163 {
              tunnel: w1159 -> [_ w1167]
              tunnel: w1161 -> [_ w1168]
              frame False {
              }
              frame True {
                n953 = call "string_to_formated_string.vi"("Numeric"=w1168) -> ("String"=w1169:string)  [unwired: 1 in]
                n954 = call "string_to_formated_string.vi"("Numeric"=w1167) -> ("String"=w1171:string)  [unwired: 1 in]
                n955 = local read "Time"() -> (w1174:string)
                n956 = Build Array(w1174, w1169, w1171) -> (w1170:string[])
                n957 = local read "Path SLAB #7"() -> (w1175:path)
                n958 = call-poly <vilib>:"Write Delimited Spreadsheet.vi"("file path (dialog if empty)"=w1175, "1D data"=w1170, "append to file? (new file:F)"=TRUE, "delimiter (\\t)"="," ("delimiter (\\t)")) -> ()  [unwired: 10 in, 2 out]
              }
            }
          }
          frame True {
          }
        }
        n959 = case shown="False" w1134 {
          tunnel: w1132 -> [w1137 _]
          frame False {
            n960 = local read "Threshold Green 1"() -> (w1142:dbl)
            n961 = local write "Measure 8"(w1137) -> ()
            n962 = Multiply(x=w1137, y="Factor 8") -> (x*y=w1136:T3)
            n963 = Multiply(x=w1137, y=1.0) -> (x*y=w1138:dbl)
            n964 = Greater Or Equal?(x=w1136, y=w1142) -> (x >= y?=w1141:bool)
            n965 = shared-variable "My Computer\\Server Library.lvlib\\slab9"(w1136) -> ()  [unwired: 1 in, 1 out]
            n966 = local write "Ch 8"(w1136) -> ()
            n967 = case shown="False" w1141 {
              tunnel: w1136 -> [w1155 _]
              frame False {
                n968 = local read "Threshold Green 2"() -> (w1154:dbl)
                n969 = Less?(x=w1155, y=w1154) -> (x < y?=w1153:bool)
                n970 = case shown="True" w1153 {
                  frame False {
                    w1156 = cluster{u32, u32}[] [{1985280, 0}, {16769536, 0}] ("Colors [4]")
                    n971 = property on="Ch 08 Status" class="Bool (strict)"("Colors [4]"=w1156) -> ()  [unwired: 2 in, 2 out]
                    n972 = property on="Ch 08 Status 2" class="Bool (strict)"("Colors [4]"=w1156) -> ()  [unwired: 2 in, 2 out]
                  }
                  frame True {
                    w1157 = cluster{u32, u32}[] [{1985280, 0}, {16722474, 0}] ("Colors [4]")
                    n973 = property on="Ch 08 Status" class="Bool (strict)"("Colors [4]"=w1157) -> ()  [unwired: 2 in, 2 out]
                    n974 = property on="Ch 08 Status 2" class="Bool (strict)"("Colors [4]"=w1157) -> ()  [unwired: 2 in, 2 out]
                  }
                }
              }
              frame True {
                w1158 = cluster{u32, u32}[] [{1985280, 0}, {6618880, 0}] ("Colors [4]")
                n975 = property on="Ch 08 Status" class="Bool (strict)"("Colors [4]"=w1158) -> ()  [unwired: 2 in, 2 out]
                n976 = property on="Ch 08 Status 2" class="Bool (strict)"("Colors [4]"=w1158) -> ()  [unwired: 2 in, 2 out]
              }
            }
            n977 = local read "Save Next shot to File?"() -> (w1140:bool)
            n978 = case shown="True" w1140 {
              tunnel: w1136 -> [_ w1145]
              tunnel: w1138 -> [_ w1144]
              frame False {
              }
              frame True {
                n979 = call "string_to_formated_string.vi"("Numeric"=w1145) -> ("String"=w1148:string)  [unwired: 1 in]
                n980 = call "string_to_formated_string.vi"("Numeric"=w1144) -> ("String"=w1147:string)  [unwired: 1 in]
                n981 = local read "Time"() -> (w1152:string)
                n982 = Build Array(w1152, w1147, w1148) -> (w1146:string[])
                n983 = local read "Path SLAB #9"() -> (w1151:path)
                n984 = call-poly <vilib>:"Write Delimited Spreadsheet.vi"("file path (dialog if empty)"=w1151, "1D data"=w1146, "append to file? (new file:F)"=TRUE, "delimiter (\\t)"="," ("delimiter (\\t)")) -> ()  [unwired: 10 in, 2 out]
              }
            }
          }
          frame True {
          }
        }
      }
      frame #4 {
        n985 = local read "Ch 09 Status"() -> (w1182:bool)
        n986 = local read "Ch 10 Status"() -> (w1183:bool)
        n987 = call "Read.vi"("Ch2 Status"=w1183, "Com Port"=w1188, "Ch1 Status"=w1182) -> ("Ch 2 out"=w1184:dbl, "Ch 1 out"=w1185:dbl)
        n988 = Equal To 0?(x=w1184) -> (x = 0?=w1187:bool)
        n989 = Equal To 0?(x=w1185) -> (x = 0?=w1186:bool)
        n990 = case shown="False" w1187 {
          tunnel: w1184 -> [w1190 _]
          frame False {
            n991 = local write "Measure 10"(w1190) -> ()
            n992 = local read "Threshold Green 1"() -> (w1195:dbl)
            n993 = Multiply(x=w1190, y=1.0) -> (x*y=w1191:dbl)
            n994 = Multiply(x=w1190, y="Factor 10") -> (x*y=w1189:T3)
            n995 = shared-variable "My Computer\\Server Library.lvlib\\slab8"(w1189) -> ()  [unwired: 1 in, 1 out]
            n996 = Greater Or Equal?(x=w1189, y=w1195) -> (x >= y?=w1194:bool)
            n997 = local write "Ch 10"(w1189) -> ()
            n998 = case shown="False" w1194 {
              tunnel: w1189 -> [w1208 _]
              frame False {
                n999 = local read "Threshold Green 2"() -> (w1207:dbl)
                n1000 = Less?(x=w1208, y=w1207) -> (x < y?=w1206:bool)
                n1001 = case shown="True" w1206 {
                  frame False {
                    w1209 = cluster{u32, u32}[] [{1985280, 0}, {16769536, 0}] ("Colors [4]")
                    n1002 = property on="Ch 10 Status 2" class="Bool (strict)"("Colors [4]"=w1209) -> ()  [unwired: 2 in, 2 out]
                    n1003 = property on="Ch 10 Status" class="Bool (strict)"("Colors [4]"=w1209) -> ()  [unwired: 2 in, 2 out]
                  }
                  frame True {
                    w1210 = cluster{u32, u32}[] [{1985280, 0}, {16722474, 0}] ("Colors [4]")
                    n1004 = property on="Ch 10 Status" class="Bool (strict)"("Colors [4]"=w1210) -> ()  [unwired: 2 in, 2 out]
                    n1005 = property on="Ch 10 Status 2" class="Bool (strict)"("Colors [4]"=w1210) -> ()  [unwired: 2 in, 2 out]
                  }
                }
              }
              frame True {
                w1211 = cluster{u32, u32}[] [{1985280, 0}, {6618880, 0}] ("Colors [4]")
                n1006 = property on="Ch 10 Status 2" class="Bool (strict)"("Colors [4]"=w1211) -> ()  [unwired: 2 in, 2 out]
                n1007 = property on="Ch 10 Status" class="Bool (strict)"("Colors [4]"=w1211) -> ()  [unwired: 2 in, 2 out]
              }
            }
            n1008 = local read "Save Next shot to File?"() -> (w1193:bool)
            n1009 = case shown="True" w1193 {
              tunnel: w1189 -> [_ w1197]
              tunnel: w1191 -> [_ w1198]
              frame False {
              }
              frame True {
                n1010 = call "string_to_formated_string.vi"("Numeric"=w1198) -> ("String"=w1200:string)  [unwired: 1 in]
                n1011 = call "string_to_formated_string.vi"("Numeric"=w1197) -> ("String"=w1201:string)  [unwired: 1 in]
                n1012 = local read "Time"() -> (w1205:string)
                n1013 = Build Array(w1205, w1200, w1201) -> (w1199:string[])
                n1014 = local read "Path SLAB #8"() -> (w1204:path)
                n1015 = call-poly <vilib>:"Write Delimited Spreadsheet.vi"("file path (dialog if empty)"=w1204, "1D data"=w1199, "append to file? (new file:F)"=TRUE, "delimiter (\\t)"="," ("delimiter (\\t)")) -> ()  [unwired: 10 in, 2 out]
              }
            }
          }
          frame True {
          }
        }
        n1016 = case shown="False" w1186 {
          tunnel: w1185 -> [w1213 _]
          frame False {
            n1017 = local write "Measure 9"(w1213) -> ()
            n1018 = local read "Threshold Green 1"() -> (w1218:dbl)
            n1019 = Multiply(x=w1213, y="Factor 9") -> (x*y=w1212:T3)
            n1020 = shared-variable "My Computer\\Server Library.lvlib\\slab10"(w1212) -> ()  [unwired: 1 in, 1 out]
            n1021 = Multiply(x=w1213, y=1.0) -> (x*y=w1214:dbl)
            n1022 = local write "Ch 9"(w1212) -> ()
            n1023 = Greater Or Equal?(x=w1212, y=w1218) -> (x >= y?=w1217:bool)
            n1024 = case shown="False" w1217 {
              tunnel: w1212 -> [w1231 _]
              frame False {
                n1025 = local read "Threshold Green 2"() -> (w1230:dbl)
                n1026 = Less?(x=w1231, y=w1230) -> (x < y?=w1229:bool)
                n1027 = case shown="True" w1229 {
                  frame False {
                    w1232 = cluster{u32, u32}[] [{1985280, 0}, {16769536, 0}] ("Colors [4]")
                    n1028 = property on="Ch 09 Status 2" class="Bool (strict)"("Colors [4]"=w1232) -> ()  [unwired: 2 in, 2 out]
                    n1029 = property on="Ch 09 Status" class="Bool (strict)"("Colors [4]"=w1232) -> ()  [unwired: 2 in, 2 out]
                  }
                  frame True {
                    w1233 = cluster{u32, u32}[] [{1985280, 0}, {16722474, 0}] ("Colors [4]")
                    n1030 = property on="Ch 09 Status" class="Bool (strict)"("Colors [4]"=w1233) -> ()  [unwired: 2 in, 2 out]
                    n1031 = property on="Ch 09 Status 2" class="Bool (strict)"("Colors [4]"=w1233) -> ()  [unwired: 2 in, 2 out]
                  }
                }
              }
              frame True {
                w1234 = cluster{u32, u32}[] [{1985280, 0}, {6618880, 0}] ("Colors [4]")
                n1032 = property on="Ch 09 Status" class="Bool (strict)"("Colors [4]"=w1234) -> ()  [unwired: 2 in, 2 out]
                n1033 = property on="Ch 09 Status 2" class="Bool (strict)"("Colors [4]"=w1234) -> ()  [unwired: 2 in, 2 out]
              }
            }
            n1034 = local read "Save Next shot to File?"() -> (w1216:bool)
            n1035 = case shown="True" w1216 {
              tunnel: w1212 -> [_ w1220]
              tunnel: w1214 -> [_ w1221]
              frame False {
              }
              frame True {
                n1036 = call "string_to_formated_string.vi"("Numeric"=w1220) -> ("String"=w1224:string)  [unwired: 1 in]
                n1037 = call "string_to_formated_string.vi"("Numeric"=w1221) -> ("String"=w1222:string)  [unwired: 1 in]
                n1038 = local read "Time"() -> (w1228:string)
                n1039 = local read "Path SLAB #10"() -> (w1225:path)
                n1040 = Build Array(w1228, w1222, w1224) -> (w1223:string[])
                n1041 = call-poly <vilib>:"Write Delimited Spreadsheet.vi"("file path (dialog if empty)"=w1225, "1D data"=w1223, "append to file? (new file:F)"=TRUE, "delimiter (\\t)"="," ("delimiter (\\t)")) -> ()  [unwired: 10 in, 2 out]
              }
            }
          }
          frame True {
          }
        }
      }
      frame #5 {
        # "Display mJ in bar plot and Measure Indicator for 2nd stage , but still in J in the file"
        n1042 = local read "Ch 12 Status"() -> (w1235:bool)
        n1043 = local read "Ch 11 Status"() -> (w1236:bool)
        n1044 = call "Read.vi"("Ch2 Status"=w1235, "Com Port"=w1241, "Ch1 Status"=w1236) -> ("Ch 2 out"=w1237:dbl, "Ch 1 out"=w1238:dbl)
        n1045 = Equal To 0?(x=w1237) -> (x = 0?=w1240:bool)
        n1046 = Equal To 0?(x=w1238) -> (x = 0?=w1239:bool)
        n1047 = case shown="False" w1240 {
          tunnel: w1237 -> [w1243 _]
          frame False {
            n1048 = local write "Measure 12"(w1243) -> ()
            n1049 = Multiply(x=w1243, y="Factor 12") -> (x*y=w1242:T3)
            n1050 = local read "Threshold 3rd stage 1"() -> (w1248:dbl)
            n1051 = Multiply(x=w1243, y=1.0) -> (x*y=w1244:dbl)
            n1052 = local write "Ch 12"(w1242) -> ()
            n1053 = Greater Or Equal?(x=w1242, y=w1248) -> (x >= y?=w1247:bool)
            n1054 = shared-variable "My Computer\\Server Library.lvlib\\stage3"(w1242) -> ()  [unwired: 1 in, 1 out]
            n1055 = case shown="False" w1247 {
              tunnel: w1242 -> [w1261 _]
              frame False {
                n1056 = local read "Threshold 3rd stage 2"() -> (w1260:dbl)
                n1057 = Less?(x=w1261, y=w1260) -> (x < y?=w1259:bool)
                n1058 = case shown="True" w1259 {
                  frame False {
                    w1262 = cluster{u32, u32}[] [{1985280, 0}, {16769536, 0}] ("Colors [4]")
                    n1059 = property on="Ch 12 Status 2" class="Bool (strict)"("Colors [4]"=w1262) -> ()  [unwired: 2 in, 2 out]
                    n1060 = property on="Ch 12 Status" class="Bool (strict)"("Colors [4]"=w1262) -> ()  [unwired: 2 in, 2 out]
                  }
                  frame True {
                    w1263 = cluster{u32, u32}[] [{1985280, 0}, {16722474, 0}] ("Colors [4]")
                    n1061 = property on="Ch 12 Status 2" class="Bool (strict)"("Colors [4]"=w1263) -> ()  [unwired: 2 in, 2 out]
                    n1062 = property on="Ch 12 Status" class="Bool (strict)"("Colors [4]"=w1263) -> ()  [unwired: 2 in, 2 out]
                  }
                }
              }
              frame True {
                w1264 = cluster{u32, u32}[] [{1985280, 0}, {6618880, 0}] ("Colors [4]")
                n1063 = property on="Ch 12 Status" class="Bool (strict)"("Colors [4]"=w1264) -> ()  [unwired: 2 in, 2 out]
                n1064 = property on="Ch 12 Status 2" class="Bool (strict)"("Colors [4]"=w1264) -> ()  [unwired: 2 in, 2 out]
              }
            }
            n1065 = local read "Save Next shot to File?"() -> (w1246:bool)
            n1066 = case shown="True" w1246 {
              tunnel: w1242 -> [_ w1251]
              tunnel: w1244 -> [_ w1250]
              frame False {
              }
              frame True {
                n1067 = call "string_to_formated_string.vi"("Numeric"=w1251) -> ("String"=w1254:string)  [unwired: 1 in]
                n1068 = call "string_to_formated_string.vi"("Numeric"=w1250) -> ("String"=w1253:string)  [unwired: 1 in]
                n1069 = local read "Time"() -> (w1257:string)
                n1070 = Build Array(w1257, w1253, w1254) -> (w1252:string[])
                n1071 = local read "Path 3rd stage"() -> (w1258:path)
                n1072 = call-poly <vilib>:"Write Delimited Spreadsheet.vi"("file path (dialog if empty)"=w1258, "1D data"=w1252, "append to file? (new file:F)"=TRUE, "delimiter (\\t)"="," ("delimiter (\\t)")) -> ()  [unwired: 10 in, 2 out]
              }
            }
          }
          frame True {
          }
        }
        n1073 = case shown="False" w1239 {
          tunnel: w1238 -> [w1267 _]
          frame False {
            n1074 = local write "Measure 11"(w1267) -> ()
            n1075 = Multiply(x=w1267, y="Factor 11") -> (x*y=w1265:T3)
            n1076 = local read "Threshold 2nd stage 1"() -> (w1273:dbl)
            n1077 = Multiply(x=w1267, y=1.0) -> (x*y=w1268:dbl)
            n1078 = Multiply(x=w1265, y=1000.0) -> (x*y=w1266:T3)
            n1079 = local write "Ch 11"(w1266) -> ()
            n1080 = Greater Or Equal?(x=w1265, y=w1273) -> (x >= y?=w1272:bool)
            n1081 = shared-variable "My Computer\\Server Library.lvlib\\stage2"(w1265) -> ()  [unwired: 1 in, 1 out]
            n1082 = case shown="False" w1272 {
              tunnel: w1265 -> [w1286 _]
              frame False {
                n1083 = local read "Threshold 2nd stage 2"() -> (w1285:dbl)
                n1084 = Less?(x=w1286, y=w1285) -> (x < y?=w1284:bool)
                n1085 = case shown="True" w1284 {
                  frame False {
                    w1287 = cluster{u32, u32}[] [{1985280, 0}, {16769536, 0}] ("Colors [4]")
                    n1086 = property on="Ch 11 Status 2" class="Bool (strict)"("Colors [4]"=w1287) -> ()  [unwired: 2 in, 2 out]
                    n1087 = property on="Ch 11 Status" class="Bool (strict)"("Colors [4]"=w1287) -> ()  [unwired: 2 in, 2 out]
                  }
                  frame True {
                    w1288 = cluster{u32, u32}[] [{1985280, 0}, {16722474, 0}] ("Colors [4]")
                    n1088 = property on="Ch 11 Status" class="Bool (strict)"("Colors [4]"=w1288) -> ()  [unwired: 2 in, 2 out]
                    n1089 = property on="Ch 11 Status 2" class="Bool (strict)"("Colors [4]"=w1288) -> ()  [unwired: 2 in, 2 out]
                  }
                }
              }
              frame True {
                w1289 = cluster{u32, u32}[] [{1985280, 0}, {6618880, 0}] ("Colors [4]")
                n1090 = property on="Ch 11 Status 2" class="Bool (strict)"("Colors [4]"=w1289) -> ()  [unwired: 2 in, 2 out]
                n1091 = property on="Ch 11 Status" class="Bool (strict)"("Colors [4]"=w1289) -> ()  [unwired: 2 in, 2 out]
              }
            }
            n1092 = local read "Save Next shot to File?"() -> (w1271:bool)
            n1093 = case shown="True" w1271 {
              tunnel: w1265 -> [_ w1275]
              tunnel: w1268 -> [_ w1276]
              frame False {
              }
              frame True {
                n1094 = call "string_to_formated_string.vi"("Numeric"=w1275) -> ("String"=w1279:string)  [unwired: 1 in]
                n1095 = call "string_to_formated_string.vi"("Numeric"=w1276) -> ("String"=w1277:string)  [unwired: 1 in]
                n1096 = local read "Time"() -> (w1283:string)
                n1097 = Build Array(w1283, w1277, w1279) -> (w1278:string[])
                n1098 = local read "Path 2nd stage"() -> (w1282:path)
                n1099 = call-poly <vilib>:"Write Delimited Spreadsheet.vi"("file path (dialog if empty)"=w1282, "1D data"=w1278, "append to file? (new file:F)"=TRUE, "delimiter (\\t)"="," ("delimiter (\\t)")) -> ()  [unwired: 10 in, 2 out]
              }
            }
          }
          frame True {
          }
        }
      }
      frame #6 {
        # "Display mJ in bar plot and Measure Indicator for QuantaRay and 1st stage , but still in J in the file"
        n1100 = local read "Ch 13 Status"() -> (w1290:bool)
        n1101 = local read "Ch 14 Status"() -> (w1291:bool)
        n1102 = call "Read.vi"("Ch2 Status"=w1291, "Com Port"=w1296, "Ch1 Status"=w1290) -> ("Ch 2 out"=w1293:dbl, "Ch 1 out"=w1292:dbl)
        n1103 = Equal To 0?(x=w1293) -> (x = 0?=w1295:bool)
        n1104 = Equal To 0?(x=w1292) -> (x = 0?=w1294:bool)
        n1105 = case shown="False" w1295 {
          tunnel: w1293 -> [w1298 _]
          frame False {
            n1106 = local write "Measure 14"(w1298) -> ()
            n1107 = local read "Threshold 1st stage 1"() -> (w1305:dbl)
            n1108 = Multiply(x=w1298, y="Factor 14") -> (x*y=w1297:T3)
            n1109 = Multiply(x=w1297, y=1000.0) -> (x*y=w1301:T3)
            n1110 = Multiply(x=w1298, y=1.0) -> (x*y=w1299:dbl)
            n1111 = local write "Ch 14"(w1301) -> ()
            n1112 = Greater Or Equal?(x=w1297, y=w1305) -> (x >= y?=w1304:bool)
            n1113 = shared-variable "My Computer\\Server Library.lvlib\\stage1"(w1297) -> ()  [unwired: 1 in, 1 out]
            n1114 = case shown="True" w1304 {
              tunnel: w1297 -> [w1318 _]
              frame False {
                n1115 = local read "Threshold 1st stage 2"() -> (w1317:dbl)
                n1116 = Less?(x=w1318, y=w1317) -> (x < y?=w1316:bool)
                n1117 = case shown="False" w1316 {
                  frame False {
                    w1319 = cluster{u32, u32}[] [{1985280, 0}, {16769536, 0}] ("Colors [4]")
                    n1118 = property on="Ch 14 Status 2" class="Bool (strict)"("Colors [4]"=w1319) -> ()  [unwired: 2 in, 2 out]
                    n1119 = property on="Ch 14 Status" class="Bool (strict)"("Colors [4]"=w1319) -> ()  [unwired: 2 in, 2 out]
                  }
                  frame True {
                    w1320 = cluster{u32, u32}[] [{1985280, 0}, {16722474, 0}] ("Colors [4]")
                    n1120 = property on="Ch 14 Status 2" class="Bool (strict)"("Colors [4]"=w1320) -> ()  [unwired: 2 in, 2 out]
                    n1121 = property on="Ch 14 Status" class="Bool (strict)"("Colors [4]"=w1320) -> ()  [unwired: 2 in, 2 out]
                  }
                }
              }
              frame True {
                w1321 = cluster{u32, u32}[] [{1985280, 0}, {6618880, 0}] ("Colors [4]")
                n1122 = property on="Ch 14 Status 2" class="Bool (strict)"("Colors [4]"=w1321) -> ()  [unwired: 2 in, 2 out]
                n1123 = property on="Ch 14 Status" class="Bool (strict)"("Colors [4]"=w1321) -> ()  [unwired: 2 in, 2 out]
              }
            }
            n1124 = local read "Save Next shot to File?"() -> (w1303:bool)
            n1125 = case shown="True" w1303 {
              tunnel: w1297 -> [_ w1308]
              tunnel: w1299 -> [_ w1307]
              frame False {
              }
              frame True {
                n1126 = local read "Time"() -> (w1314:string)
                n1127 = call "string_to_formated_string.vi"("Numeric"=w1308) -> ("String"=w1311:string)  [unwired: 1 in]
                n1128 = call "string_to_formated_string.vi"("Numeric"=w1307) -> ("String"=w1310:string)  [unwired: 1 in]
                n1129 = local read "Path 1st stage"() -> (w1315:path)
                n1130 = Build Array(w1314, w1310, w1311) -> (w1309:string[])
                n1131 = call-poly <vilib>:"Write Delimited Spreadsheet.vi"("file path (dialog if empty)"=w1315, "1D data"=w1309, "append to file? (new file:F)"=TRUE, "delimiter (\\t)"="," ("delimiter (\\t)")) -> ()  [unwired: 10 in, 2 out]
              }
            }
          }
          frame True {
          }
        }
        n1132 = case shown="False" w1294 {
          tunnel: w1292 -> [w1323 _]
          frame False {
            n1133 = local read "Threshold quantaray stage 1"() -> (w1330:dbl)
            n1134 = local write "Measure 13"(w1323) -> ()
            n1135 = Multiply(x=w1323, y="Factor 13") -> (x*y=w1322:T3)
            n1136 = Multiply(x=w1322, y=1000.0) -> (x*y=w1324:T3)
            n1137 = local write "Ch 13"(w1324) -> ()
            n1138 = Greater Or Equal?(x=w1322, y=w1330) -> (x >= y?=w1329:bool)
            n1139 = case shown="False" w1329 {
              tunnel: w1322 -> [w1343 _]
              frame False {
                n1140 = local read "Threshold quantaray stage 2"() -> (w1342:dbl)
                n1141 = Less?(x=w1343, y=w1342) -> (x < y?=w1341:bool)
                n1142 = case shown="True" w1341 {
                  frame False {
                    w1344 = cluster{u32, u32}[] [{1985280, 0}, {16769536, 0}] ("Colors [4]")
                    n1143 = property on="Ch 13 Status 2" class="Bool (strict)"("Colors [4]"=w1344) -> ()  [unwired: 2 in, 2 out]
                    n1144 = property on="Ch 13 Status" class="Bool (strict)"("Colors [4]"=w1344) -> ()  [unwired: 2 in, 2 out]
                  }
                  frame True {
                    w1345 = cluster{u32, u32}[] [{1985280, 0}, {16722474, 0}] ("Colors [4]")
                    n1145 = property on="Ch 13 Status 2" class="Bool (strict)"("Colors [4]"=w1345) -> ()  [unwired: 2 in, 2 out]
                    n1146 = property on="Ch 13 Status" class="Bool (strict)"("Colors [4]"=w1345) -> ()  [unwired: 2 in, 2 out]
                  }
                }
              }
              frame True {
                w1346 = cluster{u32, u32}[] [{1985280, 0}, {6618880, 0}] ("Colors [4]")
                n1147 = property on="Ch 13 Status" class="Bool (strict)"("Colors [4]"=w1346) -> ()  [unwired: 2 in, 2 out]
                n1148 = property on="Ch 13 Status 2" class="Bool (strict)"("Colors [4]"=w1346) -> ()  [unwired: 2 in, 2 out]
              }
            }
            n1149 = shared-variable "My Computer\\Server Library.lvlib\\QuantaRay"(w1322) -> ()  [unwired: 1 in, 1 out]
            n1150 = Multiply(x=w1323, y=1.0) -> (x*y=w1325:dbl)
            n1151 = local read "Save Next shot to File?"() -> (w1328:bool)
            n1152 = case shown="True" w1328 {
              tunnel: w1322 -> [_ w1332]
              tunnel: w1325 -> [_ w1333]
              frame False {
              }
              frame True {
                n1153 = call "string_to_formated_string.vi"("Numeric"=w1332) -> ("String"=w1336:string)  [unwired: 1 in]
                n1154 = call "string_to_formated_string.vi"("Numeric"=w1333) -> ("String"=w1334:string)  [unwired: 1 in]
                n1155 = local read "Time"() -> (w1340:string)
                n1156 = Build Array(w1340, w1334, w1336) -> (w1335:string[])
                n1157 = local read "Path quanta ray"() -> (w1339:path)
                n1158 = call-poly <vilib>:"Write Delimited Spreadsheet.vi"("file path (dialog if empty)"=w1339, "1D data"=w1335, "append to file? (new file:F)"=TRUE, "delimiter (\\t)"="," ("delimiter (\\t)")) -> ()  [unwired: 10 in, 2 out]
              }
            }
          }
          frame True {
          }
        }
      }
      frame #7 {
        n1159 = local read "Ch 16 Status"() -> (w1347:bool)
        n1160 = local read "Ch 15 Status"() -> (w1349:bool)
        n1161 = call "Read.vi"("Ch2 Status"=w1347, "Com Port"=w1353, "Ch1 Status"=w1349) -> ("Ch 2 out"=w1350:dbl, "Ch 1 out"=w1351:dbl)
        n1162 = Equal To 0?(x=w1350) -> (x = 0?=w1348:bool)
        n1163 = Equal To 0?(x=w1351) -> (x = 0?=w1352:bool)
        n1164 = case shown="False" w1348 {
          selector: w1348 -> [w1363 w1394]
          tunnel: w1350 -> [w1369 _]
          tunnel: w1347 -> [w1365 _]
          frame False {
            n1165 = local write "Measure 16"(w1369) -> ()
            n1166 = local read "Threshold 5th stage 1"() -> (w1377:dbl)
            n1167 = call "Polynomial_factor.vi"("Input"=w1369, "c"="Factor c", "b"="Factor b", "a"="Factor a") -> ("Output"=w1362:dbl)
            n1168 = local write "Ch 16"(w1362) -> ()
            n1169 = Multiply(x=w1369, y=1.0) -> (x*y=w1370:dbl)
            n1170 = Greater Or Equal?(x=w1362, y=w1377) -> (x >= y?=w1376:bool)
            n1171 = shared-variable "My Computer\\Server Library.lvlib\\stage5"(w1362) -> ()  [unwired: 1 in, 1 out]
            n1172 = case shown="True" w1376 {
              tunnel: w1362 -> [w1390 _]
              tunnel: [w1387 w1393] -> w1366
              frame False {
                n1173 = local read "Threshold 5th stage 2"() -> (w1389:dbl)
                n1174 = Less?(x=w1390, y=w1389) -> (x < y?=w1388:bool)
                n1175 = case shown="False" w1388 {
                  tunnel: [w1391 w1392] -> w1387
                  frame False {
                    w1391 = cluster{u32, u32}[] [{1985280, 0}, {16769536, 0}] ("Colors [4]")
                    n1176 = property on="Ch 16 Status 2" class="Bool (strict)"("Colors [4]"=w1391) -> ()  [unwired: 2 in, 2 out]
                    n1177 = property on="Ch 16 Status" class="Bool (strict)"("Colors [4]"=w1391) -> ()  [unwired: 2 in, 2 out]
                  }
                  frame True {
                    w1392 = cluster{u32, u32}[] [{1985280, 0}, {16722474, 0}] ("Colors [4]")
                    n1178 = property on="Ch 16 Status 2" class="Bool (strict)"("Colors [4]"=w1392) -> ()  [unwired: 2 in, 2 out]
                    n1179 = property on="Ch 16 Status" class="Bool (strict)"("Colors [4]"=w1392) -> ()  [unwired: 2 in, 2 out]
                  }
                }
              }
              frame True {
                w1393 = cluster{u32, u32}[] [{1985280, 0}, {6618880, 0}] ("Colors [4]")
                n1180 = property on="Ch 16 Status 2" class="Bool (strict)"("Colors [4]"=w1393) -> ()  [unwired: 2 in, 2 out]
                n1181 = property on="Ch 16 Status" class="Bool (strict)"("Colors [4]"=w1393) -> ()  [unwired: 2 in, 2 out]
              }
            }
            n1182 = local read "Save Next shot to File?"() -> (w1375:bool)
            n1183 = local read "Time"() -> (w1364:string)
            n1184 = case shown="True" w1375 {
              tunnel: w1362 -> [_ w1378]
              tunnel: w1370 -> [_ w1379]
              frame False {
              }
              frame True {
                n1185 = call "string_to_formated_string.vi"("Numeric"=w1378) -> ("String"=w1382:string)  [unwired: 1 in]
                n1186 = call "string_to_formated_string.vi"("Numeric"=w1379) -> ("String"=w1381:string)  [unwired: 1 in]
                n1187 = local read "Time"() -> (w1385:string)
                n1188 = Build Array(w1385, w1381, w1382) -> (w1380:string[])
                n1189 = local read "Path 5th stage"() -> (w1386:path)
                n1190 = call-poly <vilib>:"Write Delimited Spreadsheet.vi"("file path (dialog if empty)"=w1386, "1D data"=w1380, "append to file? (new file:F)"=TRUE, "delimiter (\\t)"="," ("delimiter (\\t)")) -> ()  [unwired: 10 in, 2 out]
              }
            }
            n1191 = local read "Second Window Output"() -> (w1368:T1)
            n1192 = Bundle By Name(cluster=w1368, "Energy Value"=w1362, "Indicator Color"=w1366, "Status"=w1365, "Time"=w1364, "Energy stat"=w1363) -> (w1367:T1)
            n1193 = local write "Second Window Output"(w1367) -> ()
            n1194 = Format Date/Time String(time format string (%c)="%y%m%d%H%M%S") -> (date/time string=w1354:string)  [unwired: 2 in]
            n1195 = Format Date/Time String(time format string (%c)="%2u") -> (date/time string=w1360:string)  [unwired: 2 in]
            n1196 = String Subset(string=w1360, offset (0)=1, length (rest)=2) -> (substring=w1357:string)
            n1197 = Concatenate Strings(w1354, w1357) -> (w1356:string)
            n1198 = shared-variable "My Computer\\Server Library.lvlib\\timeStamp"(w1356) -> ()  [unwired: 1 in, 1 out]
          }
          frame True {
            n1199 = local read "Second Window Output"() -> (w1396:T1)
            n1200 = Bundle By Name(cluster=w1396, "Energy stat"=w1394) -> (w1395:T1)
            n1201 = local write "Second Window Output"(w1395) -> ()
          }
        }
        n1202 = case shown="False" w1352 {
          tunnel: w1351 -> [w1398 _]
          frame False {
            n1203 = local write "Measure 15"(w1398) -> ()
            n1204 = local read "Threshold 4th stage 1"() -> (w1403:dbl)
            n1205 = Multiply(x=w1398, y="Factor 15") -> (x*y=w1397:T3)
            n1206 = shared-variable "My Computer\\Server Library.lvlib\\stage4"(w1397) -> ()  [unwired: 1 in, 1 out]
            n1207 = local write "Ch 15"(w1397) -> ()
            n1208 = Greater Or Equal?(x=w1397, y=w1403) -> (x >= y?=w1402:bool)
            n1209 = case shown="False" w1402 {
              tunnel: w1397 -> [w1416 _]
              frame False {
                n1210 = local read "Threshold 4th stage 2"() -> (w1415:dbl)
                n1211 = Less?(x=w1416, y=w1415) -> (x < y?=w1414:bool)
                n1212 = case shown="False" w1414 {
                  frame False {
                    w1417 = cluster{u32, u32}[] [{1985280, 0}, {16769536, 0}] ("Colors [4]")
                    n1213 = property on="Ch 15 Status 2" class="Bool (strict)"("Colors [4]"=w1417) -> ()  [unwired: 2 in, 2 out]
                    n1214 = property on="Ch 15 Status" class="Bool (strict)"("Colors [4]"=w1417) -> ()  [unwired: 2 in, 2 out]
                  }
                  frame True {
                    w1418 = cluster{u32, u32}[] [{1985280, 0}, {16722474, 0}] ("Colors [4]")
                    n1215 = property on="Ch 15 Status 2" class="Bool (strict)"("Colors [4]"=w1418) -> ()  [unwired: 2 in, 2 out]
                    n1216 = property on="Ch 15 Status" class="Bool (strict)"("Colors [4]"=w1418) -> ()  [unwired: 2 in, 2 out]
                  }
                }
              }
              frame True {
                w1419 = cluster{u32, u32}[] [{1985280, 0}, {6618880, 0}] ("Colors [4]")
                n1217 = property on="Ch 15 Status" class="Bool (strict)"("Colors [4]"=w1419) -> ()  [unwired: 2 in, 2 out]
                n1218 = property on="Ch 15 Status 2" class="Bool (strict)"("Colors [4]"=w1419) -> ()  [unwired: 2 in, 2 out]
              }
            }
            n1219 = Multiply(x=w1398, y=1.0) -> (x*y=w1399:dbl)
            n1220 = local read "Save Next shot to File?"() -> (w1401:bool)
            n1221 = case shown="True" w1401 {
              tunnel: w1397 -> [_ w1406]
              tunnel: w1399 -> [_ w1405]
              frame False {
              }
              frame True {
                n1222 = call "string_to_formated_string.vi"("Numeric"=w1405) -> ("String"=w1407:string)  [unwired: 1 in]
                n1223 = call "string_to_formated_string.vi"("Numeric"=w1406) -> ("String"=w1409:string)  [unwired: 1 in]
                n1224 = local read "Time"() -> (w1413:string)
                n1225 = Build Array(w1413, w1407, w1409) -> (w1408:string[])
                n1226 = local read "Path 4th stage"() -> (w1412:path)
                n1227 = call-poly <vilib>:"Write Delimited Spreadsheet.vi"("file path (dialog if empty)"=w1412, "1D data"=w1408, "append to file? (new file:F)"=TRUE, "delimiter (\\t)"="," ("delimiter (\\t)")) -> ()  [unwired: 10 in, 2 out]
              }
            }
          }
          frame True {
          }
        }
      }
      frame #8 {
        # "Check for new Spectrum Data, and display if new data are found"
        n1228 = local read "Path Spectrometer Folder"() -> (w1423:path)
        n1229 = List Folder(path=w1423, pattern="*.csv") -> (filenames=w1424:string[])  [unwired: 2 in, 3 out]
        n1230 = Array Size(array=w1424) -> (size(s)=w1425:i32)
        n1231 = Not Equal?(x=w1425, y=0) -> (x != y?=w1426:bool)
        n1232 = case shown="True" w1426 {
          tunnel: w1424 -> [_ w1436]
          tunnel: w1423 -> [_ w1435]
          tunnel: [FALSE w1434] -> w1421
          tunnel: [w1428 w1431] -> w1420
          frame False {
            n1233 = String To Path(string="") -> (path=w1428:path)
          }
          frame True {
            n1234 = Reverse 1D Array(array=w1436) -> (reversed array=w1437:string[])
            n1235 = Index Array(array=w1437) -> (element=w1438:string)  [unwired: 1 in]
            n1236 = String To Path(string=w1438) -> (path=w1432:path)
            n1237 = local read "Path Spectrometer Data Old"() -> (w1433:path)
            n1238 = Build Path(base path=w1435, name or relative path=w1432) -> (appended path=w1431:path)
            n1239 = Not Equal?(x=w1431, y=w1433) -> (x != y?=w1434:bool)
          }
        }
        n1240 = case shown="True" w1421 {
          tunnel: w1420 -> [_ w1439]
          frame False {
          }
          frame True {
            # "Read Spectrum data from .csv. Seperate the data into wavelength and intensity, and reduce the output range to 750-850nm"
            n1241 = flat-sequence {
              tunnel: w1439 -> [w1449]
              frame #0 {
                n1242 = Wait (ms)(milliseconds to wait=80) -> ()  [unwired: 1 out]
              }
              frame #1 {
                w1444 = 500
                w1445 = 275
                w1452 = 0
                w1451 = 1
                n1243 = local write "Path Spectrometer Data Old"(w1449) -> ()
                n1244 = call-poly <vilib>:"Read Delimited Spreadsheet.vi"("file path (dialog if empty)"=w1449, "delimiter (\\t)"=",") -> ("all rows"=w1453:dbl[][])  [unwired: 8 in, 5 out]
                n1245 = Array Subset(array=w1453, index (row)=w1445, length (row)=w1444, index (col)=w1452, length (col)=w1451) -> (w1454:dbl[][])
                n1246 = Array Subset(array=w1453, index (row)=w1445, length (row)=w1444, index (col)=w1451, length (col)=w1451) -> (w1455:dbl[][])
                n1247 = Index Array(array=w1455, index (col)=w1452) -> (element=w1442:dbl[])  [unwired: 1 in]
                n1248 = local read "Second Window Output"() -> (w1448:T1)
                n1249 = Index Array(array=w1454, index (col)=w1452) -> (element=w1456:dbl[])  [unwired: 1 in]
                n1250 = Array Max & Min(array=w1442) -> (max value=w1443:dbl)  [unwired: 3 out]
                n1251 = Divide(x=w1442, y=w1443) -> (x/y=w1441:dbl[])
                n1252 = Bundle(w1456, w1441) -> (w1447:cluster{dbl[], dbl[]})  [unwired: 1 in]
                n1253 = Bundle By Name(cluster=w1448, "Spectrometer Output"=w1447) -> (w1446:T1)
                n1254 = local write "Second Window Output"(w1446) -> ()
              }
            }
          }
        }
      }
      frame #9 {
        n1255 = local read "Second Window Output"() -> (w1464:T1)
        n1256 = Format Date/Time String(time format string (%c)="%Y%m%d%H%M") -> (date/time string=w1457:string)  [unwired: 2 in]
        n1257 = Unbundle By Name(w1464) -> ("Energy Value"=w1463:dbl, "Energy stat"=w1462:bool, "Indicator Color"=w1461:cluster{u32, u32}[], "Status"=w1460:bool, "Spectrometer Output"=w1459:cluster{dbl[], dbl[]})
        n1258 = call "16Chennels_ExtraWindow.vi"("Spectral Waveform"=w1459, "Energy Data"=w1463, "New Energy"=w1462, "Shot # in"=w1457, "Ch 16 Status"=w1460, "Colors [4]"=w1461) -> ()  [unwired: 4 in]
      }
    }
    n1259 = local read "Com Port 2"() -> (w954:refnum<visa-resource-name>)
    n1260 = local read "Com Port 4"() -> (w934:refnum<visa-resource-name>)
    n1261 = local read "Com Port 6"() -> (w909:refnum<visa-resource-name>)
    n1262 = local read "Com Port 8"() -> (w889:refnum<visa-resource-name>)
    n1263 = local read "Com Port 2"() -> (w959:refnum<visa-resource-name>)
    n1264 = local read "Com Port 6"() -> (w904:refnum<visa-resource-name>)
    n1265 = local read "Com Port 8"() -> (w884:refnum<visa-resource-name>)
    n1266 = local read "Com Port 4"() -> (w939:refnum<visa-resource-name>)
    n1267 = local read "Stop Application"() -> (w917:bool)
    n1268 = case shown="False" "Scale UP 4" {
      tunnel: w954 -> [_ w2143]
      frame False {
      }
      frame True {
        n1269 = stacked-sequence {
          tunnel: w2143 -> [w2145 w2150 w2152]
          tunnel: [w2145 _ _] -> w2141
          frame #0 {
            w2147 = 10 items=["*RST", "*PWC", "*CA1", "*CA2", "*SS1001", "*SS2001", "*SU1", "*SU2", "*SD1", "*SD2", "*CS1", "*CS2"] ("string to write")
            n1270 = call "Send.vi"("string to write"=w2147, "port number"=w2145) -> ()  [unwired: 1 in]
            n1271 = Wait (ms)(milliseconds to wait=10) -> ()  [unwired: 1 out]
          }
          frame #1 {
            w2148 = 11 items=["*RST", "*VER", "*CA1", "*CA2", "*SS100", "*SS200", "*SU1", "*SU2", "*SD1", "*SD2", "*CS1", "*CS2", "*AT1", "*AT2", "*AN1", "*AN2", "*PW1", "*PW2", "*TL1", "*TL2", "*ST1", "*ST2", "*ET1", "*ET2", "*EM1", "*EM2", "*SC1", "*SC2"] ("string to write")
            n1272 = call "Send.vi"("string to write"=w2148, "port number"=w2150) -> ()  [unwired: 1 in]
            n1273 = Wait (ms)(milliseconds to wait=10) -> ()  [unwired: 1 out]
          }
          frame #2 {
            w2153 = 7 items=["*RST", "*PWC", "*CA1", "*CA2", "*SS1001", "*SS2001", "*SU1", "*SU2", "*SD1", "*SD2"] ("string to write")
            n1274 = call "Send.vi"("string to write"=w2153, "port number"=w2152) -> ()  [unwired: 1 in]
            n1275 = Wait (ms)(milliseconds to wait=10) -> ()  [unwired: 1 out]
          }
        }
        n1276 = local write "Scale UP 4"(FALSE) -> ()
        n1277 = local read "Ch 04 Status"() -> (w2139:bool)
        n1278 = local read "Ch 03 Status"() -> (w2140:bool)
        n1279 = call "Read Scale Ch 2.vi"("Ch 2"=w2139, "Com Port"=w2141, "Ch1"=w2140) -> ("Scale Ch2"=w2142:dbl)  [unwired: 2 out]
        n1280 = local write "Scale 4"(w2142) -> ()
      }
    }
    n1281 = case shown="False" "Scale UP 3" {
      tunnel: w959 -> [_ w2188]
      frame False {
      }
      frame True {
        n1282 = stacked-sequence {
          tunnel: w2188 -> [w2190 w2193 w2197]
          tunnel: [w2190 _ _] -> w2187
          frame #0 {
            w2192 = 10 items=["*RST", "*PWC", "*CA1", "*CA2", "*SS1001", "*SS2001", "*SU1", "*SU2", "*SD1", "*SD2", "*CS1", "*CS2"] ("string to write")
            n1283 = call "Send.vi"("string to write"=w2192, "port number"=w2190) -> ()  [unwired: 1 in]
            n1284 = Wait (ms)(milliseconds to wait=10) -> ()  [unwired: 1 out]
          }
          frame #1 {
            w2195 = 11 items=["*RST", "*PWC", "*CA1", "*CA2", "*SS1001", "*SS2001", "*SU1", "*SU2", "*SD1", "*SD2", "*CS1", "*CS2"] ("string to write")
            n1285 = call "Send.vi"("string to write"=w2195, "port number"=w2193) -> ()  [unwired: 1 in]
            n1286 = Wait (ms)(milliseconds to wait=10) -> ()  [unwired: 1 out]
          }
          frame #2 {
            w2198 = 6 items=["*RST", "*PWC", "*CA1", "*CA2", "*SS1001", "*SS2001", "*SU1", "*SU2", "*SD1", "*SD2"] ("string to write")
            n1287 = call "Send.vi"("string to write"=w2198, "port number"=w2197) -> ()  [unwired: 1 in]
            n1288 = Wait (ms)(milliseconds to wait=10) -> ()  [unwired: 1 out]
          }
        }
        n1289 = local write "Scale UP 3"(FALSE) -> ()
        n1290 = local read "Ch 04 Status"() -> (w2185:bool)
        n1291 = local read "Ch 03 Status"() -> (w2186:bool)
        n1292 = call "Read Scale Ch 1.vi"("Ch2"=w2185, "Com Port"=w2187, "Ch 1"=w2186) -> ("Scale 1Ch"=w2184:dbl)  [unwired: 2 out]
        n1293 = local write "Scale 3"(w2184) -> ()
      }
    }
    n1294 = case shown="False" "Scale UP 12" {
      tunnel: w909 -> [_ w1643]
      frame False {
      }
      frame True {
        n1295 = stacked-sequence {
          tunnel: w1643 -> [w1645 w1650 w1652]
          tunnel: [w1645 _ _] -> w1641
          frame #0 {
            w1647 = 10 items=["*RST", "*PWC", "*CA1", "*CA2", "*SS1001", "*SS2001", "*SU1", "*SU2", "*SD1", "*SD2", "*CS1", "*CS2"] ("string to write")
            n1296 = call "Send.vi"("string to write"=w1647, "port number"=w1645) -> ()  [unwired: 1 in]
            n1297 = Wait (ms)(milliseconds to wait=10) -> ()  [unwired: 1 out]
          }
          frame #1 {
            w1648 = 11 items=["*RST", "*VER", "*CA1", "*CA2", "*SS100", "*SS200", "*SU1", "*SU2", "*SD1", "*SD2", "*CS1", "*CS2", "*AT1", "*AT2", "*AN1", "*AN2", "*PW1", "*PW2", "*TL1", "*TL2", "*ST1", "*ST2", "*ET1", "*ET2", "*EM1", "*EM2", "*SC1", "*SC2"] ("string to write")
            n1298 = call "Send.vi"("string to write"=w1648, "port number"=w1650) -> ()  [unwired: 1 in]
            n1299 = Wait (ms)(milliseconds to wait=10) -> ()  [unwired: 1 out]
          }
          frame #2 {
            w1653 = 7 items=["*RST", "*PWC", "*CA1", "*CA2", "*SS1001", "*SS2001", "*SU1", "*SU2", "*SD1", "*SD2"] ("string to write")
            n1300 = call "Send.vi"("string to write"=w1653, "port number"=w1652) -> ()  [unwired: 1 in]
            n1301 = Wait (ms)(milliseconds to wait=10) -> ()  [unwired: 1 out]
          }
        }
        n1302 = local write "Scale UP 12"(FALSE) -> ()
        n1303 = local read "Ch 12 Status"() -> (w1639:bool)
        n1304 = local read "Ch 11 Status"() -> (w1640:bool)
        n1305 = call "Read Scale Ch 2.vi"("Ch 2"=w1639, "Com Port"=w1641, "Ch1"=w1640) -> ("Scale Ch2"=w1642:dbl)  [unwired: 2 out]
        n1306 = local write "Scale 12"(w1642) -> ()
      }
    }
    n1307 = case shown="False" "Scale UP 16" {
      tunnel: w889 -> [_ w1487]
      frame False {
      }
      frame True {
        n1308 = stacked-sequence {
          tunnel: w1487 -> [w1489 w1494 w1496]
          tunnel: [w1489 _ _] -> w1485
          frame #0 {
            w1491 = 10 items=["*RST", "*PWC", "*CA1", "*CA2", "*SS1001", "*SS2001", "*SU1", "*SU2", "*SD1", "*SD2", "*CS1", "*CS2"] ("string to write")
            n1309 = call "Send.vi"("string to write"=w1491, "port number"=w1489) -> ()  [unwired: 1 in]
            n1310 = Wait (ms)(milliseconds to wait=10) -> ()  [unwired: 1 out]
          }
          frame #1 {
            w1492 = 11 items=["*RST", "*VER", "*CA1", "*CA2", "*SS100", "*SS200", "*SU1", "*SU2", "*SD1", "*SD2", "*CS1", "*CS2", "*AT1", "*AT2", "*AN1", "*AN2", "*PW1", "*PW2", "*TL1", "*TL2", "*ST1", "*ST2", "*ET1", "*ET2", "*EM1", "*EM2", "*SC1", "*SC2"] ("string to write")
            n1311 = call "Send.vi"("string to write"=w1492, "port number"=w1494) -> ()  [unwired: 1 in]
            n1312 = Wait (ms)(milliseconds to wait=10) -> ()  [unwired: 1 out]
          }
          frame #2 {
            w1497 = 7 items=["*RST", "*PWC", "*CA1", "*CA2", "*SS1001", "*SS2001", "*SU1", "*SU2", "*SD1", "*SD2"] ("string to write")
            n1313 = call "Send.vi"("string to write"=w1497, "port number"=w1496) -> ()  [unwired: 1 in]
            n1314 = Wait (ms)(milliseconds to wait=10) -> ()  [unwired: 1 out]
          }
        }
        n1315 = local write "Scale UP 16"(FALSE) -> ()
        n1316 = local read "Ch 16 Status"() -> (w1483:bool)
        n1317 = local read "Ch 15 Status"() -> (w1484:bool)
        n1318 = call "Read Scale Ch 2.vi"("Ch 2"=w1483, "Com Port"=w1485, "Ch1"=w1484) -> ("Scale Ch2"=w1486:dbl)  [unwired: 2 out]
        n1319 = local write "Scale 16"(w1486) -> ()
      }
    }
    n1320 = case shown="False" "Scale UP 8" {
      tunnel: w934 -> [_ w1987]
      frame False {
      }
      frame True {
        n1321 = stacked-sequence {
          tunnel: w1987 -> [w1989 w1994 w1996]
          tunnel: [w1989 _ _] -> w1985
          frame #0 {
            w1991 = 10 items=["*RST", "*PWC", "*CA1", "*CA2", "*SS1001", "*SS2001", "*SU1", "*SU2", "*SD1", "*SD2", "*CS1", "*CS2"] ("string to write")
            n1322 = call "Send.vi"("string to write"=w1991, "port number"=w1989) -> ()  [unwired: 1 in]
            n1323 = Wait (ms)(milliseconds to wait=10) -> ()  [unwired: 1 out]
          }
          frame #1 {
            w1992 = 11 items=["*RST", "*VER", "*CA1", "*CA2", "*SS100", "*SS200", "*SU1", "*SU2", "*SD1", "*SD2", "*CS1", "*CS2", "*AT1", "*AT2", "*AN1", "*AN2", "*PW1", "*PW2", "*TL1", "*TL2", "*ST1", "*ST2", "*ET1", "*ET2", "*EM1", "*EM2", "*SC1", "*SC2"] ("string to write")
            n1324 = call "Send.vi"("string to write"=w1992, "port number"=w1994) -> ()  [unwired: 1 in]
            n1325 = Wait (ms)(milliseconds to wait=10) -> ()  [unwired: 1 out]
          }
          frame #2 {
            w1997 = 7 items=["*RST", "*PWC", "*CA1", "*CA2", "*SS1001", "*SS2001", "*SU1", "*SU2", "*SD1", "*SD2"] ("string to write")
            n1326 = call "Send.vi"("string to write"=w1997, "port number"=w1996) -> ()  [unwired: 1 in]
            n1327 = Wait (ms)(milliseconds to wait=10) -> ()  [unwired: 1 out]
          }
        }
        n1328 = local write "Scale UP 8"(FALSE) -> ()
        n1329 = local read "Ch 08 Status"() -> (w1983:bool)
        n1330 = local read "Ch 07 Status"() -> (w1984:bool)
        n1331 = call "Read Scale Ch 2.vi"("Ch 2"=w1983, "Com Port"=w1985, "Ch1"=w1984) -> ("Scale Ch2"=w1986:dbl)  [unwired: 2 out]
        n1332 = local write "Scale 8"(w1986) -> ()
      }
    }
    n1333 = case shown="False" "Scale UP 11" {
      tunnel: w904 -> [_ w1688]
      frame False {
      }
      frame True {
        n1334 = stacked-sequence {
          tunnel: w1688 -> [w1690 w1693 w1697]
          tunnel: [w1690 _ _] -> w1687
          frame #0 {
            w1692 = 10 items=["*RST", "*PWC", "*CA1", "*CA2", "*SS1001", "*SS2001", "*SU1", "*SU2", "*SD1", "*SD2", "*CS1", "*CS2"] ("string to write")
            n1335 = call "Send.vi"("string to write"=w1692, "port number"=w1690) -> ()  [unwired: 1 in]
            n1336 = Wait (ms)(milliseconds to wait=10) -> ()  [unwired: 1 out]
          }
          frame #1 {
            w1695 = 11 items=["*RST", "*PWC", "*CA1", "*CA2", "*SS1001", "*SS2001", "*SU1", "*SU2", "*SD1", "*SD2", "*CS1", "*CS2"] ("string to write")
            n1337 = call "Send.vi"("string to write"=w1695, "port number"=w1693) -> ()  [unwired: 1 in]
            n1338 = Wait (ms)(milliseconds to wait=10) -> ()  [unwired: 1 out]
          }
          frame #2 {
            w1698 = 6 items=["*RST", "*PWC", "*CA1", "*CA2", "*SS1001", "*SS2001", "*SU1", "*SU2", "*SD1", "*SD2"] ("string to write")
            n1339 = call "Send.vi"("string to write"=w1698, "port number"=w1697) -> ()  [unwired: 1 in]
            n1340 = Wait (ms)(milliseconds to wait=10) -> ()  [unwired: 1 out]
          }
        }
        n1341 = local write "Scale UP 11"(FALSE) -> ()
        n1342 = local read "Ch 12 Status"() -> (w1685:bool)
        n1343 = local read "Ch 11 Status"() -> (w1686:bool)
        n1344 = call "Read Scale Ch 1.vi"("Ch2"=w1685, "Com Port"=w1687, "Ch 1"=w1686) -> ("Scale 1Ch"=w1684:dbl)  [unwired: 2 out]
        n1345 = local write "Scale 11"(w1684) -> ()
      }
    }
    n1346 = case shown="False" "Scale UP 15" {
      tunnel: w884 -> [_ w1532]
      frame False {
      }
      frame True {
        n1347 = stacked-sequence {
          tunnel: w1532 -> [w1534 w1537 w1541]
          tunnel: [w1534 _ _] -> w1531
          frame #0 {
            w1536 = 10 items=["*RST", "*PWC", "*CA1", "*CA2", "*SS1001", "*SS2001", "*SU1", "*SU2", "*SD1", "*SD2", "*CS1", "*CS2"] ("string to write")
            n1348 = call "Send.vi"("string to write"=w1536, "port number"=w1534) -> ()  [unwired: 1 in]
            n1349 = Wait (ms)(milliseconds to wait=10) -> ()  [unwired: 1 out]
          }
          frame #1 {
            w1539 = 11 items=["*RST", "*PWC", "*CA1", "*CA2", "*SS1001", "*SS2001", "*SU1", "*SU2", "*SD1", "*SD2", "*CS1", "*CS2"] ("string to write")
            n1350 = call "Send.vi"("string to write"=w1539, "port number"=w1537) -> ()  [unwired: 1 in]
            n1351 = Wait (ms)(milliseconds to wait=10) -> ()  [unwired: 1 out]
          }
          frame #2 {
            w1542 = 6 items=["*RST", "*PWC", "*CA1", "*CA2", "*SS1001", "*SS2001", "*SU1", "*SU2", "*SD1", "*SD2"] ("string to write")
            n1352 = call "Send.vi"("string to write"=w1542, "port number"=w1541) -> ()  [unwired: 1 in]
            n1353 = Wait (ms)(milliseconds to wait=10) -> ()  [unwired: 1 out]
          }
        }
        n1354 = local write "Scale UP 15"(FALSE) -> ()
        n1355 = local read "Ch 16 Status"() -> (w1529:bool)
        n1356 = local read "Ch 15 Status"() -> (w1530:bool)
        n1357 = call "Read Scale Ch 1.vi"("Ch2"=w1529, "Com Port"=w1531, "Ch 1"=w1530) -> ("Scale 1Ch"=w1528:dbl)  [unwired: 2 out]
        n1358 = local write "Scale 15"(w1528) -> ()
      }
    }
    n1359 = case shown="False" "Scale UP 7" {
      tunnel: w939 -> [_ w2032]
      frame False {
      }
      frame True {
        n1360 = stacked-sequence {
          tunnel: w2032 -> [w2034 w2037 w2041]
          tunnel: [w2034 _ _] -> w2031
          frame #0 {
            w2036 = 10 items=["*RST", "*PWC", "*CA1", "*CA2", "*SS1001", "*SS2001", "*SU1", "*SU2", "*SD1", "*SD2", "*CS1", "*CS2"] ("string to write")
            n1361 = call "Send.vi"("string to write"=w2036, "port number"=w2034) -> ()  [unwired: 1 in]
            n1362 = Wait (ms)(milliseconds to wait=10) -> ()  [unwired: 1 out]
          }
          frame #1 {
            w2039 = 11 items=["*RST", "*PWC", "*CA1", "*CA2", "*SS1001", "*SS2001", "*SU1", "*SU2", "*SD1", "*SD2", "*CS1", "*CS2"] ("string to write")
            n1363 = call "Send.vi"("string to write"=w2039, "port number"=w2037) -> ()  [unwired: 1 in]
            n1364 = Wait (ms)(milliseconds to wait=10) -> ()  [unwired: 1 out]
          }
          frame #2 {
            w2042 = 6 items=["*RST", "*PWC", "*CA1", "*CA2", "*SS1001", "*SS2001", "*SU1", "*SU2", "*SD1", "*SD2"] ("string to write")
            n1365 = call "Send.vi"("string to write"=w2042, "port number"=w2041) -> ()  [unwired: 1 in]
            n1366 = Wait (ms)(milliseconds to wait=10) -> ()  [unwired: 1 out]
          }
        }
        n1367 = local write "Scale UP 7"(FALSE) -> ()
        n1368 = local read "Ch 08 Status"() -> (w2029:bool)
        n1369 = local read "Ch 07 Status"() -> (w2030:bool)
        n1370 = call "Read Scale Ch 1.vi"("Ch2"=w2029, "Com Port"=w2031, "Ch 1"=w2030) -> ("Scale 1Ch"=w2028:dbl)  [unwired: 2 out]
        n1371 = local write "Scale 7"(w2028) -> ()
      }
    }
    n1372 = local write "Program Status:"("Logging..." ("Program Status")) -> ()
    n1373 = local read "Com Port 2"() -> (w957:refnum<visa-resource-name>)
    n1374 = local read "Com Port 2"() -> (w955:refnum<visa-resource-name>)
    n1375 = local read "Com Port 6"() -> (w906:refnum<visa-resource-name>)
    n1376 = local read "Com Port 8"() -> (w886:refnum<visa-resource-name>)
    n1377 = local read "Com Port 4"() -> (w937:refnum<visa-resource-name>)
    n1378 = local read "Com Port 8"() -> (w888:refnum<visa-resource-name>)
    n1379 = local read "Com Port 4"() -> (w935:refnum<visa-resource-name>)
    n1380 = local read "Com Port 6"() -> (w908:refnum<visa-resource-name>)
    n1381 = case shown="False" "Scale Down 3" {
      tunnel: w957 -> [_ w2173]
      frame False {
      }
      frame True {
        n1382 = stacked-sequence {
          tunnel: w2173 -> [w2175 w2178 w2182]
          tunnel: [w2175 _ _] -> w2172
          frame #0 {
            w2177 = 10 items=["*RST", "*PWC", "*CA1", "*CA2", "*SS1001", "*SS2001", "*SU1", "*SU2", "*SD1", "*SD2", "*CS1", "*CS2"] ("string to write")
            n1383 = call "Send.vi"("string to write"=w2177, "port number"=w2175) -> ()  [unwired: 1 in]
            n1384 = Wait (ms)(milliseconds to wait=10) -> ()  [unwired: 1 out]
          }
          frame #1 {
            w2180 = 11 items=["*RST", "*PWC", "*CA1", "*CA2", "*SS1001", "*SS2001", "*SU1", "*SU2", "*SD1", "*SD2", "*CS1", "*CS2"] ("string to write")
            n1385 = call "Send.vi"("string to write"=w2180, "port number"=w2178) -> ()  [unwired: 1 in]
            n1386 = Wait (ms)(milliseconds to wait=10) -> ()  [unwired: 1 out]
          }
          frame #2 {
            w2183 = 8 items=["*RST", "*PWC", "*CA1", "*CA2", "*SS1001", "*SS2001", "*SU1", "*SU2", "*SD1", "*SD2"] ("string to write")
            n1387 = call "Send.vi"("string to write"=w2183, "port number"=w2182) -> ()  [unwired: 1 in]
            n1388 = Wait (ms)(milliseconds to wait=10) -> ()  [unwired: 1 out]
          }
        }
        n1389 = local write "Scale Down 3"(FALSE) -> ()
        n1390 = local read "Ch 03 Status"() -> (w2171:bool)
        n1391 = local read "Ch 04 Status"() -> (w2169:bool)
        n1392 = call "Read Scale Ch 1.vi"("Ch2"=w2169, "Com Port"=w2172, "Ch 1"=w2171) -> ("Scale 1Ch"=w2170:dbl)  [unwired: 2 out]
        n1393 = local write "Scale 3"(w2170) -> ()
      }
    }
    n1394 = case shown="False" "Scale Down 15" {
      tunnel: w886 -> [_ w1517]
      frame False {
      }
      frame True {
        n1395 = stacked-sequence {
          tunnel: w1517 -> [w1519 w1522 w1526]
          tunnel: [w1519 _ _] -> w1516
          frame #0 {
            w1521 = 10 items=["*RST", "*PWC", "*CA1", "*CA2", "*SS1001", "*SS2001", "*SU1", "*SU2", "*SD1", "*SD2", "*CS1", "*CS2"] ("string to write")
            n1396 = call "Send.vi"("string to write"=w1521, "port number"=w1519) -> ()  [unwired: 1 in]
            n1397 = Wait (ms)(milliseconds to wait=10) -> ()  [unwired: 1 out]
          }
          frame #1 {
            w1524 = 11 items=["*RST", "*PWC", "*CA1", "*CA2", "*SS1001", "*SS2001", "*SU1", "*SU2", "*SD1", "*SD2", "*CS1", "*CS2"] ("string to write")
            n1398 = call "Send.vi"("string to write"=w1524, "port number"=w1522) -> ()  [unwired: 1 in]
            n1399 = Wait (ms)(milliseconds to wait=10) -> ()  [unwired: 1 out]
          }
          frame #2 {
            w1527 = 8 items=["*RST", "*PWC", "*CA1", "*CA2", "*SS1001", "*SS2001", "*SU1", "*SU2", "*SD1", "*SD2"] ("string to write")
            n1400 = call "Send.vi"("string to write"=w1527, "port number"=w1526) -> ()  [unwired: 1 in]
            n1401 = Wait (ms)(milliseconds to wait=10) -> ()  [unwired: 1 out]
          }
        }
        n1402 = local write "Scale Down 15"(FALSE) -> ()
        n1403 = local read "Ch 15 Status"() -> (w1515:bool)
        n1404 = local read "Ch 16 Status"() -> (w1513:bool)
        n1405 = call "Read Scale Ch 1.vi"("Ch2"=w1513, "Com Port"=w1516, "Ch 1"=w1515) -> ("Scale 1Ch"=w1514:dbl)  [unwired: 2 out]
        n1406 = local write "Scale 15"(w1514) -> ()
      }
    }
    n1407 = case shown="False" "Scale Down 4" {
      tunnel: w955 -> [_ w2158]
      frame False {
      }
      frame True {
        n1408 = stacked-sequence {
          tunnel: w2158 -> [w2160 w2163 w2167]
          tunnel: [w2160 _ _] -> w2157
          frame #0 {
            w2162 = 10 items=["*RST", "*PWC", "*CA1", "*CA2", "*SS1001", "*SS2001", "*SU1", "*SU2", "*SD1", "*SD2", "*CS1", "*CS2"] ("string to write")
            n1409 = call "Send.vi"("string to write"=w2162, "port number"=w2160) -> ()  [unwired: 1 in]
            n1410 = Wait (ms)(milliseconds to wait=10) -> ()  [unwired: 1 out]
          }
          frame #1 {
            w2165 = 11 items=["*RST", "*PWC", "*CA1", "*CA2", "*SS1001", "*SS2001", "*SU1", "*SU2", "*SD1", "*SD2", "*CS1", "*CS2"] ("string to write")
            n1411 = call "Send.vi"("string to write"=w2165, "port number"=w2163) -> ()  [unwired: 1 in]
            n1412 = Wait (ms)(milliseconds to wait=10) -> ()  [unwired: 1 out]
          }
          frame #2 {
            w2168 = 9 items=["*RST", "*PWC", "*CA1", "*CA2", "*SS1001", "*SS2001", "*SU1", "*SU2", "*SD1", "*SD2"] ("string to write")
            n1413 = call "Send.vi"("string to write"=w2168, "port number"=w2167) -> ()  [unwired: 1 in]
            n1414 = Wait (ms)(milliseconds to wait=10) -> ()  [unwired: 1 out]
          }
        }
        n1415 = local write "Scale Down 4"(FALSE) -> ()
        n1416 = local read "Ch 03 Status"() -> (w2155:bool)
        n1417 = local read "Ch 04 Status"() -> (w2154:bool)
        n1418 = call "Read Scale Ch 2.vi"("Ch 2"=w2154, "Com Port"=w2157, "Ch1"=w2155) -> ("Scale Ch2"=w2156:dbl)  [unwired: 2 out]
        n1419 = local write "Scale 4"(w2156) -> ()
      }
    }
    n1420 = case shown="False" "Scale Down 7" {
      tunnel: w937 -> [_ w2017]
      frame False {
      }
      frame True {
        n1421 = stacked-sequence {
          tunnel: w2017 -> [w2019 w2022 w2026]
          tunnel: [w2019 _ _] -> w2016
          frame #0 {
            w2021 = 10 items=["*RST", "*PWC", "*CA1", "*CA2", "*SS1001", "*SS2001", "*SU1", "*SU2", "*SD1", "*SD2", "*CS1", "*CS2"] ("string to write")
            n1422 = call "Send.vi"("string to write"=w2021, "port number"=w2019) -> ()  [unwired: 1 in]
            n1423 = Wait (ms)(milliseconds to wait=10) -> ()  [unwired: 1 out]
          }
          frame #1 {
            w2024 = 11 items=["*RST", "*PWC", "*CA1", "*CA2", "*SS1001", "*SS2001", "*SU1", "*SU2", "*SD1", "*SD2", "*CS1", "*CS2"] ("string to write")
            n1424 = call "Send.vi"("string to write"=w2024, "port number"=w2022) -> ()  [unwired: 1 in]
            n1425 = Wait (ms)(milliseconds to wait=10) -> ()  [unwired: 1 out]
          }
          frame #2 {
            w2027 = 8 items=["*RST", "*PWC", "*CA1", "*CA2", "*SS1001", "*SS2001", "*SU1", "*SU2", "*SD1", "*SD2"] ("string to write")
            n1426 = call "Send.vi"("string to write"=w2027, "port number"=w2026) -> ()  [unwired: 1 in]
            n1427 = Wait (ms)(milliseconds to wait=10) -> ()  [unwired: 1 out]
          }
        }
        n1428 = local write "Scale Down 7"(FALSE) -> ()
        n1429 = local read "Ch 07 Status"() -> (w2015:bool)
        n1430 = local read "Ch 08 Status"() -> (w2013:bool)
        n1431 = call "Read Scale Ch 1.vi"("Ch2"=w2013, "Com Port"=w2016, "Ch 1"=w2015) -> ("Scale 1Ch"=w2014:dbl)  [unwired: 2 out]
        n1432 = local write "Scale 7"(w2014) -> ()
      }
    }
    n1433 = case shown="True" "Scale Down 12" {
      tunnel: w908 -> [_ w1658]
      frame False {
      }
      frame True {
        n1434 = stacked-sequence {
          tunnel: w1658 -> [w1660 w1663 w1667]
          tunnel: [w1660 _ _] -> w1657
          frame #0 {
            w1662 = 10 items=["*RST", "*PWC", "*CA1", "*CA2", "*SS1001", "*SS2001", "*SU1", "*SU2", "*SD1", "*SD2", "*CS1", "*CS2"] ("string to write")
            n1435 = call "Send.vi"("string to write"=w1662, "port number"=w1660) -> ()  [unwired: 1 in]
            n1436 = Wait (ms)(milliseconds to wait=10) -> ()  [unwired: 1 out]
          }
          frame #1 {
            w1665 = 11 items=["*RST", "*PWC", "*CA1", "*CA2", "*SS1001", "*SS2001", "*SU1", "*SU2", "*SD1", "*SD2", "*CS1", "*CS2"] ("string to write")
            n1437 = call "Send.vi"("string to write"=w1665, "port number"=w1663) -> ()  [unwired: 1 in]
            n1438 = Wait (ms)(milliseconds to wait=10) -> ()  [unwired: 1 out]
          }
          frame #2 {
            w1668 = 9 items=["*RST", "*PWC", "*CA1", "*CA2", "*SS1001", "*SS2001", "*SU1", "*SU2", "*SD1", "*SD2"] ("string to write")
            n1439 = call "Send.vi"("string to write"=w1668, "port number"=w1667) -> ()  [unwired: 1 in]
            n1440 = Wait (ms)(milliseconds to wait=10) -> ()  [unwired: 1 out]
          }
        }
        n1441 = local write "Scale Down 12"(FALSE) -> ()
        n1442 = local read "Ch 11 Status"() -> (w1655:bool)
        n1443 = local read "Ch 12 Status"() -> (w1654:bool)
        n1444 = call "Read Scale Ch 2.vi"("Ch 2"=w1654, "Com Port"=w1657, "Ch1"=w1655) -> ("Scale Ch2"=w1656:dbl)  [unwired: 2 out]
        n1445 = local write "Scale 12"(w1656) -> ()
      }
    }
    n1446 = case shown="False" "Scale Down 16" {
      tunnel: w888 -> [_ w1502]
      frame False {
      }
      frame True {
        n1447 = stacked-sequence {
          tunnel: w1502 -> [w1504 w1507 w1511]
          tunnel: [w1504 _ _] -> w1501
          frame #0 {
            w1506 = 10 items=["*RST", "*PWC", "*CA1", "*CA2", "*SS1001", "*SS2001", "*SU1", "*SU2", "*SD1", "*SD2", "*CS1", "*CS2"] ("string to write")
            n1448 = call "Send.vi"("string to write"=w1506, "port number"=w1504) -> ()  [unwired: 1 in]
            n1449 = Wait (ms)(milliseconds to wait=10) -> ()  [unwired: 1 out]
          }
          frame #1 {
            w1509 = 11 items=["*RST", "*PWC", "*CA1", "*CA2", "*SS1001", "*SS2001", "*SU1", "*SU2", "*SD1", "*SD2", "*CS1", "*CS2"] ("string to write")
            n1450 = call "Send.vi"("string to write"=w1509, "port number"=w1507) -> ()  [unwired: 1 in]
            n1451 = Wait (ms)(milliseconds to wait=10) -> ()  [unwired: 1 out]
          }
          frame #2 {
            w1512 = 9 items=["*RST", "*PWC", "*CA1", "*CA2", "*SS1001", "*SS2001", "*SU1", "*SU2", "*SD1", "*SD2"] ("string to write")
            n1452 = call "Send.vi"("string to write"=w1512, "port number"=w1511) -> ()  [unwired: 1 in]
            n1453 = Wait (ms)(milliseconds to wait=10) -> ()  [unwired: 1 out]
          }
        }
        n1454 = local write "Scale Down 16"(FALSE) -> ()
        n1455 = local read "Ch 15 Status"() -> (w1499:bool)
        n1456 = local read "Ch 16 Status"() -> (w1498:bool)
        n1457 = call "Read Scale Ch 2.vi"("Ch 2"=w1498, "Com Port"=w1501, "Ch1"=w1499) -> ("Scale Ch2"=w1500:dbl)  [unwired: 2 out]
        n1458 = local write "Scale 16"(w1500) -> ()
      }
    }
    n1459 = case shown="False" "Scale Down 8" {
      tunnel: w935 -> [_ w2002]
      frame False {
      }
      frame True {
        n1460 = stacked-sequence {
          tunnel: w2002 -> [w2004 w2007 w2011]
          tunnel: [w2004 _ _] -> w2001
          frame #0 {
            w2006 = 10 items=["*RST", "*PWC", "*CA1", "*CA2", "*SS1001", "*SS2001", "*SU1", "*SU2", "*SD1", "*SD2", "*CS1", "*CS2"] ("string to write")
            n1461 = call "Send.vi"("string to write"=w2006, "port number"=w2004) -> ()  [unwired: 1 in]
            n1462 = Wait (ms)(milliseconds to wait=10) -> ()  [unwired: 1 out]
          }
          frame #1 {
            w2009 = 11 items=["*RST", "*PWC", "*CA1", "*CA2", "*SS1001", "*SS2001", "*SU1", "*SU2", "*SD1", "*SD2", "*CS1", "*CS2"] ("string to write")
            n1463 = call "Send.vi"("string to write"=w2009, "port number"=w2007) -> ()  [unwired: 1 in]
            n1464 = Wait (ms)(milliseconds to wait=10) -> ()  [unwired: 1 out]
          }
          frame #2 {
            w2012 = 9 items=["*RST", "*PWC", "*CA1", "*CA2", "*SS1001", "*SS2001", "*SU1", "*SU2", "*SD1", "*SD2"] ("string to write")
            n1465 = call "Send.vi"("string to write"=w2012, "port number"=w2011) -> ()  [unwired: 1 in]
            n1466 = Wait (ms)(milliseconds to wait=10) -> ()  [unwired: 1 out]
          }
        }
        n1467 = local write "Scale Down 8"(FALSE) -> ()
        n1468 = local read "Ch 07 Status"() -> (w1999:bool)
        n1469 = local read "Ch 08 Status"() -> (w1998:bool)
        n1470 = call "Read Scale Ch 2.vi"("Ch 2"=w1998, "Com Port"=w2001, "Ch1"=w1999) -> ("Scale Ch2"=w2000:dbl)  [unwired: 2 out]
        n1471 = local write "Scale 8"(w2000) -> ()
      }
    }
    n1472 = case shown="True" "Scale Down 11" {
      tunnel: w906 -> [_ w1673]
      frame False {
      }
      frame True {
        n1473 = stacked-sequence {
          tunnel: w1673 -> [w1675 w1678 w1682]
          tunnel: [w1675 _ _] -> w1672
          frame #0 {
            w1677 = 10 items=["*RST", "*PWC", "*CA1", "*CA2", "*SS1001", "*SS2001", "*SU1", "*SU2", "*SD1", "*SD2", "*CS1", "*CS2"] ("string to write")
            n1474 = call "Send.vi"("string to write"=w1677, "port number"=w1675) -> ()  [unwired: 1 in]
            n1475 = Wait (ms)(milliseconds to wait=10) -> ()  [unwired: 1 out]
          }
          frame #1 {
            w1680 = 11 items=["*RST", "*PWC", "*CA1", "*CA2", "*SS1001", "*SS2001", "*SU1", "*SU2", "*SD1", "*SD2", "*CS1", "*CS2"] ("string to write")
            n1476 = call "Send.vi"("string to write"=w1680, "port number"=w1678) -> ()  [unwired: 1 in]
            n1477 = Wait (ms)(milliseconds to wait=10) -> ()  [unwired: 1 out]
          }
          frame #2 {
            w1683 = 8 items=["*RST", "*PWC", "*CA1", "*CA2", "*SS1001", "*SS2001", "*SU1", "*SU2", "*SD1", "*SD2"] ("string to write")
            n1478 = call "Send.vi"("string to write"=w1683, "port number"=w1682) -> ()  [unwired: 1 in]
            n1479 = Wait (ms)(milliseconds to wait=10) -> ()  [unwired: 1 out]
          }
        }
        n1480 = local write "Scale Down 11"(FALSE) -> ()
        n1481 = local read "Ch 11 Status"() -> (w1671:bool)
        n1482 = local read "Ch 12 Status"() -> (w1669:bool)
        n1483 = call "Read Scale Ch 1.vi"("Ch2"=w1669, "Com Port"=w1672, "Ch 1"=w1671) -> ("Scale 1Ch"=w1670:dbl)  [unwired: 2 out]
        n1484 = local write "Scale 11"(w1670) -> ()
      }
    }
    n1485 = Format Date/Time String(time format string (%c)="%H:%M:%S%3u") -> (date/time string=w874:string)  [unwired: 2 in]
    n1486 = local read "Com Port 6"() -> (w912:refnum<visa-resource-name>)
    n1487 = local read "Com Port 8"() -> (w892:refnum<visa-resource-name>)
    n1488 = local read "Com Port 2"() -> (w951:refnum<visa-resource-name>)
    n1489 = local read "Com Port 4"() -> (w931:refnum<visa-resource-name>)
    n1490 = local write "Time"(w874) -> ()
    n1491 = case shown="True" "Send 6" {
      tunnel: w912 -> [_ w1621]
      frame False {
      }
      frame True {
        n1492 = stacked-sequence {
          tunnel: w1621 -> [w1626 w1632 w1638]
          frame #0 {
            n1493 = local read "Option"() -> (w1624:string)
            n1494 = local read "Command"() -> (w1623:i32)
            n1495 = call "Send.vi"("string to write"=w1623, "port number"=w1626, "Option"=w1624) -> ()
            n1496 = Wait (ms)(milliseconds to wait=10) -> ()  [unwired: 1 out]
          }
          frame #1 {
            n1497 = local read "Ch 11 Status"() -> (w1629:bool)
            n1498 = local read "Ch 12 Status"() -> (w1628:bool)
            n1499 = call "Read Scale Ch 1.vi"("Ch2"=w1628, "Com Port"=w1632, "Ch 1"=w1629) -> ("Scale 1Ch"=w1631:dbl, "Trigger Status Ch1"=w1630:bool, "Wavelength"=w1627:u32)
            n1500 = local write "Trigger ch 11"(w1630) -> ()
            n1501 = local write "Wavelength 11"(w1627) -> ()
            n1502 = local write "Scale 11"(w1631) -> ()
          }
          frame #2 {
            n1503 = local read "Ch 11 Status"() -> (w1633:bool)
            n1504 = local read "Ch 12 Status"() -> (w1635:bool)
            n1505 = call "Read Scale Ch 2.vi"("Ch 2"=w1635, "Com Port"=w1638, "Ch1"=w1633) -> ("Scale Ch2"=w1636:dbl, "External Trigger Ch2"=w1634:bool, "Wavelength"=w1637:u32)
            n1506 = local write "Wavelength 12"(w1637) -> ()
            n1507 = local write "Trigger ch 12"(w1634) -> ()
            n1508 = local write "Scale 12"(w1636) -> ()
          }
        }
        n1509 = local write "Send 6"(FALSE) -> ()
      }
    }
    n1510 = case shown="True" "Send 8" {
      tunnel: w892 -> [_ w1465]
      frame False {
      }
      frame True {
        n1511 = stacked-sequence {
          tunnel: w1465 -> [w1470 w1476 w1482]
          frame #0 {
            n1512 = local read "Option"() -> (w1468:string)
            n1513 = local read "Command"() -> (w1467:i32)
            n1514 = call "Send.vi"("string to write"=w1467, "port number"=w1470, "Option"=w1468) -> ()
            n1515 = Wait (ms)(milliseconds to wait=10) -> ()  [unwired: 1 out]
          }
          frame #1 {
            n1516 = local read "Ch 15 Status"() -> (w1473:bool)
            n1517 = local read "Ch 16 Status"() -> (w1472:bool)
            n1518 = call "Read Scale Ch 1.vi"("Ch2"=w1472, "Com Port"=w1476, "Ch 1"=w1473) -> ("Scale 1Ch"=w1475:dbl, "Trigger Status Ch1"=w1474:bool, "Wavelength"=w1471:u32)
            n1519 = local write "Trigger ch 15"(w1474) -> ()
            n1520 = local write "Wavelength 15"(w1471) -> ()
            n1521 = local write "Scale 15"(w1475) -> ()
          }
          frame #2 {
            n1522 = local read "Ch 15 Status"() -> (w1477:bool)
            n1523 = local read "Ch 16 Status"() -> (w1479:bool)
            n1524 = call "Read Scale Ch 2.vi"("Ch 2"=w1479, "Com Port"=w1482, "Ch1"=w1477) -> ("Scale Ch2"=w1480:dbl, "External Trigger Ch2"=w1478:bool, "Wavelength"=w1481:u32)
            n1525 = local write "Wavelength 16"(w1481) -> ()
            n1526 = local write "Trigger ch 16"(w1478) -> ()
            n1527 = local write "Scale 16"(w1480) -> ()
          }
        }
        n1528 = local write "Send 8"(FALSE) -> ()
      }
    }
    n1529 = case shown="False" "Send 2" {
      tunnel: w951 -> [_ w2121]
      frame False {
      }
      frame True {
        n1530 = stacked-sequence {
          tunnel: w2121 -> [w2126 w2131 w2134]
          frame #0 {
            n1531 = local read "Option"() -> (w2124:string)
            n1532 = local read "Command"() -> (w2123:i32)
            n1533 = call "Send.vi"("string to write"=w2123, "port number"=w2126, "Option"=w2124) -> ()
            n1534 = Wait (ms)(milliseconds to wait=10) -> ()  [unwired: 1 out]
          }
          frame #1 {
            n1535 = local read "Ch 04 Status"() -> (w2129:bool)
            n1536 = local read "Ch 03 Status"() -> (w2130:bool)
            n1537 = call "Read Scale Ch 1.vi"("Ch2"=w2129, "Com Port"=w2131, "Ch 1"=w2130) -> ("Scale 1Ch"=w2128:dbl, "Trigger Status Ch1"=w2127:bool, "Wavelength"=w2132:u32)
            n1538 = local write "Trigger ch 3"(w2127) -> ()
            n1539 = local write "Wavelength 3"(w2132) -> ()
            n1540 = local write "Scale 3"(w2128) -> ()
          }
          frame #2 {
            n1541 = local read "Ch 03 Status"() -> (w2136:bool)
            n1542 = local read "Ch 04 Status"() -> (w2137:bool)
            n1543 = call "Read Scale Ch 2.vi"("Ch 2"=w2137, "Com Port"=w2134, "Ch1"=w2136) -> ("Scale Ch2"=w2135:dbl, "External Trigger Ch2"=w2133:bool, "Wavelength"=w2138:u32)
            n1544 = local write "Trigger ch 4"(w2133) -> ()
            n1545 = local write "Wavelength 4"(w2138) -> ()
            n1546 = local write "Scale 4"(w2135) -> ()
          }
        }
        n1547 = local write "Send 2"(FALSE) -> ()
      }
    }
    n1548 = case shown="True" "Send 4" {
      tunnel: w931 -> [_ w1965]
      frame False {
      }
      frame True {
        n1549 = stacked-sequence {
          tunnel: w1965 -> [w1970 w1975 w1978]
          frame #0 {
            n1550 = local read "Option"() -> (w1968:string)
            n1551 = local read "Command"() -> (w1967:i32)
            n1552 = call "Send.vi"("string to write"=w1967, "port number"=w1970, "Option"=w1968) -> ()
            n1553 = Wait (ms)(milliseconds to wait=10) -> ()  [unwired: 1 out]
          }
          frame #1 {
            n1554 = local read "Ch 08 Status"() -> (w1972:bool)
            n1555 = local read "Ch 07 Status"() -> (w1974:bool)
            n1556 = call "Read Scale Ch 1.vi"("Ch2"=w1972, "Com Port"=w1975, "Ch 1"=w1974) -> ("Scale 1Ch"=w1973:dbl, "Trigger Status Ch1"=w1971:bool, "Wavelength"=w1976:u32)
            n1557 = local write "Trigger ch 7"(w1971) -> ()
            n1558 = local write "Wavelength 7"(w1976) -> ()
            n1559 = local write "Scale 7"(w1973) -> ()
          }
          frame #2 {
            n1560 = local read "Ch 07 Status"() -> (w1980:bool)
            n1561 = local read "Ch 08 Status"() -> (w1981:bool)
            n1562 = call "Read Scale Ch 2.vi"("Ch 2"=w1981, "Com Port"=w1978, "Ch1"=w1980) -> ("Scale Ch2"=w1979:dbl, "External Trigger Ch2"=w1977:bool, "Wavelength"=w1982:u32)
            n1563 = local write "Trigger ch 8"(w1977) -> ()
            n1564 = local write "Wavelength 8"(w1982) -> ()
            n1565 = local write "Scale 8"(w1979) -> ()
          }
        }
        n1566 = local write "Send 4"(FALSE) -> ()
      }
    }
    n1567 = local read "Com Port 1"() -> (w969:refnum<visa-resource-name>)
    n1568 = local read "Com Port 1"() -> (w964:refnum<visa-resource-name>)
    n1569 = local read "Com Port 5"() -> (w925:refnum<visa-resource-name>)
    n1570 = local read "Com Port 3"() -> (w949:refnum<visa-resource-name>)
    n1571 = local read "Com Port 3"() -> (w944:refnum<visa-resource-name>)
    n1572 = local read "Com Port 7"() -> (w898:refnum<visa-resource-name>)
    n1573 = local read "Com Port 7"() -> (w903:refnum<visa-resource-name>)
    n1574 = local read "Com Port 5"() -> (w920:refnum<visa-resource-name>)
    n1575 = Format Date/Time String(time format string (%c)="%Y%m%d") -> (date/time string=w875:string)  [unwired: 2 in]
    n1576 = local read "Date"() -> (w916:string)
    n1577 = case shown="False" "Scale UP 2" {
      tunnel: w964 -> [_ w2221]
      frame False {
      }
      frame True {
        # "If clicked, stop slink reading(*CS1 and *CS2),\nsend scale up ch2 to slink, and read ch2 status"
        n1578 = stacked-sequence {
          tunnel: w2221 -> [w2223 w2228 w2230]
          tunnel: [w2223 _ _] -> w2219
          frame #0 {
            w2225 = 10 items=["*RST", "*PWC", "*CA1", "*CA2", "*SS1001", "*SS2001", "*SU1", "*SU2", "*SD1", "*SD2", "*CS1", "*CS2"] ("string to write")
            n1579 = call "Send.vi"("string to write"=w2225, "port number"=w2223) -> ()  [unwired: 1 in]
            n1580 = Wait (ms)(milliseconds to wait=10) -> ()  [unwired: 1 out]
          }
          frame #1 {
            w2226 = 11 items=["*RST", "*VER", "*CA1", "*CA2", "*SS100", "*SS200", "*SU1", "*SU2", "*SD1", "*SD2", "*CS1", "*CS2", "*AT1", "*AT2", "*AN1", "*AN2", "*PW1", "*PW2", "*TL1", "*TL2", "*ST1", "*ST2", "*ET1", "*ET2", "*EM1", "*EM2", "*SC1", "*SC2"] ("string to write")
            n1581 = call "Send.vi"("string to write"=w2226, "port number"=w2228) -> ()  [unwired: 1 in]
            n1582 = Wait (ms)(milliseconds to wait=10) -> ()  [unwired: 1 out]
          }
          frame #2 {
            w2231 = 7 items=["*RST", "*PWC", "*CA1", "*CA2", "*SS1001", "*SS2001", "*SU1", "*SU2", "*SD1", "*SD2"] ("string to write")
            n1583 = call "Send.vi"("string to write"=w2231, "port number"=w2230) -> ()  [unwired: 1 in]
            n1584 = Wait (ms)(milliseconds to wait=10) -> ()  [unwired: 1 out]
          }
        }
        n1585 = local write "Scale UP 2"(FALSE) -> ()
        n1586 = local read "Ch 02 Status"() -> (w2217:bool)
        n1587 = local read "Ch 01 Status"() -> (w2218:bool)
        n1588 = call "Read Scale Ch 2.vi"("Ch 2"=w2217, "Com Port"=w2219, "Ch1"=w2218) -> ("Scale Ch2"=w2220:dbl)  [unwired: 2 out]
        n1589 = local write "Scale 2"(w2220) -> ()
      }
    }
    n1590 = case shown="True" "Scale UP" {
      tunnel: w969 -> [_ w2266]
      frame False {
      }
      frame True {
        # "If clicked, stop slink reading(*CS1 and *CS2),\nsend scale up ch1 to slink, and read ch1 status"
        n1591 = stacked-sequence {
          tunnel: w2266 -> [w2268 w2271 w2275]
          tunnel: [w2268 _ _] -> w2265
          frame #0 {
            w2270 = 10 items=["*RST", "*PWC", "*CA1", "*CA2", "*SS1001", "*SS2001", "*SU1", "*SU2", "*SD1", "*SD2", "*CS1", "*CS2"] ("string to write")
            n1592 = call "Send.vi"("string to write"=w2270, "port number"=w2268) -> ()  [unwired: 1 in]
            n1593 = Wait (ms)(milliseconds to wait=10) -> ()  [unwired: 1 out]
          }
          frame #1 {
            w2273 = 11 items=["*RST", "*PWC", "*CA1", "*CA2", "*SS1001", "*SS2001", "*SU1", "*SU2", "*SD1", "*SD2", "*CS1", "*CS2"] ("string to write")
            n1594 = call "Send.vi"("string to write"=w2273, "port number"=w2271) -> ()  [unwired: 1 in]
            n1595 = Wait (ms)(milliseconds to wait=10) -> ()  [unwired: 1 out]
          }
          frame #2 {
            w2276 = 6 items=["*RST", "*PWC", "*CA1", "*CA2", "*SS1001", "*SS2001", "*SU1", "*SU2", "*SD1", "*SD2"] ("string to write")
            n1596 = call "Send.vi"("string to write"=w2276, "port number"=w2275) -> ()  [unwired: 1 in]
            n1597 = Wait (ms)(milliseconds to wait=10) -> ()  [unwired: 1 out]
          }
        }
        n1598 = local write "Scale UP"(FALSE) -> ()
        n1599 = local read "Ch 01 Status"() -> (w2264:bool)
        n1600 = local read "Ch 02 Status"() -> (w2263:bool)
        n1601 = call "Read Scale Ch 1.vi"("Ch2"=w2263, "Com Port"=w2265, "Ch 1"=w2264) -> ("Scale 1Ch"=w2262:dbl)  [unwired: 2 out]
        n1602 = local write "Scale 1"(w2262) -> ()
      }
    }
    n1603 = case shown="False" "Scale UP 14" {
      tunnel: w898 -> [_ w1565]
      frame False {
      }
      frame True {
        n1604 = stacked-sequence {
          tunnel: w1565 -> [w1567 w1572 w1574]
          tunnel: [w1567 _ _] -> w1563
          frame #0 {
            w1569 = 10 items=["*RST", "*PWC", "*CA1", "*CA2", "*SS1001", "*SS2001", "*SU1", "*SU2", "*SD1", "*SD2", "*CS1", "*CS2"] ("string to write")
            n1605 = call "Send.vi"("string to write"=w1569, "port number"=w1567) -> ()  [unwired: 1 in]
            n1606 = Wait (ms)(milliseconds to wait=10) -> ()  [unwired: 1 out]
          }
          frame #1 {
            w1570 = 11 items=["*RST", "*VER", "*CA1", "*CA2", "*SS100", "*SS200", "*SU1", "*SU2", "*SD1", "*SD2", "*CS1", "*CS2", "*AT1", "*AT2", "*AN1", "*AN2", "*PW1", "*PW2", "*TL1", "*TL2", "*ST1", "*ST2", "*ET1", "*ET2", "*EM1", "*EM2", "*SC1", "*SC2"] ("string to write")
            n1607 = call "Send.vi"("string to write"=w1570, "port number"=w1572) -> ()  [unwired: 1 in]
            n1608 = Wait (ms)(milliseconds to wait=10) -> ()  [unwired: 1 out]
          }
          frame #2 {
            w1575 = 7 items=["*RST", "*PWC", "*CA1", "*CA2", "*SS1001", "*SS2001", "*SU1", "*SU2", "*SD1", "*SD2"] ("string to write")
            n1609 = call "Send.vi"("string to write"=w1575, "port number"=w1574) -> ()  [unwired: 1 in]
            n1610 = Wait (ms)(milliseconds to wait=10) -> ()  [unwired: 1 out]
          }
        }
        n1611 = local write "Scale UP 14"(FALSE) -> ()
        n1612 = local read "Ch 14 Status"() -> (w1561:bool)
        n1613 = local read "Ch 13 Status"() -> (w1562:bool)
        n1614 = call "Read Scale Ch 2.vi"("Ch 2"=w1561, "Com Port"=w1563, "Ch1"=w1562) -> ("Scale Ch2"=w1564:dbl)  [unwired: 2 out]
        n1615 = local write "Scale 14"(w1564) -> ()
      }
    }
    n1616 = case shown="False" "Scale UP 13" {
      tunnel: w903 -> [_ w1610]
      frame False {
      }
      frame True {
        n1617 = stacked-sequence {
          tunnel: w1610 -> [w1612 w1615 w1619]
          tunnel: [w1612 _ _] -> w1609
          frame #0 {
            w1614 = 10 items=["*RST", "*PWC", "*CA1", "*CA2", "*SS1001", "*SS2001", "*SU1", "*SU2", "*SD1", "*SD2", "*CS1", "*CS2"] ("string to write")
            n1618 = call "Send.vi"("string to write"=w1614, "port number"=w1612) -> ()  [unwired: 1 in]
            n1619 = Wait (ms)(milliseconds to wait=10) -> ()  [unwired: 1 out]
          }
          frame #1 {
            w1617 = 11 items=["*RST", "*PWC", "*CA1", "*CA2", "*SS1001", "*SS2001", "*SU1", "*SU2", "*SD1", "*SD2", "*CS1", "*CS2"] ("string to write")
            n1620 = call "Send.vi"("string to write"=w1617, "port number"=w1615) -> ()  [unwired: 1 in]
            n1621 = Wait (ms)(milliseconds to wait=10) -> ()  [unwired: 1 out]
          }
          frame #2 {
            w1620 = 6 items=["*RST", "*PWC", "*CA1", "*CA2", "*SS1001", "*SS2001", "*SU1", "*SU2", "*SD1", "*SD2"] ("string to write")
            n1622 = call "Send.vi"("string to write"=w1620, "port number"=w1619) -> ()  [unwired: 1 in]
            n1623 = Wait (ms)(milliseconds to wait=10) -> ()  [unwired: 1 out]
          }
        }
        n1624 = local write "Scale UP 13"(FALSE) -> ()
        n1625 = local read "Ch 14 Status"() -> (w1607:bool)
        n1626 = local read "Ch 13 Status"() -> (w1608:bool)
        n1627 = call "Read Scale Ch 1.vi"("Ch2"=w1607, "Com Port"=w1609, "Ch 1"=w1608) -> ("Scale 1Ch"=w1606:dbl)  [unwired: 2 out]
        n1628 = local write "Scale 13"(w1606) -> ()
      }
    }
    n1629 = case shown="False" "Scale UP 10" {
      tunnel: w925 -> [_ w1909]
      frame False {
      }
      frame True {
        n1630 = stacked-sequence {
          tunnel: w1909 -> [w1911 w1916 w1918]
          tunnel: [w1911 _ _] -> w1907
          frame #0 {
            w1913 = 10 items=["*RST", "*PWC", "*CA1", "*CA2", "*SS1001", "*SS2001", "*SU1", "*SU2", "*SD1", "*SD2", "*CS1", "*CS2"] ("string to write")
            n1631 = call "Send.vi"("string to write"=w1913, "port number"=w1911) -> ()  [unwired: 1 in]
            n1632 = Wait (ms)(milliseconds to wait=10) -> ()  [unwired: 1 out]
          }
          frame #1 {
            w1914 = 11 items=["*RST", "*VER", "*CA1", "*CA2", "*SS100", "*SS200", "*SU1", "*SU2", "*SD1", "*SD2", "*CS1", "*CS2", "*AT1", "*AT2", "*AN1", "*AN2", "*PW1", "*PW2", "*TL1", "*TL2", "*ST1", "*ST2", "*ET1", "*ET2", "*EM1", "*EM2", "*SC1", "*SC2"] ("string to write")
            n1633 = call "Send.vi"("string to write"=w1914, "port number"=w1916) -> ()  [unwired: 1 in]
            n1634 = Wait (ms)(milliseconds to wait=10) -> ()  [unwired: 1 out]
          }
          frame #2 {
            w1919 = 7 items=["*RST", "*PWC", "*CA1", "*CA2", "*SS1001", "*SS2001", "*SU1", "*SU2", "*SD1", "*SD2"] ("string to write")
            n1635 = call "Send.vi"("string to write"=w1919, "port number"=w1918) -> ()  [unwired: 1 in]
            n1636 = Wait (ms)(milliseconds to wait=10) -> ()  [unwired: 1 out]
          }
        }
        n1637 = local write "Scale UP 10"(FALSE) -> ()
        n1638 = local read "Ch 10 Status"() -> (w1906:bool)
        n1639 = local read "Ch 09 Status"() -> (w1905:bool)
        n1640 = call "Read Scale Ch 2.vi"("Ch 2"=w1906, "Com Port"=w1907, "Ch1"=w1905) -> ("Scale Ch2"=w1908:dbl)  [unwired: 2 out]
        n1641 = local write "Scale 10"(w1908) -> ()
      }
    }
    n1642 = case shown="False" "Scale UP 9" {
      tunnel: w920 -> [_ w1954]
      frame False {
      }
      frame True {
        n1643 = stacked-sequence {
          tunnel: w1954 -> [w1956 w1959 w1963]
          tunnel: [w1956 _ _] -> w1953
          frame #0 {
            w1958 = 10 items=["*RST", "*PWC", "*CA1", "*CA2", "*SS1001", "*SS2001", "*SU1", "*SU2", "*SD1", "*SD2", "*CS1", "*CS2"] ("string to write")
            n1644 = call "Send.vi"("string to write"=w1958, "port number"=w1956) -> ()  [unwired: 1 in]
            n1645 = Wait (ms)(milliseconds to wait=10) -> ()  [unwired: 1 out]
          }
          frame #1 {
            w1961 = 11 items=["*RST", "*PWC", "*CA1", "*CA2", "*SS1001", "*SS2001", "*SU1", "*SU2", "*SD1", "*SD2", "*CS1", "*CS2"] ("string to write")
            n1646 = call "Send.vi"("string to write"=w1961, "port number"=w1959) -> ()  [unwired: 1 in]
            n1647 = Wait (ms)(milliseconds to wait=10) -> ()  [unwired: 1 out]
          }
          frame #2 {
            w1964 = 6 items=["*RST", "*PWC", "*CA1", "*CA2", "*SS1001", "*SS2001", "*SU1", "*SU2", "*SD1", "*SD2"] ("string to write")
            n1648 = call "Send.vi"("string to write"=w1964, "port number"=w1963) -> ()  [unwired: 1 in]
            n1649 = Wait (ms)(milliseconds to wait=10) -> ()  [unwired: 1 out]
          }
        }
        n1650 = local write "Scale UP 9"(FALSE) -> ()
        n1651 = local read "Ch 10 Status"() -> (w1950:bool)
        n1652 = local read "Ch 09 Status"() -> (w1952:bool)
        n1653 = call "Read Scale Ch 1.vi"("Ch2"=w1950, "Com Port"=w1953, "Ch 1"=w1952) -> ("Scale 1Ch"=w1951:dbl)  [unwired: 2 out]
        n1654 = local write "Scale 9"(w1951) -> ()
      }
    }
    n1655 = case shown="False" "Scale UP 6" {
      tunnel: w944 -> [_ w2065]
      frame False {
      }
      frame True {
        n1656 = stacked-sequence {
          tunnel: w2065 -> [w2067 w2072 w2074]
          tunnel: [w2067 _ _] -> w2063
          frame #0 {
            w2069 = 10 items=["*RST", "*PWC", "*CA1", "*CA2", "*SS1001", "*SS2001", "*SU1", "*SU2", "*SD1", "*SD2", "*CS1", "*CS2"] ("string to write")
            n1657 = call "Send.vi"("string to write"=w2069, "port number"=w2067) -> ()  [unwired: 1 in]
            n1658 = Wait (ms)(milliseconds to wait=10) -> ()  [unwired: 1 out]
          }
          frame #1 {
            w2070 = 11 items=["*RST", "*VER", "*CA1", "*CA2", "*SS100", "*SS200", "*SU1", "*SU2", "*SD1", "*SD2", "*CS1", "*CS2", "*AT1", "*AT2", "*AN1", "*AN2", "*PW1", "*PW2", "*TL1", "*TL2", "*ST1", "*ST2", "*ET1", "*ET2", "*EM1", "*EM2", "*SC1", "*SC2"] ("string to write")
            n1659 = call "Send.vi"("string to write"=w2070, "port number"=w2072) -> ()  [unwired: 1 in]
            n1660 = Wait (ms)(milliseconds to wait=10) -> ()  [unwired: 1 out]
          }
          frame #2 {
            w2075 = 7 items=["*RST", "*PWC", "*CA1", "*CA2", "*SS1001", "*SS2001", "*SU1", "*SU2", "*SD1", "*SD2"] ("string to write")
            n1661 = call "Send.vi"("string to write"=w2075, "port number"=w2074) -> ()  [unwired: 1 in]
            n1662 = Wait (ms)(milliseconds to wait=10) -> ()  [unwired: 1 out]
          }
        }
        n1663 = local write "Scale UP 6"(FALSE) -> ()
        n1664 = local read "Ch 06 Status"() -> (w2061:bool)
        n1665 = local read "Ch 05 Status"() -> (w2062:bool)
        n1666 = call "Read Scale Ch 2.vi"("Ch 2"=w2061, "Com Port"=w2063, "Ch1"=w2062) -> ("Scale Ch2"=w2064:dbl)  [unwired: 2 out]
        n1667 = local write "Scale 6"(w2064) -> ()
      }
    }
    n1668 = case shown="False" "Scale UP 5" {
      tunnel: w949 -> [_ w2110]
      frame False {
      }
      frame True {
        n1669 = stacked-sequence {
          tunnel: w2110 -> [w2112 w2115 w2119]
          tunnel: [w2112 _ _] -> w2109
          frame #0 {
            w2114 = 10 items=["*RST", "*PWC", "*CA1", "*CA2", "*SS1001", "*SS2001", "*SU1", "*SU2", "*SD1", "*SD2", "*CS1", "*CS2"] ("string to write")
            n1670 = call "Send.vi"("string to write"=w2114, "port number"=w2112) -> ()  [unwired: 1 in]
            n1671 = Wait (ms)(milliseconds to wait=10) -> ()  [unwired: 1 out]
          }
          frame #1 {
            w2117 = 11 items=["*RST", "*PWC", "*CA1", "*CA2", "*SS1001", "*SS2001", "*SU1", "*SU2", "*SD1", "*SD2", "*CS1", "*CS2"] ("string to write")
            n1672 = call "Send.vi"("string to write"=w2117, "port number"=w2115) -> ()  [unwired: 1 in]
            n1673 = Wait (ms)(milliseconds to wait=10) -> ()  [unwired: 1 out]
          }
          frame #2 {
            w2120 = 6 items=["*RST", "*PWC", "*CA1", "*CA2", "*SS1001", "*SS2001", "*SU1", "*SU2", "*SD1", "*SD2"] ("string to write")
            n1674 = call "Send.vi"("string to write"=w2120, "port number"=w2119) -> ()  [unwired: 1 in]
            n1675 = Wait (ms)(milliseconds to wait=10) -> ()  [unwired: 1 out]
          }
        }
        n1676 = local write "Scale UP 5"(FALSE) -> ()
        n1677 = local read "Ch 06 Status"() -> (w2107:bool)
        n1678 = local read "Ch 05 Status"() -> (w2108:bool)
        n1679 = call "Read Scale Ch 1.vi"("Ch2"=w2107, "Com Port"=w2109, "Ch 1"=w2108) -> ("Scale 1Ch"=w2106:dbl)  [unwired: 2 out]
        n1680 = local write "Scale 5"(w2106) -> ()
      }
    }
    n1681 = Equal?(x=w916, y=w875) -> (x = y?=w915:bool)
    n1682 = case shown="False" w915 {
      tunnel: w875 -> [w1699 _]
      frame False {
        # "Date changed! Make new folder and create new files and write headers in to each file\nFor details, see initialization frame 1"
        n1683 = stacked-sequence {
          tunnel: w1699 -> [w1701 _ _ _ _ _ _ _ _ _ _ _ _ _ _ _ _]
          frame #0 {
            n1684 = local read "Base Path"() -> (w1700:path)
            n1685 = local write "Date"(w1701) -> ()
            n1686 = String To Path(string=w1701) -> (path=w1706:path)
            n1687 = Build Path(base path=w1700, name or relative path=w1706) -> (appended path=w1705:path)
            n1688 = call <vilib>:"Check if File or Folder Exists.vi"("path"=w1705) -> ("error out"=w1703:errorcluster, "file or folder exists?"=w1702:bool, "dup path"=w1704:path)  [unwired: 8 in]
            n1689 = case shown="True" w1702 {
              tunnel: w1704 -> [w1708 w1710]
              tunnel: w1703 -> [w1707 _]
              frame False {
                n1690 = Create Folder(path (use dialog)=w1708, error in=w1707) -> (created path=w1709:path)  [unwired: 1 in, 2 out]
                n1691 = local write "Folder"(w1709) -> ()
              }
              frame True {
                n1692 = local write "Folder"(w1710) -> ()
              }
            }
          }
          frame #1 {
            n1693 = local read "Ch 01 Status"() -> (w1711:bool)
            n1694 = case shown="True" w1711 {
              frame False {
              }
              frame True {
                n1695 = local read "Folder"() -> (w1716:path)
                n1696 = Build Path(base path=w1716, name or relative path="FrontEnd1.csv") -> (appended path=w1715:path)
                n1697 = call <vilib>:"Check if File or Folder Exists.vi"("path"=w1715) -> ("file or folder exists?"=w1714:bool, "dup path"=w1713:path)  [unwired: 8 in, 1 out]
                n1698 = case shown="False" w1714 {
                  tunnel: w1713 -> [w1719 w1721]
                  frame False {
                    n1699 = local write "Path Frontend #1"(w1719) -> ()
                    n1700 = call-poly <vilib>:"Write To Spreadsheet File.vi"("delimiter (\\t)"="," ("delimiter (\\t)"), "append to file? (new file:F)"=FALSE, "1D data"=string[] ["Timestamp", "Measured", "Calibrated"], "file path (dialog if empty)"=w1719) -> ()  [unwired: 3 in, 2 out]
                  }
                  frame True {
                    n1701 = local write "Path Frontend #1"(w1721) -> ()
                  }
                }
              }
            }
          }
          frame #2 {
            n1702 = local read "Ch 02 Status"() -> (w1722:bool)
            n1703 = case shown="True" w1722 {
              frame False {
              }
              frame True {
                n1704 = local read "Folder"() -> (w1727:path)
                n1705 = Build Path(base path=w1727, name or relative path="FrontEnd2.csv") -> (appended path=w1726:path)
                n1706 = call <vilib>:"Check if File or Folder Exists.vi"("path"=w1726) -> ("file or folder exists?"=w1725:bool, "dup path"=w1724:path)  [unwired: 8 in, 1 out]
                n1707 = case shown="False" w1725 {
                  tunnel: w1724 -> [w1730 w1732]
                  frame False {
                    n1708 = local write "Path Frontend #2"(w1730) -> ()
                    n1709 = call-poly <vilib>:"Write To Spreadsheet File.vi"("delimiter (\\t)"="," ("delimiter (\\t)"), "append to file? (new file:F)"=FALSE, "1D data"=string[] ["Timestamp", "Measured", "Calibrated"], "file path (dialog if empty)"=w1730) -> ()  [unwired: 3 in, 2 out]
                  }
                  frame True {
                    n1710 = local write "Path Frontend #2"(w1732) -> ()
                  }
                }
              }
            }
          }
          frame #3 {
            n1711 = local read "Ch 03 Status"() -> (w1733:bool)
            n1712 = case shown="True" w1733 {
              frame False {
              }
              frame True {
                n1713 = local read "Folder"() -> (w1735:path)
                n1714 = Build Path(base path=w1735, name or relative path="SLAB2.csv") -> (appended path=w1736:path)
                n1715 = call <vilib>:"Check if File or Folder Exists.vi"("path"=w1736) -> ("file or folder exists?"=w1737:bool, "dup path"=w1738:path)  [unwired: 8 in, 1 out]
                n1716 = case shown="False" w1737 {
                  tunnel: w1738 -> [w1741 w1743]
                  frame False {
                    n1717 = local write "Path SLAB #2"(w1741) -> ()
                    n1718 = call-poly <vilib>:"Write To Spreadsheet File.vi"("delimiter (\\t)"="," ("delimiter (\\t)"), "append to file? (new file:F)"=FALSE, "1D data"=string[] ["Timestamp", "Measured", "Calibrated"], "file path (dialog if empty)"=w1741) -> ()  [unwired: 3 in, 2 out]
                  }
                  frame True {
                    n1719 = local write "Path SLAB #2"(w1743) -> ()
                  }
                }
              }
            }
          }
          frame #4 {
            n1720 = local read "Ch 06 Status"() -> (w1744:bool)
            n1721 = case shown="True" w1744 {
              frame False {
              }
              frame True {
                n1722 = local read "Folder"() -> (w1746:path)
                n1723 = Build Path(base path=w1746, name or relative path="SLAB3.csv") -> (appended path=w1747:path)
                n1724 = call <vilib>:"Check if File or Folder Exists.vi"("path"=w1747) -> ("file or folder exists?"=w1748:bool, "dup path"=w1749:path)  [unwired: 8 in, 1 out]
                n1725 = case shown="False" w1748 {
                  tunnel: w1749 -> [w1752 w1754]
                  frame False {
                    n1726 = local write "Path SLAB #3"(w1752) -> ()
                    n1727 = call-poly <vilib>:"Write To Spreadsheet File.vi"("delimiter (\\t)"="," ("delimiter (\\t)"), "append to file? (new file:F)"=FALSE, "1D data"=string[] ["Timestamp", "Measured", "Calibrated"], "file path (dialog if empty)"=w1752) -> ()  [unwired: 3 in, 2 out]
                  }
                  frame True {
                    n1728 = local write "Path SLAB #3"(w1754) -> ()
                  }
                }
              }
            }
          }
          frame #5 {
            n1729 = local read "Ch 04 Status"() -> (w1755:bool)
            n1730 = case shown="True" w1755 {
              frame False {
              }
              frame True {
                n1731 = local read "Folder"() -> (w1757:path)
                n1732 = Build Path(base path=w1757, name or relative path="SLAB4.csv") -> (appended path=w1758:path)
                n1733 = call <vilib>:"Check if File or Folder Exists.vi"("path"=w1758) -> ("file or folder exists?"=w1759:bool, "dup path"=w1760:path)  [unwired: 8 in, 1 out]
                n1734 = case shown="False" w1759 {
                  tunnel: w1760 -> [w1763 w1765]
                  frame False {
                    n1735 = local write "Path SLAB #4"(w1763) -> ()
                    n1736 = call-poly <vilib>:"Write To Spreadsheet File.vi"("delimiter (\\t)"="," ("delimiter (\\t)"), "append to file? (new file:F)"=FALSE, "1D data"=string[] ["Timestamp", "Measured", "Calibrated"], "file path (dialog if empty)"=w1763) -> ()  [unwired: 3 in, 2 out]
                  }
                  frame True {
                    n1737 = local write "Path SLAB #4"(w1765) -> ()
                  }
                }
              }
            }
          }
          frame #6 {
            n1738 = local read "Ch 05 Status"() -> (w1766:bool)
            n1739 = case shown="True" w1766 {
              frame False {
              }
              frame True {
                n1740 = local read "Folder"() -> (w1768:path)
                n1741 = Build Path(base path=w1768, name or relative path="SLAB5.csv") -> (appended path=w1769:path)
                n1742 = call <vilib>:"Check if File or Folder Exists.vi"("path"=w1769) -> ("file or folder exists?"=w1770:bool, "dup path"=w1771:path)  [unwired: 8 in, 1 out]
                n1743 = case shown="False" w1770 {
                  tunnel: w1771 -> [w1774 w1776]
                  frame False {
                    n1744 = local write "Path SLAB #5"(w1774) -> ()
                    n1745 = call-poly <vilib>:"Write To Spreadsheet File.vi"("delimiter (\\t)"="," ("delimiter (\\t)"), "append to file? (new file:F)"=FALSE, "1D data"=string[] ["Timestamp", "Measured", "Calibrated"], "file path (dialog if empty)"=w1774) -> ()  [unwired: 3 in, 2 out]
                  }
                  frame True {
                    n1746 = local write "Path SLAB #5"(w1776) -> ()
                  }
                }
              }
            }
          }
          frame #7 {
            n1747 = local read "Ch 07 Status"() -> (w1777:bool)
            n1748 = case shown="True" w1777 {
              frame False {
              }
              frame True {
                n1749 = local read "Folder"() -> (w1779:path)
                n1750 = Build Path(base path=w1779, name or relative path="SLAB7.csv") -> (appended path=w1780:path)
                n1751 = call <vilib>:"Check if File or Folder Exists.vi"("path"=w1780) -> ("file or folder exists?"=w1781:bool, "dup path"=w1782:path)  [unwired: 8 in, 1 out]
                n1752 = case shown="False" w1781 {
                  tunnel: w1782 -> [w1785 w1787]
                  frame False {
                    n1753 = local write "Path SLAB #7"(w1785) -> ()
                    n1754 = call-poly <vilib>:"Write To Spreadsheet File.vi"("delimiter (\\t)"="," ("delimiter (\\t)"), "append to file? (new file:F)"=FALSE, "1D data"=string[] ["Timestamp", "Measured", "Calibrated"], "file path (dialog if empty)"=w1785) -> ()  [unwired: 3 in, 2 out]
                  }
                  frame True {
                    n1755 = local write "Path SLAB #7"(w1787) -> ()
                  }
                }
              }
            }
          }
          frame #8 {
            n1756 = local read "Ch 10 Status"() -> (w1788:bool)
            n1757 = case shown="True" w1788 {
              frame False {
              }
              frame True {
                n1758 = local read "Folder"() -> (w1790:path)
                n1759 = Build Path(base path=w1790, name or relative path="SLAB8.csv") -> (appended path=w1791:path)
                n1760 = call <vilib>:"Check if File or Folder Exists.vi"("path"=w1791) -> ("file or folder exists?"=w1792:bool, "dup path"=w1793:path)  [unwired: 8 in, 1 out]
                n1761 = case shown="False" w1792 {
                  tunnel: w1793 -> [w1796 w1798]
                  frame False {
                    n1762 = local write "Path SLAB #8"(w1796) -> ()
                    n1763 = call-poly <vilib>:"Write To Spreadsheet File.vi"("delimiter (\\t)"="," ("delimiter (\\t)"), "append to file? (new file:F)"=FALSE, "1D data"=string[] ["Timestamp", "Measured", "Calibrated"], "file path (dialog if empty)"=w1796) -> ()  [unwired: 3 in, 2 out]
                  }
                  frame True {
                    n1764 = local write "Path SLAB #8"(w1798) -> ()
                  }
                }
              }
            }
          }
          frame #9 {
            n1765 = local read "Ch 08 Status"() -> (w1799:bool)
            n1766 = case shown="True" w1799 {
              frame False {
              }
              frame True {
                n1767 = local read "Folder"() -> (w1801:path)
                n1768 = Build Path(base path=w1801, name or relative path="SLAB9.csv") -> (appended path=w1802:path)
                n1769 = call <vilib>:"Check if File or Folder Exists.vi"("path"=w1802) -> ("file or folder exists?"=w1803:bool, "dup path"=w1804:path)  [unwired: 8 in, 1 out]
                n1770 = case shown="False" w1803 {
                  tunnel: w1804 -> [w1807 w1809]
                  frame False {
                    n1771 = local write "Path SLAB #9"(w1807) -> ()
                    n1772 = call-poly <vilib>:"Write To Spreadsheet File.vi"("delimiter (\\t)"="," ("delimiter (\\t)"), "append to file? (new file:F)"=FALSE, "1D data"=string[] ["Timestamp", "Measured", "Calibrated"], "file path (dialog if empty)"=w1807) -> ()  [unwired: 3 in, 2 out]
                  }
                  frame True {
                    n1773 = local write "Path SLAB #9"(w1809) -> ()
                  }
                }
              }
            }
          }
          frame #10 {
            n1774 = local read "Ch 09 Status"() -> (w1810:bool)
            n1775 = case shown="True" w1810 {
              frame False {
              }
              frame True {
                n1776 = local read "Folder"() -> (w1812:path)
                n1777 = Build Path(base path=w1812, name or relative path="SLAB10.csv") -> (appended path=w1813:path)
                n1778 = call <vilib>:"Check if File or Folder Exists.vi"("path"=w1813) -> ("file or folder exists?"=w1814:bool, "dup path"=w1815:path)  [unwired: 8 in, 1 out]
                n1779 = case shown="False" w1814 {
                  tunnel: w1815 -> [w1818 w1820]
                  frame False {
                    n1780 = local write "Path SLAB #10"(w1818) -> ()
                    n1781 = call-poly <vilib>:"Write To Spreadsheet File.vi"("delimiter (\\t)"="," ("delimiter (\\t)"), "append to file? (new file:F)"=FALSE, "1D data"=string[] ["Timestamp", "Measured", "Calibrated"], "file path (dialog if empty)"=w1818) -> ()  [unwired: 3 in, 2 out]
                  }
                  frame True {
                    n1782 = local write "Path SLAB #10"(w1820) -> ()
                  }
                }
              }
            }
          }
          frame #11 {
            n1783 = local read "Ch 14 Status"() -> (w1821:bool)
            n1784 = case shown="True" w1821 {
              frame False {
              }
              frame True {
                n1785 = local read "Folder"() -> (w1826:path)
                n1786 = Build Path(base path=w1826, name or relative path="1st_stage.csv") -> (appended path=w1825:path)
                n1787 = call <vilib>:"Check if File or Folder Exists.vi"("path"=w1825) -> ("file or folder exists?"=w1824:bool, "dup path"=w1823:path)  [unwired: 8 in, 1 out]
                n1788 = case shown="False" w1824 {
                  tunnel: w1823 -> [w1829 w1831]
                  frame False {
                    n1789 = local write "Path 1st stage"(w1829) -> ()
                    n1790 = call-poly <vilib>:"Write To Spreadsheet File.vi"("delimiter (\\t)"="," ("delimiter (\\t)"), "append to file? (new file:F)"=FALSE, "1D data"=string[] ["Timestamp", "Measured", "Calibrated"], "file path (dialog if empty)"=w1829) -> ()  [unwired: 3 in, 2 out]
                  }
                  frame True {
                    n1791 = local write "Path 1st stage"(w1831) -> ()
                  }
                }
              }
            }
          }
          frame #12 {
            n1792 = local read "Ch 11 Status"() -> (w1832:bool)
            n1793 = case shown="True" w1832 {
              frame False {
              }
              frame True {
                n1794 = local read "Folder"() -> (w1837:path)
                n1795 = Build Path(base path=w1837, name or relative path="2nd_stage.csv") -> (appended path=w1836:path)
                n1796 = call <vilib>:"Check if File or Folder Exists.vi"("path"=w1836) -> ("file or folder exists?"=w1835:bool, "dup path"=w1834:path)  [unwired: 8 in, 1 out]
                n1797 = case shown="False" w1835 {
                  tunnel: w1834 -> [w1840 w1842]
                  frame False {
                    n1798 = local write "Path 2nd stage"(w1840) -> ()
                    n1799 = call-poly <vilib>:"Write To Spreadsheet File.vi"("delimiter (\\t)"="," ("delimiter (\\t)"), "append to file? (new file:F)"=FALSE, "1D data"=string[] ["Timestamp", "Measured", "Calibrated"], "file path (dialog if empty)"=w1840) -> ()  [unwired: 3 in, 2 out]
                  }
                  frame True {
                    n1800 = local write "Path 2nd stage"(w1842) -> ()
                  }
                }
              }
            }
          }
          frame #13 {
            n1801 = local read "Ch 12 Status"() -> (w1843:bool)
            n1802 = case shown="True" w1843 {
              frame False {
              }
              frame True {
                n1803 = local read "Folder"() -> (w1848:path)
                n1804 = Build Path(base path=w1848, name or relative path="3rd_stage.csv") -> (appended path=w1847:path)
                n1805 = call <vilib>:"Check if File or Folder Exists.vi"("path"=w1847) -> ("file or folder exists?"=w1846:bool, "dup path"=w1845:path)  [unwired: 8 in, 1 out]
                n1806 = case shown="False" w1846 {
                  tunnel: w1845 -> [w1851 w1853]
                  frame False {
                    n1807 = local write "Path 3rd stage"(w1851) -> ()
                    n1808 = call-poly <vilib>:"Write To Spreadsheet File.vi"("delimiter (\\t)"="," ("delimiter (\\t)"), "append to file? (new file:F)"=FALSE, "1D data"=string[] ["Timestamp", "Measured", "Calibrated"], "file path (dialog if empty)"=w1851) -> ()  [unwired: 3 in, 2 out]
                  }
                  frame True {
                    n1809 = local write "Path 3rd stage"(w1853) -> ()
                  }
                }
              }
            }
          }
          frame #14 {
            n1810 = local read "Ch 15 Status"() -> (w1854:bool)
            n1811 = case shown="True" w1854 {
              frame False {
              }
              frame True {
                n1812 = local read "Folder"() -> (w1859:path)
                n1813 = Build Path(base path=w1859, name or relative path="4th_stage.csv") -> (appended path=w1858:path)
                n1814 = call <vilib>:"Check if File or Folder Exists.vi"("path"=w1858) -> ("file or folder exists?"=w1857:bool, "dup path"=w1856:path)  [unwired: 8 in, 1 out]
                n1815 = case shown="False" w1857 {
                  tunnel: w1856 -> [w1862 w1864]
                  frame False {
                    n1816 = local write "Path 4th stage"(w1862) -> ()
                    n1817 = call-poly <vilib>:"Write To Spreadsheet File.vi"("delimiter (\\t)"="," ("delimiter (\\t)"), "append to file? (new file:F)"=FALSE, "1D data"=string[] ["Timestamp", "Measured", "Calibrated"], "file path (dialog if empty)"=w1862) -> ()  [unwired: 3 in, 2 out]
                  }
                  frame True {
                    n1818 = local write "Path 4th stage"(w1864) -> ()
                  }
                }
              }
            }
          }
          frame #15 {
            n1819 = local read "Ch 16 Status"() -> (w1865:bool)
            n1820 = case shown="True" w1865 {
              frame False {
              }
              frame True {
                n1821 = local read "Folder"() -> (w1870:path)
                n1822 = Build Path(base path=w1870, name or relative path="5th_stage.csv") -> (appended path=w1869:path)
                n1823 = call <vilib>:"Check if File or Folder Exists.vi"("path"=w1869) -> ("file or folder exists?"=w1868:bool, "dup path"=w1867:path)  [unwired: 8 in, 1 out]
                n1824 = case shown="False" w1868 {
                  tunnel: w1867 -> [w1873 w1875]
                  frame False {
                    n1825 = local write "Path 5th stage"(w1873) -> ()
                    n1826 = call-poly <vilib>:"Write To Spreadsheet File.vi"("delimiter (\\t)"="," ("delimiter (\\t)"), "append to file? (new file:F)"=FALSE, "1D data"=string[] ["Timestamp", "Measured", "Calibrated"], "file path (dialog if empty)"=w1873) -> ()  [unwired: 3 in, 2 out]
                  }
                  frame True {
                    n1827 = local write "Path 5th stage"(w1875) -> ()
                  }
                }
              }
            }
          }
          frame #16 {
            n1828 = local read "Ch 13 Status"() -> (w1876:bool)
            n1829 = case shown="True" w1876 {
              frame False {
              }
              frame True {
                n1830 = local read "Folder"() -> (w1881:path)
                n1831 = Build Path(base path=w1881, name or relative path="quanta-ray.csv") -> (appended path=w1880:path)
                n1832 = call <vilib>:"Check if File or Folder Exists.vi"("path"=w1880) -> ("file or folder exists?"=w1879:bool, "dup path"=w1878:path)  [unwired: 8 in, 1 out]
                n1833 = case shown="False" w1879 {
                  tunnel: w1878 -> [w1884 w1886]
                  frame False {
                    n1834 = local write "Path quanta ray"(w1884) -> ()
                    n1835 = call-poly <vilib>:"Write To Spreadsheet File.vi"("delimiter (\\t)"="," ("delimiter (\\t)"), "append to file? (new file:F)"=FALSE, "1D data"=string[] ["Timestamp", "Measured", "Calibrated"], "file path (dialog if empty)"=w1884) -> ()  [unwired: 3 in, 2 out]
                  }
                  frame True {
                    n1836 = local write "Path quanta ray"(w1886) -> ()
                  }
                }
              }
            }
          }
        }
      }
      frame True {
        # "Do nothing if date didn't change"
      }
    }
    n1837 = local read "Com Port 1"() -> (w967:refnum<visa-resource-name>)
    n1838 = local read "Com Port 1"() -> (w965:refnum<visa-resource-name>)
    n1839 = local read "Com Port 7"() -> (w901:refnum<visa-resource-name>)
    n1840 = local read "Com Port 7"() -> (w899:refnum<visa-resource-name>)
    n1841 = local read "Com Port 5"() -> (w922:refnum<visa-resource-name>)
    n1842 = local read "Com Port 5"() -> (w924:refnum<visa-resource-name>)
    n1843 = local read "Com Port 3"() -> (w947:refnum<visa-resource-name>)
    n1844 = local read "Com Port 3"() -> (w945:refnum<visa-resource-name>)
    n1845 = case shown="False" "Scale Down 2" {
      tunnel: w967 -> [_ w2251]
      frame False {
      }
      frame True {
        # "If clicked, stop slink reading(*CS1 and *CS2),\nsend scale down ch2 to slink, and read ch2 status"
        n1846 = stacked-sequence {
          tunnel: w2251 -> [w2253 w2256 w2260]
          tunnel: [w2253 _ _] -> w2250
          frame #0 {
            w2255 = 10 items=["*RST", "*PWC", "*CA1", "*CA2", "*SS1001", "*SS2001", "*SU1", "*SU2", "*SD1", "*SD2", "*CS1", "*CS2"] ("string to write")
            n1847 = call "Send.vi"("string to write"=w2255, "port number"=w2253) -> ()  [unwired: 1 in]
            n1848 = Wait (ms)(milliseconds to wait=10) -> ()  [unwired: 1 out]
          }
          frame #1 {
            w2258 = 11 items=["*RST", "*PWC", "*CA1", "*CA2", "*SS1001", "*SS2001", "*SU1", "*SU2", "*SD1", "*SD2", "*CS1", "*CS2"] ("string to write")
            n1849 = call "Send.vi"("string to write"=w2258, "port number"=w2256) -> ()  [unwired: 1 in]
            n1850 = Wait (ms)(milliseconds to wait=10) -> ()  [unwired: 1 out]
          }
          frame #2 {
            w2261 = 8 items=["*RST", "*PWC", "*CA1", "*CA2", "*SS1001", "*SS2001", "*SU1", "*SU2", "*SD1", "*SD2"] ("string to write")
            n1851 = call "Send.vi"("string to write"=w2261, "port number"=w2260) -> ()  [unwired: 1 in]
            n1852 = Wait (ms)(milliseconds to wait=10) -> ()  [unwired: 1 out]
          }
        }
        n1853 = local write "Scale Down 2"(FALSE) -> ()
        n1854 = local read "Ch 01 Status"() -> (w2249:bool)
        n1855 = local read "Ch 02 Status"() -> (w2247:bool)
        n1856 = call "Read Scale Ch 1.vi"("Ch2"=w2247, "Com Port"=w2250, "Ch 1"=w2249) -> ("Scale 1Ch"=w2248:dbl)  [unwired: 2 out]
        n1857 = local write "Scale 2"(w2248) -> ()
      }
    }
    n1858 = case shown="True" "Scale Down" {
      tunnel: w965 -> [_ w2236]
      frame False {
      }
      frame True {
        # "If clicked, stop slink reading(*CS1 and *CS2),\nsend scale down ch1 to slink, and read ch1 status"
        n1859 = stacked-sequence {
          tunnel: w2236 -> [w2238 w2241 w2245]
          tunnel: [w2238 _ _] -> w2235
          frame #0 {
            w2240 = 10 items=["*RST", "*PWC", "*CA1", "*CA2", "*SS1001", "*SS2001", "*SU1", "*SU2", "*SD1", "*SD2", "*CS1", "*CS2"] ("string to write")
            n1860 = call "Send.vi"("string to write"=w2240, "port number"=w2238) -> ()  [unwired: 1 in]
            n1861 = Wait (ms)(milliseconds to wait=10) -> ()  [unwired: 1 out]
          }
          frame #1 {
            w2243 = 11 items=["*RST", "*PWC", "*CA1", "*CA2", "*SS1001", "*SS2001", "*SU1", "*SU2", "*SD1", "*SD2", "*CS1", "*CS2"] ("string to write")
            n1862 = call "Send.vi"("string to write"=w2243, "port number"=w2241) -> ()  [unwired: 1 in]
            n1863 = Wait (ms)(milliseconds to wait=10) -> ()  [unwired: 1 out]
          }
          frame #2 {
            w2246 = 9 items=["*RST", "*PWC", "*CA1", "*CA2", "*SS1001", "*SS2001", "*SU1", "*SU2", "*SD1", "*SD2"] ("string to write")
            n1864 = call "Send.vi"("string to write"=w2246, "port number"=w2245) -> ()  [unwired: 1 in]
            n1865 = Wait (ms)(milliseconds to wait=10) -> ()  [unwired: 1 out]
          }
        }
        n1866 = local write "Scale Down"(FALSE) -> ()
        n1867 = local read "Ch 01 Status"() -> (w2233:bool)
        n1868 = local read "Ch 02 Status"() -> (w2232:bool)
        n1869 = call "Read Scale Ch 2.vi"("Ch 2"=w2232, "Com Port"=w2235, "Ch1"=w2233) -> ("Scale Ch2"=w2234:dbl)  [unwired: 2 out]
        n1870 = local write "Scale 1"(w2234) -> ()
      }
    }
    n1871 = case shown="False" "Scale Down 13" {
      tunnel: w901 -> [_ w1595]
      frame False {
      }
      frame True {
        n1872 = stacked-sequence {
          tunnel: w1595 -> [w1597 w1600 w1604]
          tunnel: [w1597 _ _] -> w1594
          frame #0 {
            w1599 = 10 items=["*RST", "*PWC", "*CA1", "*CA2", "*SS1001", "*SS2001", "*SU1", "*SU2", "*SD1", "*SD2", "*CS1", "*CS2"] ("string to write")
            n1873 = call "Send.vi"("string to write"=w1599, "port number"=w1597) -> ()  [unwired: 1 in]
            n1874 = Wait (ms)(milliseconds to wait=10) -> ()  [unwired: 1 out]
          }
          frame #1 {
            w1602 = 11 items=["*RST", "*PWC", "*CA1", "*CA2", "*SS1001", "*SS2001", "*SU1", "*SU2", "*SD1", "*SD2", "*CS1", "*CS2"] ("string to write")
            n1875 = call "Send.vi"("string to write"=w1602, "port number"=w1600) -> ()  [unwired: 1 in]
            n1876 = Wait (ms)(milliseconds to wait=10) -> ()  [unwired: 1 out]
          }
          frame #2 {
            w1605 = 8 items=["*RST", "*PWC", "*CA1", "*CA2", "*SS1001", "*SS2001", "*SU1", "*SU2", "*SD1", "*SD2"] ("string to write")
            n1877 = call "Send.vi"("string to write"=w1605, "port number"=w1604) -> ()  [unwired: 1 in]
            n1878 = Wait (ms)(milliseconds to wait=10) -> ()  [unwired: 1 out]
          }
        }
        n1879 = local write "Scale Down 13"(FALSE) -> ()
        n1880 = local read "Ch 13 Status"() -> (w1593:bool)
        n1881 = local read "Ch 14 Status"() -> (w1591:bool)
        n1882 = call "Read Scale Ch 1.vi"("Ch2"=w1591, "Com Port"=w1594, "Ch 1"=w1593) -> ("Scale 1Ch"=w1592:dbl)  [unwired: 2 out]
        n1883 = local write "Scale 13"(w1592) -> ()
      }
    }
    n1884 = case shown="False" "Scale Down 14" {
      tunnel: w899 -> [_ w1580]
      frame False {
      }
      frame True {
        n1885 = stacked-sequence {
          tunnel: w1580 -> [w1582 w1585 w1589]
          tunnel: [w1582 _ _] -> w1579
          frame #0 {
            w1584 = 10 items=["*RST", "*PWC", "*CA1", "*CA2", "*SS1001", "*SS2001", "*SU1", "*SU2", "*SD1", "*SD2", "*CS1", "*CS2"] ("string to write")
            n1886 = call "Send.vi"("string to write"=w1584, "port number"=w1582) -> ()  [unwired: 1 in]
            n1887 = Wait (ms)(milliseconds to wait=10) -> ()  [unwired: 1 out]
          }
          frame #1 {
            w1587 = 11 items=["*RST", "*PWC", "*CA1", "*CA2", "*SS1001", "*SS2001", "*SU1", "*SU2", "*SD1", "*SD2", "*CS1", "*CS2"] ("string to write")
            n1888 = call "Send.vi"("string to write"=w1587, "port number"=w1585) -> ()  [unwired: 1 in]
            n1889 = Wait (ms)(milliseconds to wait=10) -> ()  [unwired: 1 out]
          }
          frame #2 {
            w1590 = 9 items=["*RST", "*PWC", "*CA1", "*CA2", "*SS1001", "*SS2001", "*SU1", "*SU2", "*SD1", "*SD2"] ("string to write")
            n1890 = call "Send.vi"("string to write"=w1590, "port number"=w1589) -> ()  [unwired: 1 in]
            n1891 = Wait (ms)(milliseconds to wait=10) -> ()  [unwired: 1 out]
          }
        }
        n1892 = local write "Scale Down 14"(FALSE) -> ()
        n1893 = local read "Ch 13 Status"() -> (w1577:bool)
        n1894 = local read "Ch 14 Status"() -> (w1576:bool)
        n1895 = call "Read Scale Ch 2.vi"("Ch 2"=w1576, "Com Port"=w1579, "Ch1"=w1577) -> ("Scale Ch2"=w1578:dbl)  [unwired: 2 out]
        n1896 = local write "Scale 14"(w1578) -> ()
      }
    }
    n1897 = case shown="False" "Scale Down 9" {
      tunnel: w922 -> [_ w1939]
      frame False {
      }
      frame True {
        n1898 = stacked-sequence {
          tunnel: w1939 -> [w1941 w1944 w1948]
          tunnel: [w1941 _ _] -> w1938
          frame #0 {
            w1943 = 10 items=["*RST", "*PWC", "*CA1", "*CA2", "*SS1001", "*SS2001", "*SU1", "*SU2", "*SD1", "*SD2", "*CS1", "*CS2"] ("string to write")
            n1899 = call "Send.vi"("string to write"=w1943, "port number"=w1941) -> ()  [unwired: 1 in]
            n1900 = Wait (ms)(milliseconds to wait=10) -> ()  [unwired: 1 out]
          }
          frame #1 {
            w1946 = 11 items=["*RST", "*PWC", "*CA1", "*CA2", "*SS1001", "*SS2001", "*SU1", "*SU2", "*SD1", "*SD2", "*CS1", "*CS2"] ("string to write")
            n1901 = call "Send.vi"("string to write"=w1946, "port number"=w1944) -> ()  [unwired: 1 in]
            n1902 = Wait (ms)(milliseconds to wait=10) -> ()  [unwired: 1 out]
          }
          frame #2 {
            w1949 = 8 items=["*RST", "*PWC", "*CA1", "*CA2", "*SS1001", "*SS2001", "*SU1", "*SU2", "*SD1", "*SD2"] ("string to write")
            n1903 = call "Send.vi"("string to write"=w1949, "port number"=w1948) -> ()  [unwired: 1 in]
            n1904 = Wait (ms)(milliseconds to wait=10) -> ()  [unwired: 1 out]
          }
        }
        n1905 = local write "Scale Down 9"(FALSE) -> ()
        n1906 = local read "Ch 09 Status"() -> (w1937:bool)
        n1907 = local read "Ch 10 Status"() -> (w1936:bool)
        n1908 = call "Read Scale Ch 1.vi"("Ch2"=w1936, "Com Port"=w1938, "Ch 1"=w1937) -> ("Scale 1Ch"=w1935:dbl)  [unwired: 2 out]
        n1909 = local write "Scale 9"(w1935) -> ()
      }
    }
    n1910 = case shown="False" "Scale Down 5" {
      tunnel: w947 -> [_ w2095]
      frame False {
      }
      frame True {
        n1911 = stacked-sequence {
          tunnel: w2095 -> [w2097 w2100 w2104]
          tunnel: [w2097 _ _] -> w2094
          frame #0 {
            w2099 = 10 items=["*RST", "*PWC", "*CA1", "*CA2", "*SS1001", "*SS2001", "*SU1", "*SU2", "*SD1", "*SD2", "*CS1", "*CS2"] ("string to write")
            n1912 = call "Send.vi"("string to write"=w2099, "port number"=w2097) -> ()  [unwired: 1 in]
            n1913 = Wait (ms)(milliseconds to wait=10) -> ()  [unwired: 1 out]
          }
          frame #1 {
            w2102 = 11 items=["*RST", "*PWC", "*CA1", "*CA2", "*SS1001", "*SS2001", "*SU1", "*SU2", "*SD1", "*SD2", "*CS1", "*CS2"] ("string to write")
            n1914 = call "Send.vi"("string to write"=w2102, "port number"=w2100) -> ()  [unwired: 1 in]
            n1915 = Wait (ms)(milliseconds to wait=10) -> ()  [unwired: 1 out]
          }
          frame #2 {
            w2105 = 8 items=["*RST", "*PWC", "*CA1", "*CA2", "*SS1001", "*SS2001", "*SU1", "*SU2", "*SD1", "*SD2"] ("string to write")
            n1916 = call "Send.vi"("string to write"=w2105, "port number"=w2104) -> ()  [unwired: 1 in]
            n1917 = Wait (ms)(milliseconds to wait=10) -> ()  [unwired: 1 out]
          }
        }
        n1918 = local write "Scale Down 5"(FALSE) -> ()
        n1919 = local read "Ch 05 Status"() -> (w2093:bool)
        n1920 = local read "Ch 06 Status"() -> (w2091:bool)
        n1921 = call "Read Scale Ch 1.vi"("Ch2"=w2091, "Com Port"=w2094, "Ch 1"=w2093) -> ("Scale 1Ch"=w2092:dbl)  [unwired: 2 out]
        n1922 = local write "Scale 5"(w2092) -> ()
      }
    }
    n1923 = case shown="False" "Scale Down 10" {
      tunnel: w924 -> [_ w1924]
      frame False {
      }
      frame True {
        n1924 = stacked-sequence {
          tunnel: w1924 -> [w1926 w1929 w1933]
          tunnel: [w1926 _ _] -> w1923
          frame #0 {
            w1928 = 10 items=["*RST", "*PWC", "*CA1", "*CA2", "*SS1001", "*SS2001", "*SU1", "*SU2", "*SD1", "*SD2", "*CS1", "*CS2"] ("string to write")
            n1925 = call "Send.vi"("string to write"=w1928, "port number"=w1926) -> ()  [unwired: 1 in]
            n1926 = Wait (ms)(milliseconds to wait=10) -> ()  [unwired: 1 out]
          }
          frame #1 {
            w1931 = 11 items=["*RST", "*PWC", "*CA1", "*CA2", "*SS1001", "*SS2001", "*SU1", "*SU2", "*SD1", "*SD2", "*CS1", "*CS2"] ("string to write")
            n1927 = call "Send.vi"("string to write"=w1931, "port number"=w1929) -> ()  [unwired: 1 in]
            n1928 = Wait (ms)(milliseconds to wait=10) -> ()  [unwired: 1 out]
          }
          frame #2 {
            w1934 = 9 items=["*RST", "*PWC", "*CA1", "*CA2", "*SS1001", "*SS2001", "*SU1", "*SU2", "*SD1", "*SD2"] ("string to write")
            n1929 = call "Send.vi"("string to write"=w1934, "port number"=w1933) -> ()  [unwired: 1 in]
            n1930 = Wait (ms)(milliseconds to wait=10) -> ()  [unwired: 1 out]
          }
        }
        n1931 = local write "Scale Down 10"(FALSE) -> ()
        n1932 = local read "Ch 09 Status"() -> (w1920:bool)
        n1933 = local read "Ch 10 Status"() -> (w1921:bool)
        n1934 = call "Read Scale Ch 2.vi"("Ch 2"=w1921, "Com Port"=w1923, "Ch1"=w1920) -> ("Scale Ch2"=w1922:dbl)  [unwired: 2 out]
        n1935 = local write "Scale 10"(w1922) -> ()
      }
    }
    n1936 = case shown="False" "Scale Down 6" {
      tunnel: w945 -> [_ w2080]
      frame False {
      }
      frame True {
        n1937 = stacked-sequence {
          tunnel: w2080 -> [w2082 w2085 w2089]
          tunnel: [w2082 _ _] -> w2079
          frame #0 {
            w2084 = 10 items=["*RST", "*PWC", "*CA1", "*CA2", "*SS1001", "*SS2001", "*SU1", "*SU2", "*SD1", "*SD2", "*CS1", "*CS2"] ("string to write")
            n1938 = call "Send.vi"("string to write"=w2084, "port number"=w2082) -> ()  [unwired: 1 in]
            n1939 = Wait (ms)(milliseconds to wait=10) -> ()  [unwired: 1 out]
          }
          frame #1 {
            w2087 = 11 items=["*RST", "*PWC", "*CA1", "*CA2", "*SS1001", "*SS2001", "*SU1", "*SU2", "*SD1", "*SD2", "*CS1", "*CS2"] ("string to write")
            n1940 = call "Send.vi"("string to write"=w2087, "port number"=w2085) -> ()  [unwired: 1 in]
            n1941 = Wait (ms)(milliseconds to wait=10) -> ()  [unwired: 1 out]
          }
          frame #2 {
            w2090 = 9 items=["*RST", "*PWC", "*CA1", "*CA2", "*SS1001", "*SS2001", "*SU1", "*SU2", "*SD1", "*SD2"] ("string to write")
            n1942 = call "Send.vi"("string to write"=w2090, "port number"=w2089) -> ()  [unwired: 1 in]
            n1943 = Wait (ms)(milliseconds to wait=10) -> ()  [unwired: 1 out]
          }
        }
        n1944 = local write "Scale Down 6"(FALSE) -> ()
        n1945 = local read "Ch 05 Status"() -> (w2077:bool)
        n1946 = local read "Ch 06 Status"() -> (w2076:bool)
        n1947 = call "Read Scale Ch 2.vi"("Ch 2"=w2076, "Com Port"=w2079, "Ch1"=w2077) -> ("Scale Ch2"=w2078:dbl)  [unwired: 2 out]
        n1948 = local write "Scale 6"(w2078) -> ()
      }
    }
    n1949 = local read "Com Port 1"() -> (w961:refnum<visa-resource-name>)
    n1950 = local read "Com Port 7"() -> (w895:refnum<visa-resource-name>)
    n1951 = local read "Com Port 5"() -> (w928:refnum<visa-resource-name>)
    n1952 = local read "Com Port 3"() -> (w941:refnum<visa-resource-name>)
    n1953 = case shown="True" "Send" {
      tunnel: w961 -> [_ w2199]
      frame False {
      }
      frame True {
        n1954 = stacked-sequence {
          tunnel: w2199 -> [w2204 w2209 w2212]
          frame #0 {
            # "send command"
            n1955 = local read "Option"() -> (w2202:string)
            n1956 = local read "Command"() -> (w2201:i32)
            n1957 = call "Send.vi"("string to write"=w2201, "port number"=w2204, "Option"=w2202) -> ()
            n1958 = Wait (ms)(milliseconds to wait=10) -> ()  [unwired: 1 out]
          }
          frame #1 {
            # "read ch1 status"
            n1959 = local read "Ch 02 Status"() -> (w2207:bool)
            n1960 = local read "Ch 01 Status"() -> (w2208:bool)
            n1961 = call "Read Scale Ch 1.vi"("Ch2"=w2207, "Com Port"=w2209, "Ch 1"=w2208) -> ("Scale 1Ch"=w2206:dbl, "Trigger Status Ch1"=w2205:bool, "Wavelength"=w2210:u32)
            n1962 = local write "Trigger ch 1"(w2205) -> ()
            n1963 = local write "Wavelength 1"(w2210) -> ()
            n1964 = local write "Scale 1"(w2206) -> ()
          }
          frame #2 {
            # "read ch2 status"
            n1965 = local read "Ch 01 Status"() -> (w2214:bool)
            n1966 = local read "Ch 02 Status"() -> (w2215:bool)
            n1967 = call "Read Scale Ch 2.vi"("Ch 2"=w2215, "Com Port"=w2212, "Ch1"=w2214) -> ("Scale Ch2"=w2213:dbl, "External Trigger Ch2"=w2211:bool, "Wavelength"=w2216:u32)
            n1968 = local write "Trigger ch 2"(w2211) -> ()
            n1969 = local write "Wavelength 2"(w2216) -> ()
            n1970 = local write "Scale 2"(w2213) -> ()
          }
        }
        n1971 = local write "Send"(FALSE) -> ()
      }
    }
    n1972 = case shown="True" "Send 7" {
      tunnel: w895 -> [_ w1543]
      frame False {
      }
      frame True {
        n1973 = stacked-sequence {
          tunnel: w1543 -> [w1548 w1554 w1560]
          frame #0 {
            n1974 = local read "Option"() -> (w1546:string)
            n1975 = local read "Command"() -> (w1545:i32)
            n1976 = call "Send.vi"("string to write"=w1545, "port number"=w1548, "Option"=w1546) -> ()
            n1977 = Wait (ms)(milliseconds to wait=10) -> ()  [unwired: 1 out]
          }
          frame #1 {
            n1978 = local read "Ch 13 Status"() -> (w1551:bool)
            n1979 = local read "Ch 14 Status"() -> (w1550:bool)
            n1980 = call "Read Scale Ch 1.vi"("Ch2"=w1550, "Com Port"=w1554, "Ch 1"=w1551) -> ("Scale 1Ch"=w1553:dbl, "Trigger Status Ch1"=w1552:bool, "Wavelength"=w1549:u32)
            n1981 = local write "Trigger ch 13"(w1552) -> ()
            n1982 = local write "Wavelength 13"(w1549) -> ()
            n1983 = local write "Scale 13"(w1553) -> ()
          }
          frame #2 {
            n1984 = local read "Ch 13 Status"() -> (w1555:bool)
            n1985 = local read "Ch 14 Status"() -> (w1557:bool)
            n1986 = call "Read Scale Ch 2.vi"("Ch 2"=w1557, "Com Port"=w1560, "Ch1"=w1555) -> ("Scale Ch2"=w1558:dbl, "External Trigger Ch2"=w1556:bool, "Wavelength"=w1559:u32)
            n1987 = local write "Wavelength 14"(w1559) -> ()
            n1988 = local write "Trigger ch 14"(w1556) -> ()
            n1989 = local write "Scale 14"(w1558) -> ()
          }
        }
        n1990 = local write "Send 7"(FALSE) -> ()
      }
    }
    n1991 = case shown="True" "Send 5" {
      tunnel: w928 -> [_ w1887]
      frame False {
      }
      frame True {
        n1992 = stacked-sequence {
          tunnel: w1887 -> [w1892 w1897 w1902]
          frame #0 {
            n1993 = local read "Option"() -> (w1890:string)
            n1994 = local read "Command"() -> (w1889:i32)
            n1995 = call "Send.vi"("string to write"=w1889, "port number"=w1892, "Option"=w1890) -> ()
            n1996 = Wait (ms)(milliseconds to wait=10) -> ()  [unwired: 1 out]
          }
          frame #1 {
            n1997 = local read "Ch 09 Status"() -> (w1896:bool)
            n1998 = local read "Ch 10 Status"() -> (w1894:bool)
            n1999 = call "Read Scale Ch 1.vi"("Ch2"=w1894, "Com Port"=w1897, "Ch 1"=w1896) -> ("Scale 1Ch"=w1895:dbl, "Trigger Status Ch1"=w1893:bool, "Wavelength"=w1898:u32)
            n2000 = local write "Wavelength 9"(w1898) -> ()
            n2001 = local write "Trigger ch 9"(w1893) -> ()
            n2002 = local write "Scale 9"(w1895) -> ()
          }
          frame #2 {
            n2003 = local read "Ch 09 Status"() -> (w1901:bool)
            n2004 = local read "Ch 10 Status"() -> (w1900:bool)
            n2005 = call "Read Scale Ch 2.vi"("Ch 2"=w1900, "Com Port"=w1902, "Ch1"=w1901) -> ("Scale Ch2"=w1903:dbl, "External Trigger Ch2"=w1899:bool, "Wavelength"=w1904:u32)
            n2006 = local write "Wavelength 10"(w1904) -> ()
            n2007 = local write "Trigger ch 10"(w1899) -> ()
            n2008 = local write "Scale 10"(w1903) -> ()
          }
        }
        n2009 = local write "Send 5"(FALSE) -> ()
      }
    }
    n2010 = case shown="True" "Send 3" {
      tunnel: w941 -> [_ w2043]
      frame False {
      }
      frame True {
        n2011 = stacked-sequence {
          tunnel: w2043 -> [w2048 w2053 w2056]
          frame #0 {
            n2012 = local read "Option"() -> (w2046:string)
            n2013 = local read "Command"() -> (w2045:i32)
            n2014 = call "Send.vi"("string to write"=w2045, "port number"=w2048, "Option"=w2046) -> ()
            n2015 = Wait (ms)(milliseconds to wait=10) -> ()  [unwired: 1 out]
          }
          frame #1 {
            n2016 = local read "Ch 06 Status"() -> (w2050:bool)
            n2017 = local read "Ch 05 Status"() -> (w2052:bool)
            n2018 = call "Read Scale Ch 1.vi"("Ch2"=w2050, "Com Port"=w2053, "Ch 1"=w2052) -> ("Scale 1Ch"=w2051:dbl, "Trigger Status Ch1"=w2049:bool, "Wavelength"=w2054:u32)
            n2019 = local write "Wavelength 5"(w2054) -> ()
            n2020 = local write "Scale 5"(w2051) -> ()
            n2021 = local write "Trigger ch 5"(w2049) -> ()
          }
          frame #2 {
            n2022 = local read "Ch 05 Status"() -> (w2058:bool)
            n2023 = local read "Ch 06 Status"() -> (w2059:bool)
            n2024 = call "Read Scale Ch 2.vi"("Ch 2"=w2059, "Com Port"=w2056, "Ch1"=w2058) -> ("Scale Ch2"=w2057:dbl, "External Trigger Ch2"=w2055:bool, "Wavelength"=w2060:u32)
            n2025 = local write "Trigger ch 6"(w2055) -> ()
            n2026 = local write "Wavelength 6"(w2060) -> ()
            n2027 = local write "Scale 6"(w2057) -> ()
          }
        }
        n2028 = local write "Send 3"(FALSE) -> ()
      }
    }
  }
  n2029 = stacked-sequence {
    tunnel: w15 -> [w2278 _ _ _ _ _ _ _]
    tunnel: w7 -> [_ w2281 _ _ _ _ _ _]
    tunnel: w6 -> [_ _ w2283 _ _ _ _ _]
    tunnel: w5 -> [_ _ _ w2285 _ _ _ _]
    tunnel: w4 -> [_ _ _ _ w2287 _ _ _]
    tunnel: w3 -> [_ _ _ _ _ w2289 _ _]
    tunnel: w2 -> [_ _ _ _ _ _ w2291 _]
    tunnel: w1 -> [_ _ _ _ _ _ _ w2293]
    frame #0 {
      w2279 = FALSE
      # "Close com port, and turn off Channel indicator"
      n2030 = local write "Ch 01 Status"(w2279) -> ()
      n2031 = local write "Ch 02 Status"(w2279) -> ()
      n2032 = local write "Program Status:"("Program Stopped!" ("Program Status")) -> ()
      n2033 = VISA Close(VISA resource name=w2278) -> ()  [unwired: 1 in, 1 out]
    }
    frame #1 {
      w2280 = FALSE
      n2034 = local write "Ch 03 Status"(w2280) -> ()
      n2035 = local write "Ch 04 Status"(w2280) -> ()
      n2036 = VISA Close(VISA resource name=w2281) -> ()  [unwired: 1 in, 1 out]
    }
    frame #2 {
      w2282 = FALSE
      n2037 = local write "Ch 05 Status"(w2282) -> ()
      n2038 = local write "Ch 06 Status"(w2282) -> ()
      n2039 = VISA Close(VISA resource name=w2283) -> ()  [unwired: 1 in, 1 out]
    }
    frame #3 {
      w2284 = FALSE
      n2040 = local write "Ch 07 Status"(w2284) -> ()
      n2041 = local write "Ch 08 Status"(w2284) -> ()
      n2042 = VISA Close(VISA resource name=w2285) -> ()  [unwired: 1 in, 1 out]
    }
    frame #4 {
      w2286 = FALSE
      n2043 = local write "Ch 10 Status"(w2286) -> ()
      n2044 = local write "Ch 09 Status"(w2286) -> ()
      n2045 = VISA Close(VISA resource name=w2287) -> ()  [unwired: 1 in, 1 out]
    }
    frame #5 {
      w2288 = FALSE
      n2046 = local write "Ch 12 Status"(w2288) -> ()
      n2047 = local write "Ch 11 Status"(w2288) -> ()
      n2048 = VISA Close(VISA resource name=w2289) -> ()  [unwired: 1 in, 1 out]
    }
    frame #6 {
      w2290 = FALSE
      n2049 = local write "Ch 14 Status"(w2290) -> ()
      n2050 = local write "Ch 13 Status"(w2290) -> ()
      n2051 = VISA Close(VISA resource name=w2291) -> ()  [unwired: 1 in, 1 out]
    }
    frame #7 {
      w2292 = FALSE
      n2052 = local write "Ch 16 Status"(w2292) -> ()
      n2053 = local write "Ch 15 Status"(w2292) -> ()
      n2054 = VISA Close(VISA resource name=w2293) -> ()  [unwired: 1 in, 1 out]
    }
  }
